vi "testLoop.vi"() -> ()   [LabVIEW 2018]
uses:
  02.Type Def's/All Motions.ctl
  02.Type Def's/NVH Mode Control 2.0.ctl
  05.UserVI's/type defs/EOL Global Digital Output Control.ctl
  05.UserVI's/type defs/EOL Global Digital Output Cluster Control.ctl
  <vilib>/Instr/_visa.llb/VISA Configure Serial Port (Instr).vi
  02.Type Def's/Pass Fail Control.ctl
  05.UserVI's/type defs/17x AP Data Type.ctl
  05.UserVI's/type defs/17x Audit Motion Data Seq Control.ctl
  02.Type Def's/EOL Motion Database Table.ctl
  02.Type Def's/lvdt name val pair.ctl
  02.Type Def's/NVH Digital Input.ctl
  02.Type Def's/EOL Switch Max Min Check Cluster.ctl
  02.Type Def's/EOL Switch Value Configuration Cluster.ctl
  02.Type Def's/All Switch Configuration Cluster.ctl
  02.Type Def's/station nvh config.ctl
  02.Type Def's/station DO map.ctl
  02.Type Def's/station rs232 port map.ctl
  02.Type Def's/station ethernet address map.ctl
  02.Type Def's/station paths.ctl
  05.UserVI's/type defs/17x Sunshade Limts Seq.ctl
  02.Type Def's/EOL Module Info Control.ctl
  02.Type Def's/EOL Save Module Test Data Control.ctl
  05.UserVI's/type defs/EOL Global Digital Input Control.ctl
  02.Type Def's/station DI map.ctl
  02.Type Def's/Screen Motion Data.ctl
  02.Type Def's/station motion data indicator.ctl
  02.Type Def's/station hmi.ctl
  02.Type Def's/individual station status.ctl
  02.Type Def's/control refs.ctl
  05.UserVI's/Lambda Power/power supply types.ctl
  <vilib>/Platform/dataskt.llb/DataSocket Reference Type.ctl
  05.UserVI's/type defs/plc path and tag.ctl
  02.Type Def's/station plc read boolean tags.ctl
  02.Type Def's/station plc write boolean tags.ctl
  02.Type Def's/station plc read string tags.ctl
  02.Type Def's/station plc write string tags.ctl
  02.Type Def's/iGPS float tags.ctl
  02.Type Def's/station plc read float tags.ctl
  02.Type Def's/plc comms params.ctl
  05.UserVI's/type defs/EOL LVDT's Check Controller.ctl
  05.UserVI's/LVDT's/lvdt precision.ctl
  05.UserVI's/sequence/type defs/Sequence Info.ctl
  02.Type Def's/sequence state.ctl
  05.UserVI's/type defs/EOL Motor Type.ctl
  05.UserVI's/type defs/RAP Signal Control.ctl
  05.UserVI's/type defs/Communication with Motors.ctl
  02.Type Def's/All Communication Types.ctl
  05.UserVI's/type defs/EOL Part Setup.ctl
  03.Inalfa LIN/LIN Device.ctl
  <vilib>/CMC.AME/Inalfa ADCS/Ctl'Def/ADCS_LIN info.ctl
  02.Type Def's/main state cluster.ctl
  C:/Program Files (x86)/National Instruments/LabVIEW 2018/vi.lib/CMC.AME/_Inalfa TS LIN_internal_deps/Interop.TSMasterAPI.dll
  Program Files (x86)/National Instruments/LabVIEW 2018/vi.lib/CMC.AME/_Inalfa TS LIN_internal_deps/Interop.TSMasterAPI.dll
  02.Type Def's/station LIN config.ctl
  02.Type Def's/misc station config.ctl
panel:
  out "Main State Cluster.Station Count":i32
  in  "Main State Cluster":T1 {"LIN INFO"."NAD" format="%.0x"; "LIN INFO"."ADCS LIN"."HW select" items=["NI-XNET", "NI-CAN"]; "LVDT Status"."LVDT's stored config"."Lower Limit" format="%.2f"; "LVDT Status"."LVDT's stored config"."Upper Limit" format="%.2f"; "PLC Comms"."PLC string write Tags"."error message 9"."DataSocket Reference"."OnStatusUpdated" format="%.0x"; "PLC Comms"."PLC string write Tags"."error message 9"."DataSocket Reference"."OnDataUpdated" format="%.0x"; "PLC Comms"."PLC string write Tags"."error message 8"."DataSocket Reference"."OnStatusUpdated" format="%.0x"; "PLC Comms"."PLC string write Tags"."error message 8"."DataSocket Reference"."OnDataUpdated" format="%.0x"; "PLC Comms"."PLC string write Tags"."error message 7"."DataSocket Reference"."OnStatusUpdated" format="%.0x"; "PLC Comms"."PLC string write Tags"."error message 7"."DataSocket Reference"."OnDataUpdated" format="%.0x"; "PLC Comms"."PLC string write Tags"."error message 6"."DataSocket Reference"."OnStatusUpdated" format="%.0x"; "PLC Comms"."PLC string write Tags"."error message 6"."DataSocket Reference"."OnDataUpdated" format="%.0x"; "PLC Comms"."PLC string write Tags"."error message 5"."DataSocket Reference"."OnStatusUpdated" format="%.0x"; "PLC Comms"."PLC string write Tags"."error message 5"."DataSocket Reference"."OnDataUpdated" format="%.0x"; "PLC Comms"."PLC string write Tags"."error message 4"."DataSocket Reference"."OnStatusUpdated" format="%.0x"; "PLC Comms"."PLC string write Tags"."error message 4"."DataSocket Reference"."OnDataUpdated" format="%.0x"; "PLC Comms"."PLC string write Tags"."error message 3"."DataSocket Reference"."OnStatusUpdated" format="%.0x"; "PLC Comms"."PLC string write Tags"."error message 3"."DataSocket Reference"."OnDataUpdated" format="%.0x"; "PLC Comms"."PLC string write Tags"."error message 2"."DataSocket Reference"."OnStatusUpdated" format="%.0x"; "PLC Comms"."PLC string write Tags"."error message 2"."DataSocket Reference"."OnDataUpdated" format="%.0x"; "PLC Comms"."PLC string write Tags"."error message 1"."DataSocket Reference"."OnStatusUpdated" format="%.0x"; "PLC Comms"."PLC string write Tags"."error message 1"."DataSocket Reference"."OnDataUpdated" format="%.0x"; "PLC Comms"."PLC string write Tags"."error message 0"."DataSocket Reference"."OnStatusUpdated" format="%.0x"; "PLC Comms"."PLC string write Tags"."error message 0"."DataSocket Reference"."OnDataUpdated" format="%.0x"; "PLC Comms"."PLC string write Tags"."barcode station error"."DataSocket Reference"."OnStatusUpdated" format="%.0x"; "PLC Comms"."PLC string write Tags"."barcode station error"."DataSocket Reference"."OnDataUpdated" format="%.0x"; "PLC Comms"."PLC string read Tags"."iGPS SN 9"."DataSocket Reference"."OnStatusUpdated" format="%.0x"; "PLC Comms"."PLC string read Tags"."iGPS SN 9"."DataSocket Reference"."OnDataUpdated" format="%.0x"; "PLC Comms"."PLC string read Tags"."iGPS SN 8"."DataSocket Reference"."OnStatusUpdated" format="%.0x"; "PLC Comms"."PLC string read Tags"."iGPS SN 8"."DataSocket Reference"."OnDataUpdated" format="%.0x"; "PLC Comms"."PLC string read Tags"."iGPS SN 7"."DataSocket Reference"."OnStatusUpdated" format="%.0x"; "PLC Comms"."PLC string read Tags"."iGPS SN 7"."DataSocket Reference"."OnDataUpdated" format="%.0x"; "PLC Comms"."PLC string read Tags"."iGPS SN 6"."DataSocket Reference"."OnStatusUpdated" format="%.0x"; "PLC Comms"."PLC string read Tags"."iGPS SN 6"."DataSocket Reference"."OnDataUpdated" format="%.0x"; "PLC Comms"."PLC string read Tags"."iGPS SN 5"."DataSocket Reference"."OnStatusUpdated" format="%.0x"; "PLC Comms"."PLC string read Tags"."iGPS SN 5"."DataSocket Reference"."OnDataUpdated" format="%.0x"; "PLC Comms"."PLC string read Tags"."iGPS SN 4"."DataSocket Reference"."OnStatusUpdated" format="%.0x"; "PLC Comms"."PLC string read Tags"."iGPS SN 4"."DataSocket Reference"."OnDataUpdated" format="%.0x"; "PLC Comms"."PLC string read Tags"."iGPS SN 3"."DataSocket Reference"."OnStatusUpdated" format="%.0x"; "PLC Comms"."PLC string read Tags"."iGPS SN 3"."DataSocket Reference"."OnDataUpdated" format="%.0x"; "PLC Comms"."PLC string read Tags"."iGPS SN 2"."DataSocket Reference"."OnStatusUpdated" format="%.0x"; "PLC Comms"."PLC string read Tags"."iGPS SN 2"."DataSocket Reference"."OnDataUpdated" format="%.0x"; "PLC Comms"."PLC string read Tags"."iGPS SN 1"."DataSocket Reference"."OnStatusUpdated" format="%.0x"; "PLC Comms"."PLC string read Tags"."iGPS SN 1"."DataSocket Reference"."OnDataUpdated" format="%.0x"; "PLC Comms"."PLC string read Tags"."iGPS SN 0"."DataSocket Reference"."OnStatusUpdated" format="%.0x"; "PLC Comms"."PLC string read Tags"."iGPS SN 0"."DataSocket Reference"."OnDataUpdated" format="%.0x"; "PLC Comms"."PLC string read Tags"."Manual Part History Number"."DataSocket Reference"."OnStatusUpdated" format="%.0x"; "PLC Comms"."PLC string read Tags"."Manual Part History Number"."DataSocket Reference"."OnDataUpdated" format="%.0x"; "PLC Comms"."PLC string read Tags"."Manual Customer Number"."DataSocket Reference"."OnStatusUpdated" format="%.0x"; "PLC Comms"."PLC string read Tags"."Manual Customer Number"."DataSocket Reference"."OnDataUpdated" format="%.0x"; "PLC Comms"."PLC string read Tags"."Manual Model Type"."DataSocket Reference"."OnStatusUpdated" format="%.0x"; "PLC Comms"."PLC string read Tags"."Manual Model Type"."DataSocket Reference"."OnDataUpdated" format="%.0x"; "PLC Comms"."PLC string read Tags"."Manual Shade Color"."DataSocket Reference"."OnStatusUpdated" format="%.0x"; "PLC Comms"."PLC string read Tags"."Manual Shade Color"."DataSocket Reference"."OnDataUpdated" format="%.0x"; "PLC Comms"."PLC string read Tags"."Manual Inalfa Part Number"."DataSocket Reference"."OnStatusUpdated" format="%.0x"; "PLC Comms"."PLC string read Tags"."Manual Inalfa Part Number"."DataSocket Reference"."OnDataUpdated" format="%.0x"; "PLC Comms"."PLC string read Tags"."Manual Serial Number"."DataSocket Reference"."OnStatusUpdated" format="%.0x"; "PLC Comms"."PLC string read Tags"."Manual Serial Number"."DataSocket Reference"."OnDataUpdated" format="%.0x"; "PLC Comms"."PLC string read Tags"."Shade 2 Barcode"."DataSocket Reference"."OnStatusUpdated" format="%.0x"; "PLC Comms"."PLC string read Tags"."Shade 2 Barcode"."DataSocket Reference"."OnDataUpdated" format="%.0x"; "PLC Comms"."PLC string read Tags"."Shade 1 Barcode"."DataSocket Reference"."OnStatusUpdated" format="%.0x"; "PLC Comms"."PLC string read Tags"."Shade 1 Barcode"."DataSocket Reference"."OnDataUpdated" format="%.0x"; "PLC Comms"."PLC string read Tags"."Part History Number"."DataSocket Reference"."OnStatusUpdated" format="%.0x"; "PLC Comms"."PLC string read Tags"."Part History Number"."DataSocket Reference"."OnDataUpdated" format="%.0x"; "PLC Comms"."PLC string read Tags"."Customer Number"."DataSocket Reference"."OnStatusUpdated" format="%.0x"; "PLC Comms"."PLC string read Tags"."Customer Number"."DataSocket Reference"."OnDataUpdated" format="%.0x"; "PLC Comms"."PLC string read Tags"."Model Type"."DataSocket Reference"."OnStatusUpdated" format="%.0x"; "PLC Comms"."PLC string read Tags"."Model Type"."DataSocket Reference"."OnDataUpdated" format="%.0x"; "PLC Comms"."PLC string read Tags"."Shade Color"."DataSocket Reference"."OnStatusUpdated" format="%.0x"; "PLC Comms"."PLC string read Tags"."Shade Color"."DataSocket Reference"."OnDataUpdated" format="%.0x"; "PLC Comms"."PLC string read Tags"."Inalfa Part Number"."DataSocket Reference"."OnStatusUpdated" format="%.0x"; "PLC Comms"."PLC string read Tags"."Inalfa Part Number"."DataSocket Reference"."OnDataUpdated" format="%.0x"; "PLC Comms"."PLC string read Tags"."Pallet Number"."DataSocket Reference"."OnStatusUpdated" format="%.0x"; "PLC Comms"."PLC string read Tags"."Pallet Number"."DataSocket Reference"."OnDataUpdated" format="%.0x"; "PLC Comms"."PLC string read Tags"."Serial Number"."DataSocket Reference"."OnStatusUpdated" format="%.0x"; "PLC Comms"."PLC string read Tags"."Serial Number"."DataSocket Reference"."OnDataUpdated" format="%.0x"; "PLC Comms"."PLC bool write Tags"."Move LVDT Adjust Station"."DataSocket Reference"."OnStatusUpdated" format="%.0x"; "PLC Comms"."PLC bool write Tags"."Move LVDT Adjust Station"."DataSocket Reference"."OnDataUpdated" format="%.0x"; "PLC Comms"."PLC bool write Tags"."AT set to Vent ATS Home Pos"."DataSocket Reference"."OnStatusUpdated" format="%.0x"; "PLC Comms"."PLC bool write Tags"."AT set to Vent ATS Home Pos"."DataSocket Reference"."OnDataUpdated" format="%.0x"; "PLC Comms"."PLC bool write Tags"."AT set to Vent ATS Test Pos"."DataSocket Reference"."OnStatusUpdated" format="%.0x"; "PLC Comms"."PLC bool write Tags"."AT set to Vent ATS Test Pos"."DataSocket Reference"."OnDataUpdated" format="%.0x"; "PLC Comms"."PLC bool write Tags"."Barcode02 OK"."DataSocket Reference"."OnStatusUpdated" format="%.0x"; "PLC Comms"."PLC bool write Tags"."Barcode02 OK"."DataSocket Reference"."OnDataUpdated" format="%.0x"; "PLC Comms"."PLC bool write Tags"."Barcode01 OK"."DataSocket Reference"."OnStatusUpdated" format="%.0x"; "PLC Comms"."PLC bool write Tags"."Barcode01 OK"."DataSocket Reference"."OnDataUpdated" format="%.0x"; "PLC Comms"."PLC bool write Tags"."AT set wand 02 home pos"."DataSocket Reference"."OnStatusUpdated" format="%.0x"; "PLC Comms"."PLC bool write Tags"."AT set wand 02 home pos"."DataSocket Reference"."OnDataUpdated" format="%.0x"; "PLC Comms"."PLC bool write Tags"."AT set sunshade 02 wand up"."DataSocket Reference"."OnStatusUpdated" format="%.0x"; "PLC Comms"."PLC bool write Tags"."AT set sunshade 02 wand up"."DataSocket Reference"."OnDataUpdated" format="%.0x"; "PLC Comms"."PLC bool write Tags"."NVH Operator Finish"."DataSocket Reference"."OnStatusUpdated" format="%.0x"; "PLC Comms"."PLC bool write Tags"."NVH Operator Finish"."DataSocket Reference"."OnDataUpdated" format="%.0x"; "PLC Comms"."PLC bool write Tags"."NVH Operator Glass Close Noise"."DataSocket Reference"."OnStatusUpdated" format="%.0x"; "PLC Comms"."PLC bool write Tags"."NVH Operator Glass Close Noise"."DataSocket Reference"."OnDataUpdated" format="%.0x"; "PLC Comms"."PLC bool write Tags"."NVH Operator Glass Open Noise"."DataSocket Reference"."OnStatusUpdated" format="%.0x"; "PLC Comms"."PLC bool write Tags"."NVH Operator Glass Open Noise"."DataSocket Reference"."OnDataUpdated" format="%.0x"; "PLC Comms"."PLC bool write Tags"."NVH Operator Sunshade Close Noise"."DataSocket Reference"."OnStatusUpdated" format="%.0x"; "PLC Comms"."PLC bool write Tags"."NVH Operator Sunshade Close Noise"."DataSocket Reference"."OnDataUpdated" format="%.0x"; "PLC Comms"."PLC bool write Tags"."NVH Operator Sunshade Open Noise"."DataSocket Reference"."OnStatusUpdated" format="%.0x"; "PLC Comms"."PLC bool write Tags"."NVH Operator Sunshade Open Noise"."DataSocket Reference"."OnDataUpdated" format="%.0x"; "PLC Comms"."PLC bool write Tags"."NVH Operator Vent Close Noise"."DataSocket Reference"."OnStatusUpdated" format="%.0x"; "PLC Comms"."PLC bool write Tags"."NVH Operator Vent Close Noise"."DataSocket Reference"."OnDataUpdated" format="%.0x"; "PLC Comms"."PLC bool write Tags"."NVH Operator Vent Open Noise"."DataSocket Reference"."OnStatusUpdated" format="%.0x"; "PLC Comms"."PLC bool write Tags"."NVH Operator Vent Open Noise"."DataSocket Reference"."OnDataUpdated" format="%.0x"; "PLC Comms"."PLC bool write Tags"."NVH Operator Check"."DataSocket Reference"."OnStatusUpdated" format="%.0x"; "PLC Comms"."PLC bool write Tags"."NVH Operator Check"."DataSocket Reference"."OnDataUpdated" format="%.0x"; "PLC Comms"."PLC bool write Tags"."NVH Operator Fail"."DataSocket Reference"."OnStatusUpdated" format="%.0x"; "PLC Comms"."PLC bool write Tags"."NVH Operator Fail"."DataSocket Reference"."OnDataUpdated" format="%.0x"; "PLC Comms"."PLC bool write Tags"."NVH Operator Pass"."DataSocket Reference"."OnStatusUpdated" format="%.0x"; "PLC Comms"."PLC bool write Tags"."NVH Operator Pass"."DataSocket Reference"."OnDataUpdated" format="%.0x"; "PLC Comms"."PLC bool write Tags"."NVH Operator Express Rollo Opened02"."DataSocket Reference"."OnStatusUpdated" format="%.0x"; "PLC Comms"."PLC bool write Tags"."NVH Operator Express Rollo Opened02"."DataSocket Reference"."OnDataUpdated" format="%.0x"; "PLC Comms"."PLC bool write Tags"."NVH Operator Express Rollo Closed01"."DataSocket Reference"."OnStatusUpdated" format="%.0x"; "PLC Comms"."PLC bool write Tags"."NVH Operator Express Rollo Closed01"."DataSocket Reference"."OnDataUpdated" format="%.0x"; "PLC Comms"."PLC bool write Tags"."NVH Operator Express Rollo Opened01"."DataSocket Reference"."OnStatusUpdated" format="%.0x"; "PLC Comms"."PLC bool write Tags"."NVH Operator Express Rollo Opened01"."DataSocket Reference"."OnDataUpdated" format="%.0x"; "PLC Comms"."PLC bool write Tags"."NVH Operator Express Glass Closed"."DataSocket Reference"."OnStatusUpdated" format="%.0x"; "PLC Comms"."PLC bool write Tags"."NVH Operator Express Glass Closed"."DataSocket Reference"."OnDataUpdated" format="%.0x"; "PLC Comms"."PLC bool write Tags"."NVH Operator Express Glass Opened"."DataSocket Reference"."OnStatusUpdated" format="%.0x"; "PLC Comms"."PLC bool write Tags"."NVH Operator Express Glass Opened"."DataSocket Reference"."OnDataUpdated" format="%.0x"; "PLC Comms"."PLC bool write Tags"."NVH Fail"."DataSocket Reference"."OnStatusUpdated" format="%.0x"; "PLC Comms"."PLC bool write Tags"."NVH Fail"."DataSocket Reference"."OnDataUpdated" format="%.0x"; "PLC Comms"."PLC bool write Tags"."NVH Pass"."DataSocket Reference"."OnStatusUpdated" format="%.0x"; "PLC Comms"."PLC bool write Tags"."NVH Pass"."DataSocket Reference"."OnDataUpdated" format="%.0x"; "PLC Comms"."PLC bool write Tags"."NVH SunRoof Stop"."DataSocket Reference"."OnStatusUpdated" format="%.0x"; "PLC Comms"."PLC bool write Tags"."NVH SunRoof Stop"."DataSocket Reference"."OnDataUpdated" format="%.0x"; "PLC Comms"."PLC bool write Tags"."NVH SunRoof Moving"."DataSocket Reference"."OnStatusUpdated" format="%.0x"; "PLC Comms"."PLC bool write Tags"."NVH SunRoof Moving"."DataSocket Reference"."OnDataUpdated" format="%.0x"; "PLC Comms"."PLC bool write Tags"."Extend Z LVDTS"."DataSocket Reference"."OnStatusUpdated" format="%.0x"; "PLC Comms"."PLC bool write Tags"."Extend Z LVDTS"."DataSocket Reference"."OnDataUpdated" format="%.0x"; "PLC Comms"."PLC bool write Tags"."Bad Frame Barcode"."DataSocket Reference"."OnStatusUpdated" format="%.0x"; "PLC Comms"."PLC bool write Tags"."Bad Frame Barcode"."DataSocket Reference"."OnDataUpdated" format="%.0x"; "PLC Comms"."PLC bool write Tags"."Good Frame Barcode"."DataSocket Reference"."OnStatusUpdated" format="%.0x"; "PLC Comms"."PLC bool write Tags"."Good Frame Barcode"."DataSocket Reference"."OnDataUpdated" format="%.0x"; "PLC Comms"."PLC bool write Tags"."AT VentPMACExtended"."DataSocket Reference"."OnStatusUpdated" format="%.0x"; "PLC Comms"."PLC bool write Tags"."AT VentPMACExtended"."DataSocket Reference"."OnDataUpdated" format="%.0x"; "PLC Comms"."PLC bool write Tags"."AT VentPMACHome"."DataSocket Reference"."OnStatusUpdated" format="%.0x"; "PLC Comms"."PLC bool write Tags"."AT VentPMACHome"."DataSocket Reference"."OnDataUpdated" format="%.0x"; "PLC Comms"."PLC bool write Tags"."control slide stop"."DataSocket Reference"."OnStatusUpdated" format="%.0x"; "PLC Comms"."PLC bool write Tags"."control slide stop"."DataSocket Reference"."OnDataUpdated" format="%.0x"; "PLC Comms"."PLC bool write Tags"."control slide start"."DataSocket Reference"."OnStatusUpdated" format="%.0x"; "PLC Comms"."PLC bool write Tags"."control slide start"."DataSocket Reference"."OnDataUpdated" format="%.0x"; "PLC Comms"."PLC bool write Tags"."ss servo close"."DataSocket Reference"."OnStatusUpdated" format="%.0x"; "PLC Comms"."PLC bool write Tags"."ss servo close"."DataSocket Reference"."OnDataUpdated" format="%.0x"; "PLC Comms"."PLC bool write Tags"."ss servo open"."DataSocket Reference"."OnStatusUpdated" format="%.0x"; "PLC Comms"."PLC bool write Tags"."ss servo open"."DataSocket Reference"."OnDataUpdated" format="%.0x"; "PLC Comms"."PLC bool write Tags"."Extend LVDT's"."DataSocket Reference"."OnStatusUpdated" format="%.0x"; "PLC Comms"."PLC bool write Tags"."Extend LVDT's"."DataSocket Reference"."OnDataUpdated" format="%.0x"; "PLC Comms"."PLC bool write Tags"."Retract LVDT's"."DataSocket Reference"."OnStatusUpdated" format="%.0x"; "PLC Comms"."PLC bool write Tags"."Retract LVDT's"."DataSocket Reference"."OnDataUpdated" format="%.0x"; "PLC Comms"."PLC bool write Tags"."Test Started"."DataSocket Reference"."OnStatusUpdated" format="%.0x"; "PLC Comms"."PLC bool write Tags"."Test Started"."DataSocket Reference"."OnDataUpdated" format="%.0x"; "PLC Comms"."PLC bool write Tags"."Test Complete Fail"."DataSocket Reference"."OnStatusUpdated" format="%.0x"; "PLC Comms"."PLC bool write Tags"."Test Complete Fail"."DataSocket Reference"."OnDataUpdated" format="%.0x"; "PLC Comms"."PLC bool write Tags"."Test Complete Pass"."DataSocket Reference"."OnStatusUpdated" format="%.0x"; "PLC Comms"."PLC bool write Tags"."Test Complete Pass"."DataSocket Reference"."OnDataUpdated" format="%.0x"; "PLC Comms"."PLC bool write Tags"."AT set wand home pos"."DataSocket Reference"."OnStatusUpdated" format="%.0x"; "PLC Comms"."PLC bool write Tags"."AT set wand home pos"."DataSocket Reference"."OnDataUpdated" format="%.0x"; "PLC Comms"."PLC bool write Tags"."AT set sunshade wand lower"."DataSocket Reference"."OnStatusUpdated" format="%.0x"; "PLC Comms"."PLC bool write Tags"."AT set sunshade wand lower"."DataSocket Reference"."OnDataUpdated" format="%.0x"; "PLC Comms"."PLC bool write Tags"."AT set glass wand lower"."DataSocket Reference"."OnStatusUpdated" format="%.0x"; "PLC Comms"."PLC bool write Tags"."AT set glass wand lower"."DataSocket Reference"."OnDataUpdated" format="%.0x"; "PLC Comms"."PLC boolean read Tags"."Finish Adjust LVDT"."DataSocket Reference"."OnStatusUpdated" format="%.0x"; "PLC Comms"."PLC boolean read Tags"."Finish Adjust LVDT"."DataSocket Reference"."OnDataUpdated" format="%.0x"; "PLC Comms"."PLC boolean read Tags"."Start Adjust LVDT"."DataSocket Reference"."OnStatusUpdated" format="%.0x"; "PLC Comms"."PLC boolean read Tags"."Start Adjust LVDT"."DataSocket Reference"."OnDataUpdated" format="%.0x"; "PLC Comms"."PLC boolean read Tags"."AT at vent ATS Home pos"."DataSocket Reference"."OnStatusUpdated" format="%.0x"; "PLC Comms"."PLC boolean read Tags"."AT at vent ATS Home pos"."DataSocket Reference"."OnDataUpdated" format="%.0x"; "PLC Comms"."PLC boolean read Tags"."AT at vent ATS test pos"."DataSocket Reference"."OnStatusUpdated" format="%.0x"; "PLC Comms"."PLC boolean read Tags"."AT at vent ATS test pos"."DataSocket Reference"."OnDataUpdated" format="%.0x"; "PLC Comms"."PLC boolean read Tags"."NVH Operator Re-do"."DataSocket Reference"."OnStatusUpdated" format="%.0x"; "PLC Comms"."PLC boolean read Tags"."NVH Operator Re-do"."DataSocket Reference"."OnDataUpdated" format="%.0x"; "PLC Comms"."PLC boolean read Tags"."NVH Operator Express Glass Vent Close"."DataSocket Reference"."OnStatusUpdated" format="%.0x"; "PLC Comms"."PLC boolean read Tags"."NVH Operator Express Glass Vent Close"."DataSocket Reference"."OnDataUpdated" format="%.0x"; "PLC Comms"."PLC boolean read Tags"."NVH Operator Express Glass vent Open"."DataSocket Reference"."OnStatusUpdated" format="%.0x"; "PLC Comms"."PLC boolean read Tags"."NVH Operator Express Glass vent Open"."DataSocket Reference"."OnDataUpdated" format="%.0x"; "PLC Comms"."PLC boolean read Tags"."windproof position"."DataSocket Reference"."OnStatusUpdated" format="%.0x"; "PLC Comms"."PLC boolean read Tags"."windproof position"."DataSocket Reference"."OnDataUpdated" format="%.0x"; "PLC Comms"."PLC boolean read Tags"."AT in wand 02 home pos"."DataSocket Reference"."OnStatusUpdated" format="%.0x"; "PLC Comms"."PLC boolean read Tags"."AT in wand 02 home pos"."DataSocket Reference"."OnDataUpdated" format="%.0x"; "PLC Comms"."PLC boolean read Tags"."AT in sunshad 02 wand up pos"."DataSocket Reference"."OnStatusUpdated" format="%.0x"; "PLC Comms"."PLC boolean read Tags"."AT in sunshad 02 wand up pos"."DataSocket Reference"."OnDataUpdated" format="%.0x"; "PLC Comms"."PLC boolean read Tags"."AT shade 02 position"."DataSocket Reference"."OnStatusUpdated" format="%.0x"; "PLC Comms"."PLC boolean read Tags"."AT shade 02 position"."DataSocket Reference"."OnDataUpdated" format="%.0x"; "PLC Comms"."PLC boolean read Tags"."NVH Operator Check"."DataSocket Reference"."OnStatusUpdated" format="%.0x"; "PLC Comms"."PLC boolean read Tags"."NVH Operator Check"."DataSocket Reference"."OnDataUpdated" format="%.0x"; "PLC Comms"."PLC boolean read Tags"."NVH Operator Finish"."DataSocket Reference"."OnStatusUpdated" format="%.0x"; "PLC Comms"."PLC boolean read Tags"."NVH Operator Finish"."DataSocket Reference"."OnDataUpdated" format="%.0x"; "PLC Comms"."PLC boolean read Tags"."NVH Operator Glass Close Noise"."DataSocket Reference"."OnStatusUpdated" format="%.0x"; "PLC Comms"."PLC boolean read Tags"."NVH Operator Glass Close Noise"."DataSocket Reference"."OnDataUpdated" format="%.0x"; "PLC Comms"."PLC boolean read Tags"."NVH Operator Glass Open Noise"."DataSocket Reference"."OnStatusUpdated" format="%.0x"; "PLC Comms"."PLC boolean read Tags"."NVH Operator Glass Open Noise"."DataSocket Reference"."OnDataUpdated" format="%.0x"; "PLC Comms"."PLC boolean read Tags"."NVH Operator Sunshade Close Noise"."DataSocket Reference"."OnStatusUpdated" format="%.0x"; "PLC Comms"."PLC boolean read Tags"."NVH Operator Sunshade Close Noise"."DataSocket Reference"."OnDataUpdated" format="%.0x"; "PLC Comms"."PLC boolean read Tags"."NVH Operator Sunshade Open Noise"."DataSocket Reference"."OnStatusUpdated" format="%.0x"; "PLC Comms"."PLC boolean read Tags"."NVH Operator Sunshade Open Noise"."DataSocket Reference"."OnDataUpdated" format="%.0x"; "PLC Comms"."PLC boolean read Tags"."NVH Operator Vent Close Noise"."DataSocket Reference"."OnStatusUpdated" format="%.0x"; "PLC Comms"."PLC boolean read Tags"."NVH Operator Vent Close Noise"."DataSocket Reference"."OnDataUpdated" format="%.0x"; "PLC Comms"."PLC boolean read Tags"."NVH Operator Vent Open Noise"."DataSocket Reference"."OnStatusUpdated" format="%.0x"; "PLC Comms"."PLC boolean read Tags"."NVH Operator Vent Open Noise"."DataSocket Reference"."OnDataUpdated" format="%.0x"; "PLC Comms"."PLC boolean read Tags"."NVH Operator Express Rollo Close02"."DataSocket Reference"."OnStatusUpdated" format="%.0x"; "PLC Comms"."PLC boolean read Tags"."NVH Operator Express Rollo Close02"."DataSocket Reference"."OnDataUpdated" format="%.0x"; "PLC Comms"."PLC boolean read Tags"."NVH Operator Express Rollo Open02"."DataSocket Reference"."OnStatusUpdated" format="%.0x"; "PLC Comms"."PLC boolean read Tags"."NVH Operator Express Rollo Open02"."DataSocket Reference"."OnDataUpdated" format="%.0x"; "PLC Comms"."PLC boolean read Tags"."NVH Operator Express Rollo Close01"."DataSocket Reference"."OnStatusUpdated" format="%.0x"; "PLC Comms"."PLC boolean read Tags"."NVH Operator Express Rollo Close01"."DataSocket Reference"."OnDataUpdated" format="%.0x"; "PLC Comms"."PLC boolean read Tags"."NVH Operator Express Rollo Open01"."DataSocket Reference"."OnStatusUpdated" format="%.0x"; "PLC Comms"."PLC boolean read Tags"."NVH Operator Express Rollo Open01"."DataSocket Reference"."OnDataUpdated" format="%.0x"; "PLC Comms"."PLC boolean read Tags"."NVH Operator Express Glass Close"."DataSocket Reference"."OnStatusUpdated" format="%.0x"; "PLC Comms"."PLC boolean read Tags"."NVH Operator Express Glass Close"."DataSocket Reference"."OnDataUpdated" format="%.0x"; "PLC Comms"."PLC boolean read Tags"."NVH Operator Express Glass Open"."DataSocket Reference"."OnStatusUpdated" format="%.0x"; "PLC Comms"."PLC boolean read Tags"."NVH Operator Express Glass Open"."DataSocket Reference"."OnDataUpdated" format="%.0x"; "PLC Comms"."PLC boolean read Tags"."NVH Operator Fail"."DataSocket Reference"."OnStatusUpdated" format="%.0x"; "PLC Comms"."PLC boolean read Tags"."NVH Operator Fail"."DataSocket Reference"."OnDataUpdated" format="%.0x"; "PLC Comms"."PLC boolean read Tags"."NVH Operator Pass"."DataSocket Reference"."OnStatusUpdated" format="%.0x"; "PLC Comms"."PLC boolean read Tags"."NVH Operator Pass"."DataSocket Reference"."OnDataUpdated" format="%.0x"; "PLC Comms"."PLC boolean read Tags"."Z LVDTs Extended"."DataSocket Reference"."OnStatusUpdated" format="%.0x"; "PLC Comms"."PLC boolean read Tags"."Z LVDTs Extended"."DataSocket Reference"."OnDataUpdated" format="%.0x"; "PLC Comms"."PLC boolean read Tags"."iGPS Pass 9"."DataSocket Reference"."OnStatusUpdated" format="%.0x"; "PLC Comms"."PLC boolean read Tags"."iGPS Pass 9"."DataSocket Reference"."OnDataUpdated" format="%.0x"; "PLC Comms"."PLC boolean read Tags"."iGPS Pass 8"."DataSocket Reference"."OnStatusUpdated" format="%.0x"; "PLC Comms"."PLC boolean read Tags"."iGPS Pass 8"."DataSocket Reference"."OnDataUpdated" format="%.0x"; "PLC Comms"."PLC boolean read Tags"."iGPS Pass 7"."DataSocket Reference"."OnStatusUpdated" format="%.0x"; "PLC Comms"."PLC boolean read Tags"."iGPS Pass 7"."DataSocket Reference"."OnDataUpdated" format="%.0x"; "PLC Comms"."PLC boolean read Tags"."iGPS Pass 6"."DataSocket Reference"."OnStatusUpdated" format="%.0x"; "PLC Comms"."PLC boolean read Tags"."iGPS Pass 6"."DataSocket Reference"."OnDataUpdated" format="%.0x"; "PLC Comms"."PLC boolean read Tags"."iGPS Pass 5"."DataSocket Reference"."OnStatusUpdated" format="%.0x"; "PLC Comms"."PLC boolean read Tags"."iGPS Pass 5"."DataSocket Reference"."OnDataUpdated" format="%.0x"; "PLC Comms"."PLC boolean read Tags"."iGPS Pass 4"."DataSocket Reference"."OnStatusUpdated" format="%.0x"; "PLC Comms"."PLC boolean read Tags"."iGPS Pass 4"."DataSocket Reference"."OnDataUpdated" format="%.0x"; "PLC Comms"."PLC boolean read Tags"."iGPS Pass 3"."DataSocket Reference"."OnStatusUpdated" format="%.0x"; "PLC Comms"."PLC boolean read Tags"."iGPS Pass 3"."DataSocket Reference"."OnDataUpdated" format="%.0x"; "PLC Comms"."PLC boolean read Tags"."iGPS Pass 2"."DataSocket Reference"."OnStatusUpdated" format="%.0x"; "PLC Comms"."PLC boolean read Tags"."iGPS Pass 2"."DataSocket Reference"."OnDataUpdated" format="%.0x"; "PLC Comms"."PLC boolean read Tags"."iGPS Pass 1"."DataSocket Reference"."OnStatusUpdated" format="%.0x"; "PLC Comms"."PLC boolean read Tags"."iGPS Pass 1"."DataSocket Reference"."OnDataUpdated" format="%.0x"; "PLC Comms"."PLC boolean read Tags"."iGPS Pass 0"."DataSocket Reference"."OnStatusUpdated" format="%.0x"; "PLC Comms"."PLC boolean read Tags"."iGPS Pass 0"."DataSocket Reference"."OnDataUpdated" format="%.0x"; "PLC Comms"."PLC boolean read Tags"."Check Frame Barcode"."DataSocket Reference"."OnStatusUpdated" format="%.0x"; "PLC Comms"."PLC boolean read Tags"."Check Frame Barcode"."DataSocket Reference"."OnDataUpdated" format="%.0x"; "PLC Comms"."PLC boolean read Tags"."SS Barcode Scanner Bypassed"."DataSocket Reference"."OnStatusUpdated" format="%.0x"; "PLC Comms"."PLC boolean read Tags"."SS Barcode Scanner Bypassed"."DataSocket Reference"."OnDataUpdated" format="%.0x"; "PLC Comms"."PLC boolean read Tags"."AT VentPMACisExtend"."DataSocket Reference"."OnStatusUpdated" format="%.0x"; "PLC Comms"."PLC boolean read Tags"."AT VentPMACisExtend"."DataSocket Reference"."OnDataUpdated" format="%.0x"; "PLC Comms"."PLC boolean read Tags"."AT VentPMACatHome"."DataSocket Reference"."OnStatusUpdated" format="%.0x"; "PLC Comms"."PLC boolean read Tags"."AT VentPMACatHome"."DataSocket Reference"."OnDataUpdated" format="%.0x"; "PLC Comms"."PLC boolean read Tags"."wind deflector low speed pos"."DataSocket Reference"."OnStatusUpdated" format="%.0x"; "PLC Comms"."PLC boolean read Tags"."wind deflector low speed pos"."DataSocket Reference"."OnDataUpdated" format="%.0x"; "PLC Comms"."PLC boolean read Tags"."wind deflector high speed pos"."DataSocket Reference"."OnStatusUpdated" format="%.0x"; "PLC Comms"."PLC boolean read Tags"."wind deflector high speed pos"."DataSocket Reference"."OnDataUpdated" format="%.0x"; "PLC Comms"."PLC boolean read Tags"."control slide right over stroke"."DataSocket Reference"."OnStatusUpdated" format="%.0x"; "PLC Comms"."PLC boolean read Tags"."control slide right over stroke"."DataSocket Reference"."OnDataUpdated" format="%.0x"; "PLC Comms"."PLC boolean read Tags"."control slide right good"."DataSocket Reference"."OnStatusUpdated" format="%.0x"; "PLC Comms"."PLC boolean read Tags"."control slide right good"."DataSocket Reference"."OnDataUpdated" format="%.0x"; "PLC Comms"."PLC boolean read Tags"."control slide left over stroke"."DataSocket Reference"."OnStatusUpdated" format="%.0x"; "PLC Comms"."PLC boolean read Tags"."control slide left over stroke"."DataSocket Reference"."OnDataUpdated" format="%.0x"; "PLC Comms"."PLC boolean read Tags"."control slide left good"."DataSocket Reference"."OnStatusUpdated" format="%.0x"; "PLC Comms"."PLC boolean read Tags"."control slide left good"."DataSocket Reference"."OnDataUpdated" format="%.0x"; "PLC Comms"."PLC boolean read Tags"."control slide at home"."DataSocket Reference"."OnStatusUpdated" format="%.0x"; "PLC Comms"."PLC boolean read Tags"."control slide at home"."DataSocket Reference"."OnDataUpdated" format="%.0x"; "PLC Comms"."PLC boolean read Tags"."ss servo closing"."DataSocket Reference"."OnStatusUpdated" format="%.0x"; "PLC Comms"."PLC boolean read Tags"."ss servo closing"."DataSocket Reference"."OnDataUpdated" format="%.0x"; "PLC Comms"."PLC boolean read Tags"."ss servo opening"."DataSocket Reference"."OnStatusUpdated" format="%.0x"; "PLC Comms"."PLC boolean read Tags"."ss servo opening"."DataSocket Reference"."OnDataUpdated" format="%.0x"; "PLC Comms"."PLC boolean read Tags"."ss servo at close"."DataSocket Reference"."OnStatusUpdated" format="%.0x"; "PLC Comms"."PLC boolean read Tags"."ss servo at close"."DataSocket Reference"."OnDataUpdated" format="%.0x"; "PLC Comms"."PLC boolean read Tags"."ss servo at open"."DataSocket Reference"."OnStatusUpdated" format="%.0x"; "PLC Comms"."PLC boolean read Tags"."ss servo at open"."DataSocket Reference"."OnDataUpdated" format="%.0x"; "PLC Comms"."PLC boolean read Tags"."manual barcode print"."DataSocket Reference"."OnStatusUpdated" format="%.0x"; "PLC Comms"."PLC boolean read Tags"."manual barcode print"."DataSocket Reference"."OnDataUpdated" format="%.0x"; "PLC Comms"."PLC boolean read Tags"."LVDT's Retracted"."DataSocket Reference"."OnStatusUpdated" format="%.0x"; "PLC Comms"."PLC boolean read Tags"."LVDT's Retracted"."DataSocket Reference"."OnDataUpdated" format="%.0x"; "PLC Comms"."PLC boolean read Tags"."abort"."DataSocket Reference"."OnStatusUpdated" format="%.0x"; "PLC Comms"."PLC boolean read Tags"."abort"."DataSocket Reference"."OnDataUpdated" format="%.0x"; "PLC Comms"."PLC boolean read Tags"."start"."DataSocket Reference"."OnStatusUpdated" format="%.0x"; "PLC Comms"."PLC boolean read Tags"."start"."DataSocket Reference"."OnDataUpdated" format="%.0x"; "PLC Comms"."PLC boolean read Tags"."bolt check 21"."DataSocket Reference"."OnStatusUpdated" format="%.0x"; "PLC Comms"."PLC boolean read Tags"."bolt check 21"."DataSocket Reference"."OnDataUpdated" format="%.0x"; "PLC Comms"."PLC boolean read Tags"."bolt check 20"."DataSocket Reference"."OnStatusUpdated" format="%.0x"; "PLC Comms"."PLC boolean read Tags"."bolt check 20"."DataSocket Reference"."OnDataUpdated" format="%.0x"; "PLC Comms"."PLC boolean read Tags"."bolt check 19"."DataSocket Reference"."OnStatusUpdated" format="%.0x"; "PLC Comms"."PLC boolean read Tags"."bolt check 19"."DataSocket Reference"."OnDataUpdated" format="%.0x"; "PLC Comms"."PLC boolean read Tags"."bolt check 18"."DataSocket Reference"."OnStatusUpdated" format="%.0x"; "PLC Comms"."PLC boolean read Tags"."bolt check 18"."DataSocket Reference"."OnDataUpdated" format="%.0x"; "PLC Comms"."PLC boolean read Tags"."bolt check 17"."DataSocket Reference"."OnStatusUpdated" format="%.0x"; "PLC Comms"."PLC boolean read Tags"."bolt check 17"."DataSocket Reference"."OnDataUpdated" format="%.0x"; "PLC Comms"."PLC boolean read Tags"."bolt check 16"."DataSocket Reference"."OnStatusUpdated" format="%.0x"; "PLC Comms"."PLC boolean read Tags"."bolt check 16"."DataSocket Reference"."OnDataUpdated" format="%.0x"; "PLC Comms"."PLC boolean read Tags"."bolt check 15"."DataSocket Reference"."OnStatusUpdated" format="%.0x"; "PLC Comms"."PLC boolean read Tags"."bolt check 15"."DataSocket Reference"."OnDataUpdated" format="%.0x"; "PLC Comms"."PLC boolean read Tags"."bolt check 14"."DataSocket Reference"."OnStatusUpdated" format="%.0x"; "PLC Comms"."PLC boolean read Tags"."bolt check 14"."DataSocket Reference"."OnDataUpdated" format="%.0x"; "PLC Comms"."PLC boolean read Tags"."bolt check 13"."DataSocket Reference"."OnStatusUpdated" format="%.0x"; "PLC Comms"."PLC boolean read Tags"."bolt check 13"."DataSocket Reference"."OnDataUpdated" format="%.0x"; "PLC Comms"."PLC boolean read Tags"."bolt check 12"."DataSocket Reference"."OnStatusUpdated" format="%.0x"; "PLC Comms"."PLC boolean read Tags"."bolt check 12"."DataSocket Reference"."OnDataUpdated" format="%.0x"; "PLC Comms"."PLC boolean read Tags"."bolt check 11"."DataSocket Reference"."OnStatusUpdated" format="%.0x"; "PLC Comms"."PLC boolean read Tags"."bolt check 11"."DataSocket Reference"."OnDataUpdated" format="%.0x"; "PLC Comms"."PLC boolean read Tags"."bolt check 10"."DataSocket Reference"."OnStatusUpdated" format="%.0x"; "PLC Comms"."PLC boolean read Tags"."bolt check 10"."DataSocket Reference"."OnDataUpdated" format="%.0x"; "PLC Comms"."PLC boolean read Tags"."bolt check 9"."DataSocket Reference"."OnStatusUpdated" format="%.0x"; "PLC Comms"."PLC boolean read Tags"."bolt check 9"."DataSocket Reference"."OnDataUpdated" format="%.0x"; "PLC Comms"."PLC boolean read Tags"."bolt check 8"."DataSocket Reference"."OnStatusUpdated" format="%.0x"; "PLC Comms"."PLC boolean read Tags"."bolt check 8"."DataSocket Reference"."OnDataUpdated" format="%.0x"; "PLC Comms"."PLC boolean read Tags"."bolt check 7"."DataSocket Reference"."OnStatusUpdated" format="%.0x"; "PLC Comms"."PLC boolean read Tags"."bolt check 7"."DataSocket Reference"."OnDataUpdated" format="%.0x"; "PLC Comms"."PLC boolean read Tags"."bolt check 6"."DataSocket Reference"."OnStatusUpdated" format="%.0x"; "PLC Comms"."PLC boolean read Tags"."bolt check 6"."DataSocket Reference"."OnDataUpdated" format="%.0x"; "PLC Comms"."PLC boolean read Tags"."bolt check 5"."DataSocket Reference"."OnStatusUpdated" format="%.0x"; "PLC Comms"."PLC boolean read Tags"."bolt check 5"."DataSocket Reference"."OnDataUpdated" format="%.0x"; "PLC Comms"."PLC boolean read Tags"."bolt check 4"."DataSocket Reference"."OnStatusUpdated" format="%.0x"; "PLC Comms"."PLC boolean read Tags"."bolt check 4"."DataSocket Reference"."OnDataUpdated" format="%.0x"; "PLC Comms"."PLC boolean read Tags"."bolt check 3"."DataSocket Reference"."OnStatusUpdated" format="%.0x"; "PLC Comms"."PLC boolean read Tags"."bolt check 3"."DataSocket Reference"."OnDataUpdated" format="%.0x"; "PLC Comms"."PLC boolean read Tags"."bolt check 2"."DataSocket Reference"."OnStatusUpdated" format="%.0x"; "PLC Comms"."PLC boolean read Tags"."bolt check 2"."DataSocket Reference"."OnDataUpdated" format="%.0x"; "PLC Comms"."PLC boolean read Tags"."bolt check 1"."DataSocket Reference"."OnStatusUpdated" format="%.0x"; "PLC Comms"."PLC boolean read Tags"."bolt check 1"."DataSocket Reference"."OnDataUpdated" format="%.0x"; "PLC Comms"."PLC boolean read Tags"."FB light block present"."DataSocket Reference"."OnStatusUpdated" format="%.0x"; "PLC Comms"."PLC boolean read Tags"."FB light block present"."DataSocket Reference"."OnDataUpdated" format="%.0x"; "PLC Comms"."PLC boolean read Tags"."audit gap hider present RH"."DataSocket Reference"."OnStatusUpdated" format="%.0x"; "PLC Comms"."PLC boolean read Tags"."audit gap hider present RH"."DataSocket Reference"."OnDataUpdated" format="%.0x"; "PLC Comms"."PLC boolean read Tags"."audit gap hider present LH"."DataSocket Reference"."OnStatusUpdated" format="%.0x"; "PLC Comms"."PLC boolean read Tags"."audit gap hider present LH"."DataSocket Reference"."OnDataUpdated" format="%.0x"; "PLC Comms"."PLC boolean read Tags"."motor foam present RH"."DataSocket Reference"."OnStatusUpdated" format="%.0x"; "PLC Comms"."PLC boolean read Tags"."motor foam present RH"."DataSocket Reference"."OnDataUpdated" format="%.0x"; "PLC Comms"."PLC boolean read Tags"."motor foam present LH"."DataSocket Reference"."OnStatusUpdated" format="%.0x"; "PLC Comms"."PLC boolean read Tags"."motor foam present LH"."DataSocket Reference"."OnDataUpdated" format="%.0x"; "PLC Comms"."PLC boolean read Tags"."LVDT's Extended"."DataSocket Reference"."OnStatusUpdated" format="%.0x"; "PLC Comms"."PLC boolean read Tags"."LVDT's Extended"."DataSocket Reference"."OnDataUpdated" format="%.0x"; "PLC Comms"."PLC boolean read Tags"."AT in wand home pos"."DataSocket Reference"."OnStatusUpdated" format="%.0x"; "PLC Comms"."PLC boolean read Tags"."AT in wand home pos"."DataSocket Reference"."OnDataUpdated" format="%.0x"; "PLC Comms"."PLC boolean read Tags"."AT in sunshad wand lower pos"."DataSocket Reference"."OnStatusUpdated" format="%.0x"; "PLC Comms"."PLC boolean read Tags"."AT in sunshad wand lower pos"."DataSocket Reference"."OnDataUpdated" format="%.0x"; "PLC Comms"."PLC boolean read Tags"."AT in glass wand lower pos"."DataSocket Reference"."OnStatusUpdated" format="%.0x"; "PLC Comms"."PLC boolean read Tags"."AT in glass wand lower pos"."DataSocket Reference"."OnDataUpdated" format="%.0x"; "PLC Comms"."PLC boolean read Tags"."AT shade position"."DataSocket Reference"."OnStatusUpdated" format="%.0x"; "PLC Comms"."PLC boolean read Tags"."AT shade position"."DataSocket Reference"."OnDataUpdated" format="%.0x"; "PLC Comms"."PLC boolean read Tags"."AT glass position"."DataSocket Reference"."OnStatusUpdated" format="%.0x"; "PLC Comms"."PLC boolean read Tags"."AT glass position"."DataSocket Reference"."OnDataUpdated" format="%.0x"; "Store Data"."Sun Shade Open Force Limits"."Variance" format="%.2g"; "Store Data"."Sun Shade Open Force Limits"."Truncation End" format="%.2g"; "Store Data"."Sun Shade Open Force Limits"."Truncation Start" format="%.2g"; "Store Data"."Sun Shade Open Force Limits"."Avg Max" format="%.2g"; "Store Data"."Sun Shade Open Force Limits"."Avg Min" format="%.2g"; "Store Data"."Sun Shade Open Force Limits"."Overall Max" format="%.2g"; "Store Data"."Sun Shade Open Force Limits"."Overall Min" format="%.2g"; "Store Data"."Sun Shade Close Force Limits"."Variance" format="%.2g"; "Store Data"."Sun Shade Close Force Limits"."Truncation End" format="%.2g"; "Store Data"."Sun Shade Close Force Limits"."Truncation Start" format="%.2g"; "Store Data"."Sun Shade Close Force Limits"."Avg Max" format="%.2g"; "Store Data"."Sun Shade Close Force Limits"."Avg Min" format="%.2g"; "Store Data"."Sun Shade Close Force Limits"."Overall Max" format="%.2g"; "Store Data"."Sun Shade Close Force Limits"."Overall Min" format="%.2g"}
  # "start/abort only used by barcode instance, since there are discrete signals for this in the other stations."
  # "Sunroof Barcode"
  # "Pallet Number"
  # "Part Type"
  # "Application Status"
  # "Current Step"
  # "Cycle Time"
  # "Pass / Fail"
  # "Shade Close"
  # "Actual Data"
  # "Limits"
  # "Avg Current"
  # "Run Time"
  # "Speed"
  # "Noise Test"
  # "Position"
  # "Shade Open"
  # "Actual Data"
  # "Limits"
  # "Avg Current"
  # "Run Time"
  # "Speed"
  # "Noise Test"
  # "Position"
  # "Vent Close"
  # "Actual Data"
  # "Limits"
  # "Avg Current"
  # "Run Time"
  # "Speed"
  # "Noise Test"
  # "Position"
  # "Vent Open"
  # "Actual Data"
  # "Limits"
  # "Avg Current"
  # "Run Time"
  # "Speed"
  # "Noise Test"
  # "Position"
  # "Slide Close"
  # "Actual Data"
  # "Limits"
  # "Avg Current"
  # "Run Time"
  # "Speed"
  # "Noise Test"
  # "Position"
  # "Slide Open"
  # "Actual Data"
  # "Limits"
  # "Avg Current"
  # "Run Time"
  # "Speed"
  # "Noise Test"
  # "Position"
  # "Min"
  # "N"
  # "Min"
  # "Start"
  # "N"
  # "Max"
  # "N"
  # "Max"
  # "N"
  # "End"
  # "Min"
  # "N"
  # "Min"
  # "Start"
  # "N"
  # "Max"
  # "N"
  # "Max"
  # "N"
  # "End"
  # "Min"
  # "Max"
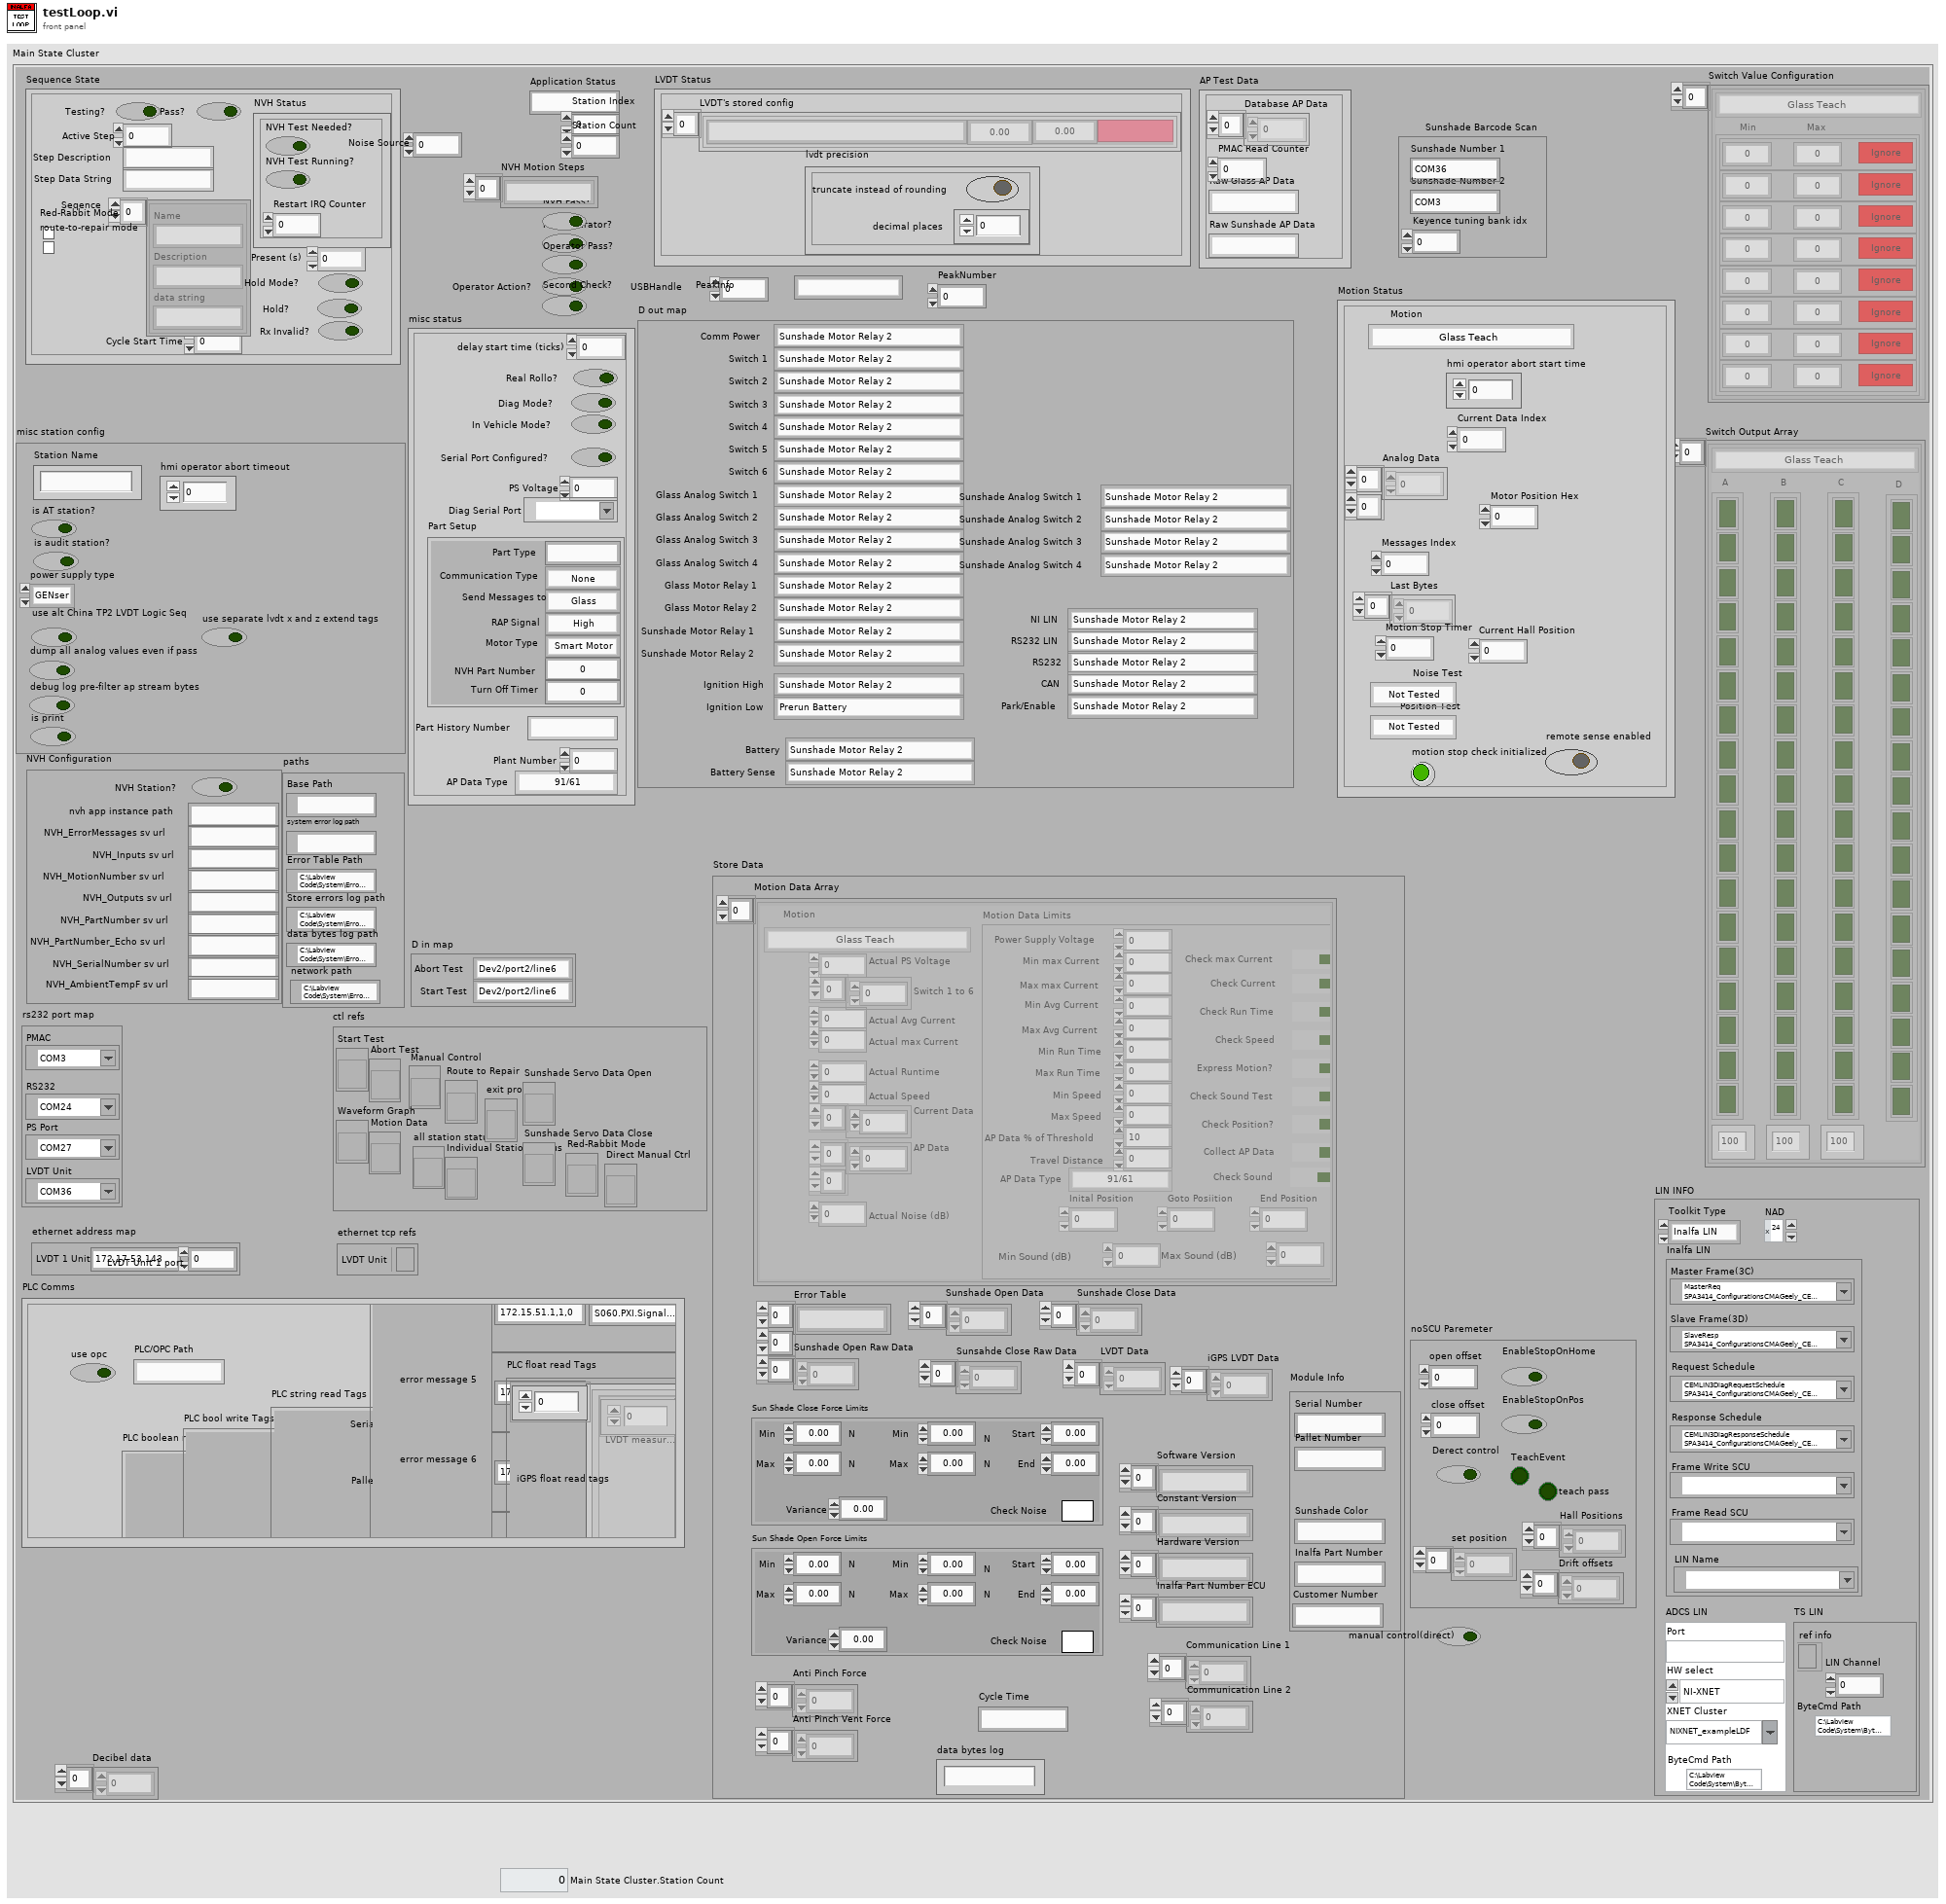
[diagram p1: front panel]
types:
  T1 = typedef "main state cluster.ctl" = cluster{"Application Status":string, "Switch Output Array":T2[], "Switch Value Configuration":T4[], "NVH Configuration":T6, "D out map":T7, "rs232 port map":T10, "ethernet address map":T11, "paths":T12, "Station Index":i32, "Station Count":i32, "Store Data":T13, "D in map":T19, "ctl refs":T21, "misc station config":T22, "ethernet tcp refs":cluster{"LVDT Unit":refnum<k5>}, "PLC Comms":T24, "Sunshade Barcode Scan":cluster{"Sunshade Number 2":string, "Sunshade Number 1":string, "Keyence tuning bank idx":i32}, "AP Test Data":cluster{"Raw Sunshade AP Data":string, "Raw Glass AP Data":string, "PMAC Read Counter":dbl, "Database AP Data":dbl[]}, "Motion Status":cluster{"hmi operator abort start time":u32, "Current Data Index":i32, "Analog Data":sgl[][], "Motor Position Hex":u16, "Messages Index":u16, "Last Bytes":u8[], "Current Hall Position":i16, "Motion Stop Timer":u32, "Position Test":T33, "Noise Test":T33, "motion stop check initialized":bool, "remote sense enabled":bool, "Motion":T3}, "LVDT Status":cluster{"LVDT's stored config":T34[], "lvdt precision":T35}, "Sequence State":T36, "misc status":cluster{"delay start time (ticks)":u32, "In Vehicle Mode?":bool, "Diag Mode?":bool, "Serial Port Configured?":bool, "PS Voltage":dbl, "Diag Serial Port":refnum<visa-resource-name>, "Part Setup":T38, "Part History Number":string, "Plant Number":u8, "AP Data Type":T16, "Real Rollo?":bool}, "NVH Operator?":bool, "NVH Pass?":bool, "Operator Pass?":bool, "Operator Action?":bool, "Noise Source":u32, "USBHandle":i32, "PeakInfo":string, "PeakNumber":i32, "NVH Motion Steps":string[], "Second Check?":bool, "Decibel data":dbl[], "noSCU Paremeter":cluster{"EnableStopOnHome":bool, "EnableStopOnPos":bool, "TeachEvent":bool, "open offset":i32, "close offset":i32, "Derect control":bool, "set position":i32[], "teach pass ":bool, "Drift offsets":i32[], "Hall Positions":i32[]}, "manual control(direct)":bool, "LIN INFO":T43}
  T2 = typedef "All Switch Configuration Cluster.ctl" = cluster{"All Motions":T3, "A":bool[], "B":bool[], "C":bool[], "D":bool[], "A activation time (ms)":u32, "B activation time (ms)":u32, "C activation time (ms)":u32}
  T3 = typedef "All Motions.ctl" = enum16{"Glass Teach", "Glass Slide Open", "Glass Slide Close", "Glass Vent Open", "Glass Vent Close", "Sunshade Teach", "Sunshade Open", "Sunshade Close", "Idle", "Sunshade Open 2", "Sunshade Close 2", "Glass Slide Open Sunshade Open", "Glass Slide Open Sunshade Close", "Glass Slide Close Sunshade Open", "Glass Slide Close Sunshade Close", "Glass Vent Open Sunshade Open", "Glass Vent Open Sunshade Close", "Glass Vent Close Sunshade Open", "Glass Vent Close Sunshade Close", "Express Glass Slide Open", "Express Glass Slide Close", "Express Glass Vent Open", "Express Glass Vent Close", "Express Sunshade Open", "Express Sunshade Close", "Express Sunshade Open 2", "Express Sunshade Close 2", "Express Glass Slide Open Sunshade Open", "Express Glass Slide Open Sunshade Close", "Express Glass Slide Close Sunshade Open", "Express Glass Slide Close Sunshade Close", "Express Glass Vent Open Sunshade Open", "Express Glass Vent Open Sunshade Close", "Express Glass Vent Close Sunshade Open", "Express Glass Vent Close Sunshade Close", "Goto Position Glass", "Goto Position Sunshade", "Sunshade Teach 2"}
  T4 = typedef "EOL Switch Value Configuration Cluster.ctl" = cluster{"All Motions":T3, "Array":T5[]}
  T5 = typedef "EOL Switch Max Min Check Cluster.ctl" = cluster{"Min":dbl, "Max":dbl, "Check?":bool}
  T6 = typedef "station nvh config.ctl" = cluster{"NVH Station?":bool, "nvh app instance path":string, "NVH_ErrorMessages sv url":string, "NVH_Inputs sv url":string, "NVH_MotionNumber sv url":string, "NVH_Outputs sv url":string, "NVH_PartNumber sv url":string, "NVH_PartNumber_Echo sv url":string, "NVH_SerialNumber sv url":string, "NVH_AmbientTempF sv url":string}
  T7 = typedef "station DO map.ctl" = cluster{"Comm Power":T8, "Switch 1":T8, "Switch 2":T8, "Switch 3":T8, "Switch 4":T8, "Switch 5":T8, "Switch 6":T8, "Glass Analog Switch 1":T8, "Glass Analog Switch 2":T8, "Glass Analog Switch 3":T8, "Glass Analog Switch 4":T8, "Glass Motor Relay 1":T8, "Glass Motor Relay 2":T8, "Sunshade Motor Relay 1":T8, "Sunshade Motor Relay 2":T8, "Ignition High":T8, "Ignition Low":T9, "Battery":T8, "Sunshade Analog Switch 1":T8, "Sunshade Analog Switch 2":T8, "Sunshade Analog Switch 3":T8, "Sunshade Analog Switch 4":T8, "NI LIN":T8, "RS232 LIN":T8, "RS232":T8, "CAN":T8, "Park/Enable":T8, "Battery Sense":T8}
  T8 = typedef "EOL Global Digital Output Control.ctl" = enum16{"Battery", "IGN High", "IGN Low", "LIN", "CAN", "Switch 1", "Switch 2", "Switch 3", "Switch 4", "Switch 5", "Switch 6", "Glass Analog Switch 1", "Glass Analog Switch 2", "Glass Analog Switch 3", "Glass Analog Switch 4", "Sunshade Analog Switch 1", "Sunshade Analog Switch 2", "Sunshade Analog Switch 3", "Sunshade Analog Switch 4", "Glass Motor Relay 1", "Glass Motor Relay 2", "Sunshade Motor Relay 1", "Sunshade Motor Relay 2"}
  T9 = typedef "EOL Global Digital Output Control.ctl" = enum16{"Prerun Battery", "Prerun Ignition High", "Prerun Switch 1", "Prerun Switch 2", "Prerun Switch 3", "Prerun Select NI LIN", "Prerun Switch 4", "Prerun Switch 5", "Prerun Switch 6", "Prerun Ignition Low", "Prerun Glass Analog Switch 1", "Prerun Glass Analog Switch 2", "Prerun Glass Analog Switch 3", "Prerun Glass Analog Switch 4", "Prerun Sunshade Analog Switch 1", "Prerun Sunshade Analog Switch 2", "Prerun Sunshade Analog Switch 3", "Prerun Sunshade Analog Switch 4", "Prerun Select RS232 LIN", "Prerun Select RS232", "Prerun Select CAN", "Prerun Park/Enable", "Prerun Communications Power", "Prerun BMW Glass Motor Relay 1", "Prerun BMW Glass Motor Relay 2", "Prerun BMW Sunshade Motor Relay 1", "Prerun BMW Sunshade Motor Relay 2", "Prerun Spare 1", "Prerun Spare 2", "Prerun Spare 3", "Prerun Spare 4", "Prerun Spare 5", "Audit Battery", "Audit Ignition High", "Audit Ignition Low", "Audit Switch 1", "Audit Switch 2", "Audit Switch 3", "Audit Switch 4", "Audit Switch 5", "Audit Switch 6", "Audit Glass Analog Switch 1", "Audit Glass Analog Switch 2", "Audit Glass Analog Switch 3", "Audit Glass Analog Switch 4", "Audit Sunshade Analog Switch 1", "Audit Sunshade Analog Switch 2", "Audit Sunshade Analog Switch 3", "Audit Sunshade Analog Switch 4", "Audit Select NI LIN", "Audit Select RS232 LIN", "Audit Select RS232", "Audit Select CAN", "Audit Park/Enable", "Audit Communications Power", "Audit BMW Glass Motor Relay 1", "Audit BMW Glass Motor Relay 2", "Audit BMW Sunshade Motor Relay 1", "Audit BMW Sunshade Motor Relay 2", "Audit Spare 1", "Audit Spare 2", "Audit Spare 3", "Audit Spare 4", "Audit Spare 5", "Repair Battery", "Repair Ignition High", "Repair Switch 1", "Repair Switch 2", "Repair Select NI LIN", "Repair Ignition Low", "Repair Switch 3", "Repair Switch 4", "Repair Switch 5", "Repair Switch 6", "Repair Glass Analog Switch 1", "Repair Glass Analog Switch 2", "Repair Glass Analog Switch 3", "Repair Glass Analog Switch 4", "Repair Sunshade Analog Switch 1", "Repair Sunshade Analog Switch 2", "Repair Sunshade Analog Switch 3", "Repair Sunshade Analog Switch 4", "Repair Select RS232 LIN", "Repair Select RS232", "Repair Select CAN", "Repair Select Park/Enable", "Repair Communications Power", "Repair BMW Glass Motor Relay 1", "Repair BMW Glass Motor Relay 2", "Repair BMW Sunshade Motor Relay 1", "Repair BMW Sunshade Motor Relay 2", "Repair Spare 1", "Repair Spare 2", "Repair Spare 3", "Repair Spare 4", "Repair Spare 5", "Breakin Battery", "Breakin Igntiion High", "Breakin Ignition Low", "Breakin Switch 1", "Breakin Switch 2", "Breakin Switch 3", "Breakin Switch 4", "Breakin Switch 5", "Breakin Switch 6", "Breakin Glass Analog Switch 1", "Breakin Glass Analog Switch 2", "Breakin Glass Analog Switch 3", "Breakin Glass Analog Switch 4", "Breakin Sunshade Analog Switch 1", "Breakin Sunshade Analog Switch 2", "Breakin Sunshade Analog Switch 3", "Breakin Sunshade Analog Switch 4", "Breakin Select NI LIN", "Breakin Select RS232 LIN", "Breakin Select RS232", "Breakin Select CAN", "Breakin Park/Enable", "Breakin Communications Power", "Breakin BMW Glass Motor Relay 1", "Breakin BMW Glass Motor Relay 2", "Breakin BMW Sunshade Motor Relay 1", "Breakin BMW Sunshade Motor Relay 2", "Breakin Spare 1", "Breakin Spare 2", "Breakin Spare 3", "Breakin Spare 4", "Breakin Spare 5", "Not Implemented"}
  T10 = typedef "station rs232 port map.ctl" = cluster{"PMAC":refnum<visa-resource-name>, "PS Port":refnum<visa-resource-name>, "LVDT Unit":refnum<visa-resource-name>, "RS232":refnum<visa-resource-name>}
  T11 = typedef "station ethernet address map.ctl" = cluster{"LVDT 1 Unit":string, "LVDT Unit 1 port":u16}
  T12 = typedef "station paths.ctl" = cluster{"Base Path":path, "system error log path":path, "Error Table Path":path, "Store errors log path":path, "data bytes log path":path, "network path":path}
  T13 = typedef "EOL Save Module Test Data Control.ctl" = cluster{"Motion Data Array":T14[], "Error Table":string[][], "Sun Shade Close Force Limits":T17, "Sun Shade Open Force Limits":T17, "Sunshade Open Data":sgl[], "Sunshade Close Data":sgl[], "Module Info":T18, "Sunsahde Close Raw Data":sgl[], "Sunshade Open Raw Data":sgl[], "Software Version":string[], "Constant Version":string[], "Hardware Version":string[], "Inalfa Part Number ECU":string[], "LVDT Data":sgl[], "Communication Line 1":sgl[], "Communication Line 2":sgl[], "Anti Pinch Force":sgl[], "Cycle Time":string, "Anti Pinch Vent Force":sgl[], "iGPS LVDT Data":sgl[], "data bytes log":string}
  T14 = typedef "EOL Motion Database Table.ctl" = cluster{"Motion":T3, "Actual Avg Current":dbl, "Actual Runtime":dbl, "Actual Speed":dbl, "Current Data":sgl[], "Motion Data Limits":T15, "Switch 1 to 6":dbl[], "Actual PS Voltage":dbl, "AP Data":i16[][], "Actual max Current":dbl, "Actual Noise (dB)":dbl}
  T15 = typedef "17x Audit Motion Data Seq Control.ctl" = cluster{"Power Supply Voltage":dbl, "Min Avg Current":dbl, "Max Avg Current":dbl, "Min Run Time":dbl, "Max Run Time":dbl, "Min Speed":dbl, "Max Speed":dbl, "AP Data % of Threshold":dbl, "Travel Distance":dbl, "AP Data Type":T16, "Check Current":bool, "Check Run Time":bool, "Check Speed":bool, "Express Motion?":bool, "Check Sound Test":bool, "Check Position?":bool, "Collect AP Data":bool, "Inital Position":u16, "End Position":u16, "Goto Posiition":u16, "Max max Current":dbl, "Min max Current":dbl, "Check max Current":bool, "Check Sound":bool, "Min Sound (dB)":dbl, "Max Sound (dB)":dbl}
  T16 = typedef "17x AP Data Type.ctl" = enum16{"91/61", "92/62", "93/63", "67", "68", "6F", "71", "91 Msg", "92 Msg", "93 Msg", "94 Msg", "HiRain 91", "HiRain 92 Speed", "HiRain 92 HS", "HiRain 92", "HiRain 93", "SnT"}
  T17 = typedef "17x Sunshade Limts Seq.ctl" = cluster{"Overall Min":dbl, "Overall Max":dbl, "Avg Min":dbl, "Avg Max":dbl, "Truncation Start":dbl, "Truncation End":dbl, "Variance":dbl, "Check Noise":bool}
  T18 = typedef "EOL Module Info Control.ctl" = cluster{"Serial Number":string, "Pallet Number":string, "Sunshade Color":string, "Inalfa Part Number":string, "Customer Number":string}
  T19 = typedef "station DI map.ctl" = cluster{"Abort Test":T20, "Start Test":T20}
  T20 = typedef "EOL Global Digital Input Control.ctl" = enum16{"Dev2/port0/line0", "Dev2/port0/line1", "Dev2/port0/line2", "Dev2/port0/line3", "Dev2/port0/line4", "Dev2/port0/line5", "Dev2/port0/line6", "Dev2/port0/line7", "Dev2/port1/line0", "Dev2/port1/line1", "Dev2/port1/line2", "Dev2/port1/line3", "Dev2/port1/line4", "Dev2/port1/line5", "Dev2/port1/line6", "Dev2/port1/line7", "Dev2/port2/line0", "Dev2/port2/line1", "Dev2/port2/line2", "Dev2/port2/line3", "Dev2/port2/line4", "Dev2/port2/line5", "Dev2/port2/line6", "Dev2/port2/line7", "Prerun Start Test", "Prerun Abort Test", "Audit Start Test", "Audit Abort Test", "Dev2/port3/line4", "Dev2/port3/line5", "Breakin Start Test", "Breakin Abort Test", "Not Implemented"}
  T21 = typedef "control refs.ctl" = cluster{"Start Test":refnum<vi>, "Abort Test":refnum<vi>, "Manual Control":refnum<vi>, "Route to Repair":refnum<vi>, "Waveform Graph":refnum<vi>, "Motion Data":refnum<vi>, "all station status":refnum<vi>, "Individual Station Status":refnum<vi>, "exit program":refnum<vi>, "Sunshade Servo Data Open":refnum<vi>, "Sunshade Servo Data Close":refnum<vi>, "Red-Rabbit Mode":refnum<vi>, "Direct Manual Ctrl":refnum<vi>}
  T22 = typedef "misc station config.ctl" = cluster{"Station Name":string, "is AT station?":bool, "is audit station?":bool, "power supply type":T23, "use alt China TP2 LVDT Logic Seq":bool, "hmi operator abort timeout":u32, "dump all analog values even if pass":bool, "debug log pre-filter ap stream bytes":bool, "use separate lvdt x and z extend tags":bool, "is print":bool}
  T23 = typedef "power supply types.ctl" = enum16{"GENser", "ZUPser", "GENeth", "Manual", "ITECH"}
  T24 = typedef "plc comms params.ctl" = cluster{"PLC boolean read Tags":T25, "PLC bool write Tags":T28, "PLC string read Tags":T29, "PLC string write Tags":T30, "use opc":bool, "PLC/OPC Path":string, "PLC float read Tags":T31}
  T25 = typedef "station plc read boolean tags.ctl" = cluster{"AT glass position":T26, "AT shade position":T26, "AT in glass wand lower pos":T26, "AT in sunshad wand lower pos":T26, "AT in wand home pos":T26, "LVDT's Extended":T26, "motor foam present LH":T26, "motor foam present RH":T26, "audit gap hider present LH":T26, "audit gap hider present RH":T26, "FB light block present":T26, "bolt check 1":T26, "bolt check 2":T26, "bolt check 3":T26, "bolt check 4":T26, "bolt check 5":T26, "bolt check 6":T26, "bolt check 7":T26, "bolt check 8":T26, "bolt check 9":T26, "bolt check 10":T26, "bolt check 11":T26, "bolt check 12":T26, "bolt check 13":T26, "bolt check 14":T26, "bolt check 15":T26, "bolt check 16":T26, "bolt check 17":T26, "bolt check 18":T26, "bolt check 19":T26, "bolt check 20":T26, "bolt check 21":T26, "start":T26, "abort":T26, "LVDT's Retracted":T26, "manual barcode print":T26, "ss servo at open":T26, "ss servo at close":T26, "ss servo opening":T26, "ss servo closing":T26, "control slide at home":T26, "control slide left good":T26, "control slide left over stroke":T26, "control slide right good":T26, "control slide right over stroke":T26, "wind deflector high speed pos":T26, "wind deflector low speed pos":T26, "AT VentPMACatHome":T26, "AT VentPMACisExtend":T26, "SS Barcode Scanner Bypassed":T26, "Check Frame Barcode":T26, "iGPS Pass 0":T26, "iGPS Pass 1":T26, "iGPS Pass 2":T26, "iGPS Pass 3":T26, "iGPS Pass 4":T26, "iGPS Pass 5":T26, "iGPS Pass 6":T26, "iGPS Pass 7":T26, "iGPS Pass 8":T26, "iGPS Pass 9":T26, "Z LVDTs Extended":T26, "NVH Operator Pass":T26, "NVH Operator Fail":T26, "NVH Operator Express Glass Open":T26, "NVH Operator Express Glass Close":T26, "NVH Operator Express Rollo Open01":T26, "NVH Operator Express Rollo Close01":T26, "NVH Operator Express Rollo Open02":T26, "NVH Operator Express Rollo Close02":T26, "NVH Operator Vent Open Noise":T26, "NVH Operator Vent Close Noise":T26, "NVH Operator Sunshade Open Noise":T26, "NVH Operator Sunshade Close Noise":T26, "NVH Operator Glass Open Noise":T26, "NVH Operator Glass Close Noise":T26, "NVH Operator Finish":T26, "NVH Operator Check":T26, "AT shade 02 position":T26, "AT in sunshad 02 wand up pos":T26, "AT in wand 02 home pos":T26, "windproof position":T26, "NVH Operator Express Glass vent Open":T26, "NVH Operator Express Glass Vent Close":T26, "NVH Operator Re-do":T26, "AT at vent ATS test pos":T26, "AT at vent ATS Home pos":T26, "Start Adjust LVDT":T26, "Finish Adjust LVDT":T26}
  T26 = typedef "plc path and tag.ctl" = cluster{"Tag Name":string, "Network Path":string, "use opc":bool, "DataSocket Reference":T27}
  T27 = typedef "DataSocket Reference Type.ctl" = cluster{"CWDSLib._DCWDataSocket":refnum<k7>, "CWDSLib._DCWData":refnum<k7>, "OnDataUpdated":u32, "OnStatusUpdated":u32}
  T28 = typedef "station plc write boolean tags.ctl" = cluster{"AT set glass wand lower":T26, "AT set sunshade wand lower":T26, "AT set wand home pos":T26, "Test Complete Pass":T26, "Test Complete Fail":T26, "Test Started":T26, "Retract LVDT's":T26, "Extend LVDT's":T26, "ss servo open":T26, "ss servo close":T26, "control slide start":T26, "control slide stop":T26, "AT VentPMACHome":T26, "AT VentPMACExtended":T26, "Good Frame Barcode":T26, "Bad Frame Barcode":T26, "Extend Z LVDTS":T26, "NVH SunRoof Moving":T26, "NVH SunRoof Stop":T26, "NVH Pass":T26, "NVH Fail":T26, "NVH Operator Express Glass Opened":T26, "NVH Operator Express Glass Closed":T26, "NVH Operator Express Rollo Opened01":T26, "NVH Operator Express Rollo Closed01":T26, "NVH Operator Express Rollo Opened02":T26, "NVH Operator Pass":T26, "NVH Operator Fail":T26, "NVH Operator Check":T26, "NVH Operator Vent Open Noise":T26, "NVH Operator Vent Close Noise":T26, "NVH Operator Sunshade Open Noise":T26, "NVH Operator Sunshade Close Noise":T26, "NVH Operator Glass Open Noise":T26, "NVH Operator Glass Close Noise":T26, "NVH Operator Finish":T26, "AT set sunshade 02 wand up":T26, "AT set wand 02 home pos":T26, "Barcode01 OK":T26, "Barcode02 OK":T26, "AT set to Vent ATS Test Pos":T26, "AT set to Vent ATS Home Pos":T26, "Move LVDT Adjust Station":T26}
  T29 = typedef "station plc read string tags.ctl" = cluster{"Serial Number":T26, "Pallet Number":T26, "Inalfa Part Number":T26, "Shade Color":T26, "Model Type":T26, "Customer Number":T26, "Part History Number":T26, "Shade 1 Barcode":T26, "Shade 2 Barcode":T26, "Manual Serial Number":T26, "Manual Inalfa Part Number":T26, "Manual Shade Color":T26, "Manual Model Type":T26, "Manual Customer Number":T26, "Manual Part History Number":T26, "iGPS SN 0":T26, "iGPS SN 1":T26, "iGPS SN 2":T26, "iGPS SN 3":T26, "iGPS SN 4":T26, "iGPS SN 5":T26, "iGPS SN 6":T26, "iGPS SN 7":T26, "iGPS SN 8":T26, "iGPS SN 9":T26}
  T30 = typedef "station plc write string tags.ctl" = cluster{"barcode station error":T26, "error message 0":T26, "error message 1":T26, "error message 2":T26, "error message 3":T26, "error message 4":T26, "error message 5":T26, "error message 6":T26, "error message 7":T26, "error message 8":T26, "error message 9":T26}
  T31 = typedef "station plc read float tags.ctl" = cluster{"iGPS float read tags":T32[]}
  T32 = typedef "iGPS float tags.ctl" = cluster{"LVDT measurements":cluster{"value":T26, "UCL":T26, "LCL":T26, "LVDT Name":string}[]}
  T33 = typedef "Pass Fail Control.ctl" = enum16{"Not Tested", "Pass", "Fail"}
  T34 = typedef "EOL LVDT's Check Controller.ctl" = cluster{"Upper Limit":dbl, "Lower Limit":dbl, "LVDT Name":string, "Check":bool}
  T35 = typedef "lvdt precision.ctl" = cluster{"truncate instead of rounding":bool, "decimal places":u8}
  T36 = typedef "sequence state.ctl" = cluster{"Step Description":string, "Cycle Start Time":u32, "Step Data String":string, "Pass?":bool, "Seqence":T37[], "Active Step":u8, "Testing?":bool, "Red-Rabbit Mode":bool, "route-to-repair mode":bool, "NVH Status":cluster{"Restart IRQ Counter":u8, "NVH Test Needed?":bool, "NVH Test Running?":bool}, "Present (s)":dbl, "Hold Mode?":bool, "Hold?":bool, "Rx Invalid?":bool}
  T37 = typedef "Sequence Info.ctl" = cluster{"Name":string, "Description":string, "data string":string}
  T38 = typedef "EOL Part Setup.ctl" = cluster{"Communication Type":T39, "Send Messages to":T40, "RAP Signal":T41, "Motor Type":T42, "NVH Part Number":u16, "Turn Off Timer":u16, "Part Type":string}
  T39 = typedef "All Communication Types.ctl" = enum16{"None", "CAN", "RS 232", "RS 232 LIN", "GM LIN", "SnT LIN", "K Line", "Robel CAN", "P42M-Continental", "Inalfa SCU LIN", "Spare 3"}
  T40 = typedef "Communication with Motors.ctl" = enum16{"Glass", "Rollo", "Both"}
  T41 = typedef "RAP Signal Control.ctl" = enum16{"High", "Low", "None"}
  T42 = typedef "EOL Motor Type.ctl" = enum16{"Smart Motor", "Sensor Motor"}
  T43 = typedef "station LIN config.ctl" = cluster{"Toolkit Type":enum16{"Inalfa LIN", "ADCS LIN", "TS LIN"}, "NAD":u8, "Inalfa LIN":T44, "ADCS LIN":T45, "TS LIN":cluster{"ref info":refnum<k24>, "LIN Channel":i32, "ByteCmd Path":path}}
  T44 = typedef "LIN Device.ctl" = cluster{"Master Frame(3C)":refnum<k21>, "Slave Frame(3D)":refnum<k21>, "Request Schedule":refnum<k21>, "Response Schedule":refnum<k21>, "Frame Write SCU":refnum<k21>, "Frame Read SCU":refnum<k21>, "LIN Name":refnum<k21>}
  T45 = typedef "ADCS_LIN info.ctl" = cluster{"Port":string, "HW select":u16, "XNET Cluster":string, "ByteCmd Path":path}
  T46 = enum32{"Invalid", "Standard", "Closed", "Hidden", "Minimized", "Maximized"}
  T47 = enum32{"invalid app kind", "Development System", "Run Time System", "Student Edition", "Embedded LabVIEW", "Evaluation", "Custom"}
  T48 = typedef "EOL Global Digital Output Cluster Control.ctl" = cluster{"Status":bool, "Global DO Ch":T8}
  T49 = enum16{"Init", "Write", "Write All", "Clear All", "Stop"}
  T50 = typedef "lvdt name val pair.ctl" = cluster{"lvdt name":string, "value":dbl}
  T51 = typedef "NVH Mode Control 2.0.ctl" = enum16{"Init", "Write", "Write String", "Read", "Write Part Number", "Write Motion Number", "Write Ambient TempF"}
  T52 = cluster{"Core":cluster{"Current VI Reference":refnum<vi>, "Close Panel on Exit?":bool}, "Your Boolean data":bool, "Your string data":string, "Main State Cluster":T1}
  T53 = cluster{"Current VI Reference":refnum<vi>, "Close Panel on Exit?":bool}
  T54 = typedef "individual station status.ctl" = cluster{"Line Number":u8, "Serial Port":bool, "Loop Stopped?":bool, "Nidec Serial #":string, "Platform Constant":string, "ATS Constant":string, "Position Constant":string, "Schematic Ver":string, "Bootloader Ver":string, "Hardware Ver":string, "Vehicle Type":string, "Inalfa Motor P/N":string, "System Mode":string, "DTC's?":bool, "Calibrated?":bool, "Slide Count":u16, "Vent Count":u16, "Glass Voltage":dbl, "Anti Pinch Test?":bool, "Station":string}
  T55 = typedef "station hmi.ctl" = cluster{"Error Table Br":string[][], "Pass / Fail":u32, "Cycle Time Br":dbl, "Sunroof Barcode":string, "Pallet Number":string, "Part Type":string, "Current Step Br":string, "Application Status":string, "Station Name":string, "Database LVDT's Data Out":T50[], "NVH System":bool, "Date":string, "Time":string}
  T56 = cluster{"Noise Test":T33, "Avg Current":dbl, "Run Time":dbl, "Speed":dbl, "Position":T33}
  T57 = typedef "station motion data indicator.ctl" = cluster{"Shade Close Limits":T58, "Shade Close Data 2":T58, "Shade Open Limits":T58, "Shade Open Data":T58, "Vent Close Limits":T58, "Vent Close Data":T58, "Vent Open Limits":T58, "Vent Open Data":T58, "Slide Close Limits":T58, "Slide Close Data":T58, "Slide Open Limits":T58, "Slide Open Data":T58}
  T58 = typedef "Screen Motion Data.ctl" = cluster{"Noise Test":T33, "Avg Current":dbl, "Run Time":dbl, "Speed":dbl, "Position":T33}
  T59 = typedef "NVH Digital Input.ctl" = enum16{"Online", "Pass", "Fail", "Testing", "Ready for Model", "Error Bit 1", "Error Bit 2", "Error Bit 3", "Failure Bit 1", "Failure Bit 2", "Failure Bit 3", "Failure Bit 4", "Echo Bit 1", "Echo Bit 2", "Echo Bit 3", "Echo Bit 4", "Serial Number Read Ok", "Ready for Serrial Number"}
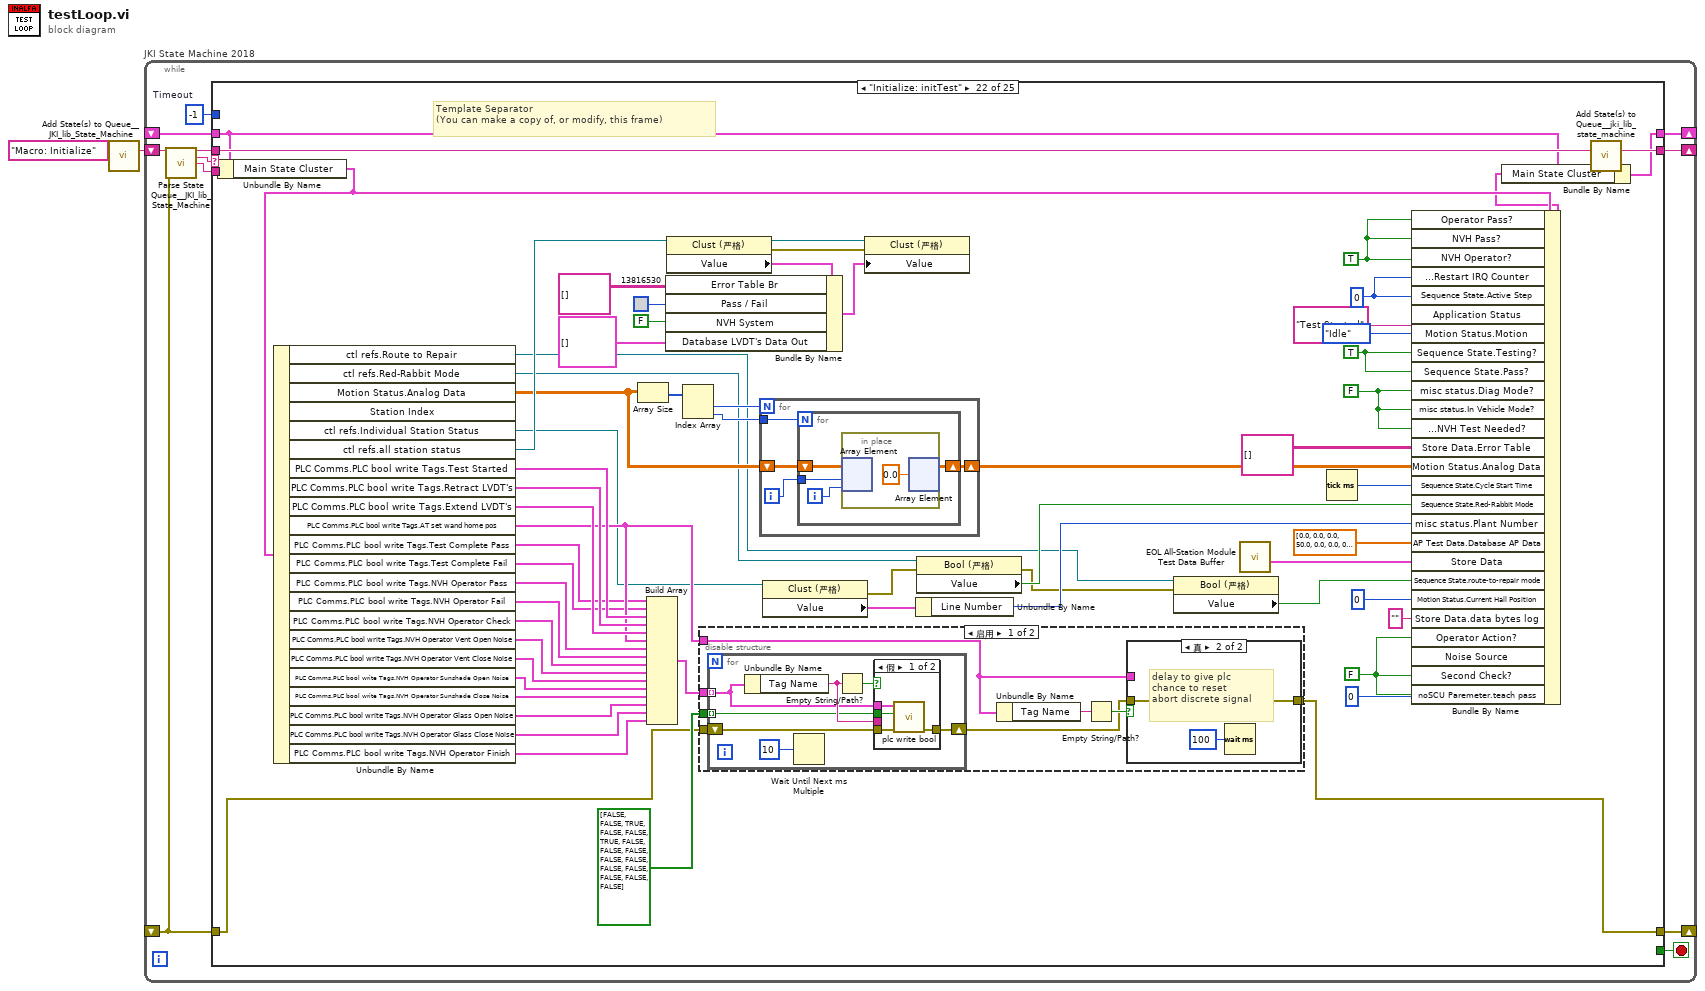
[diagram p0: block diagram]
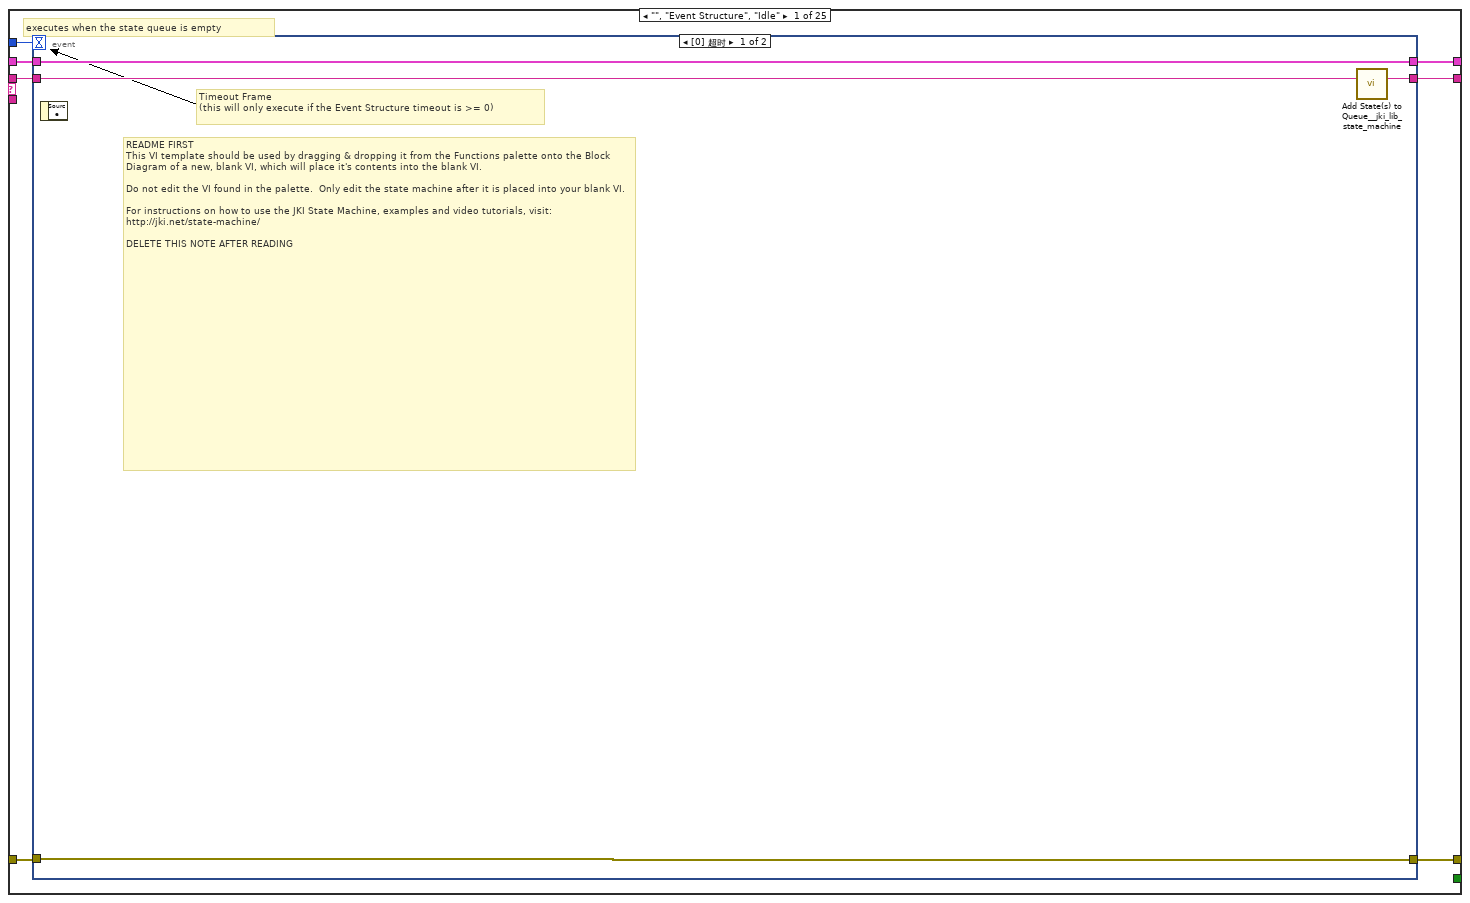
[diagram p2: hidden frame]
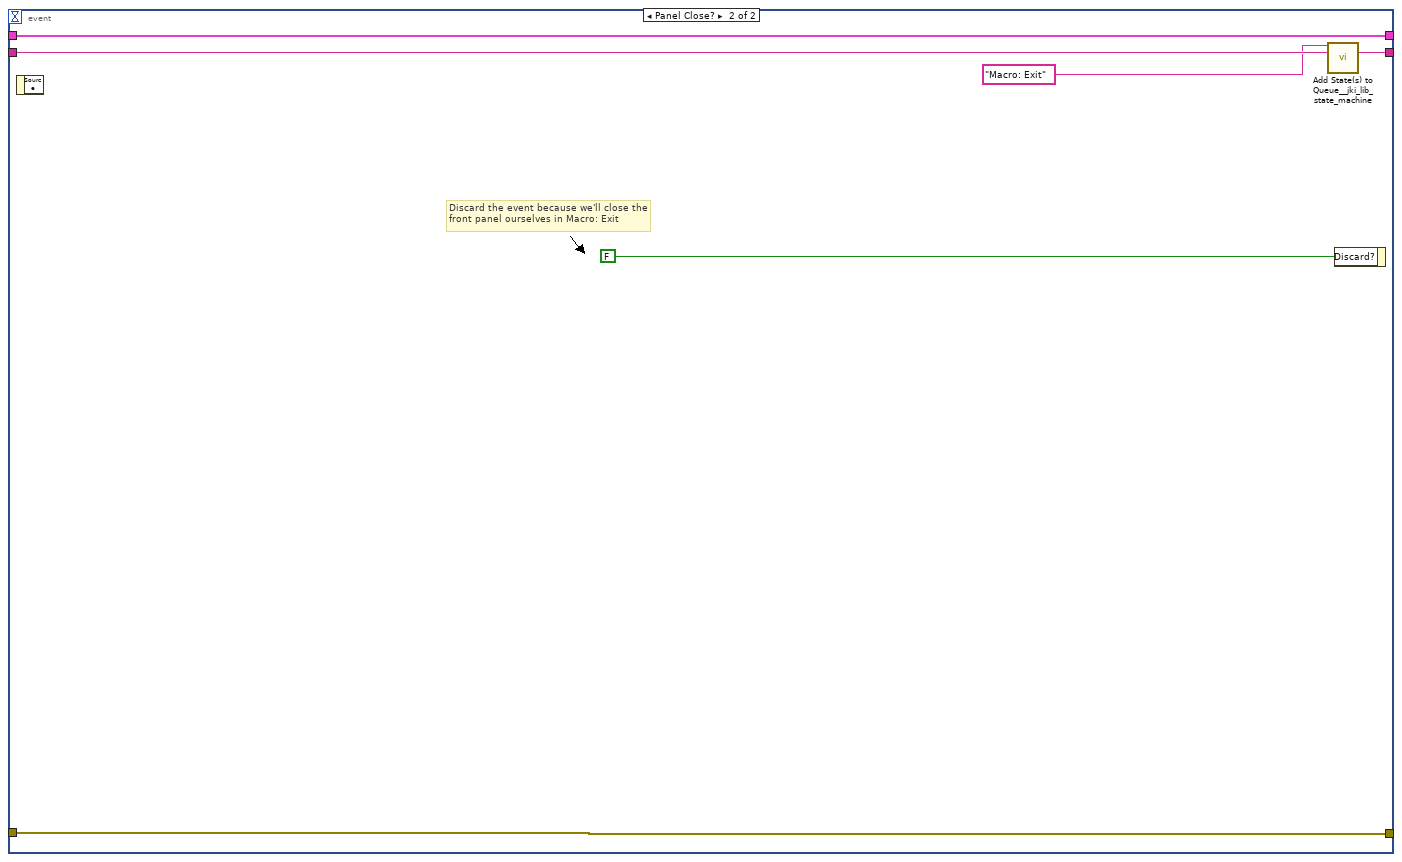
[diagram p3: hidden frame]
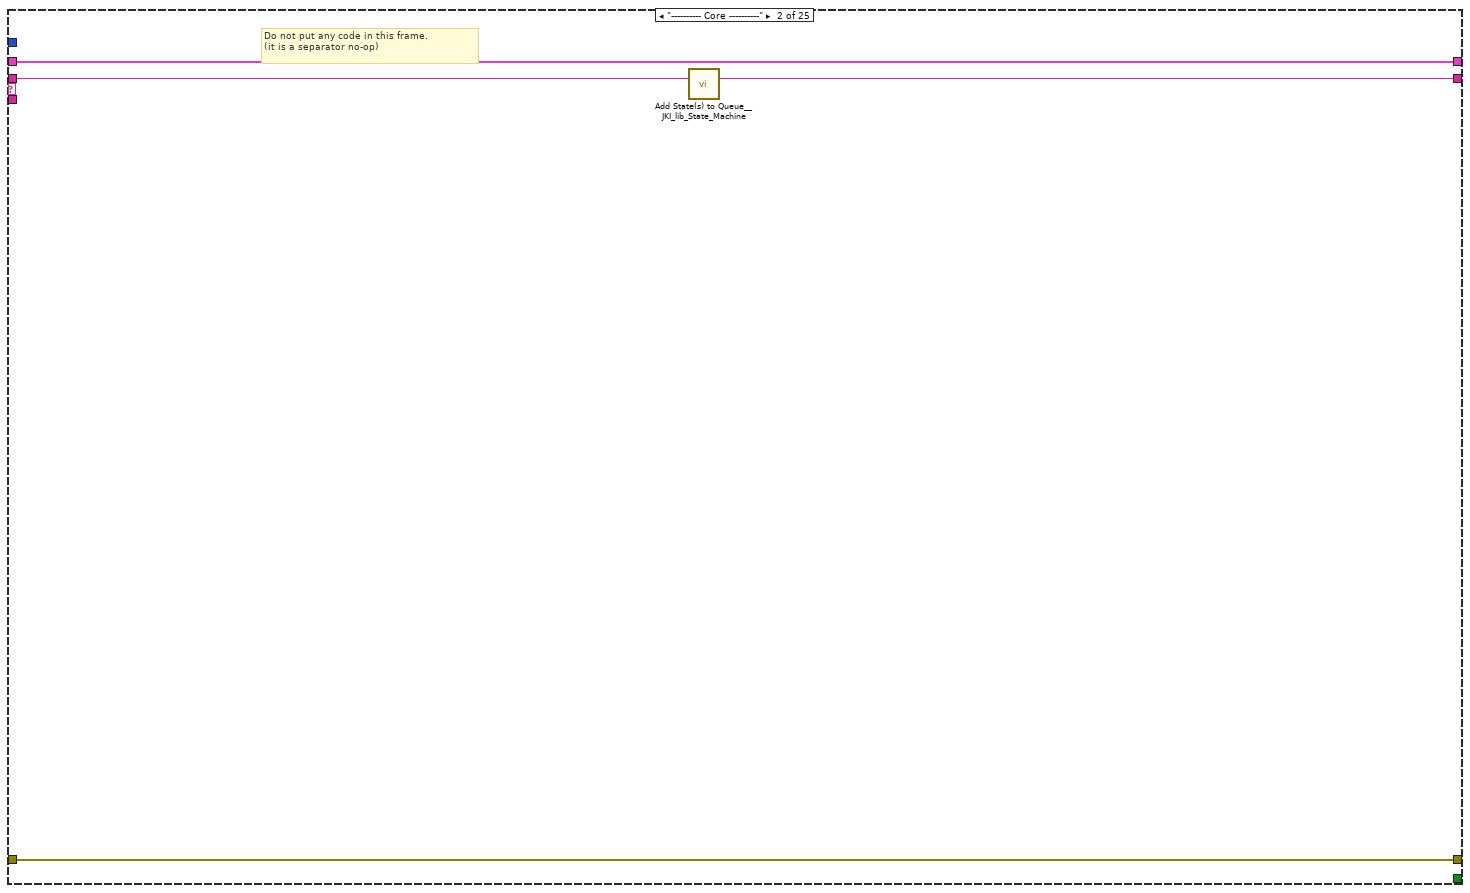
[diagram p4: hidden frame]
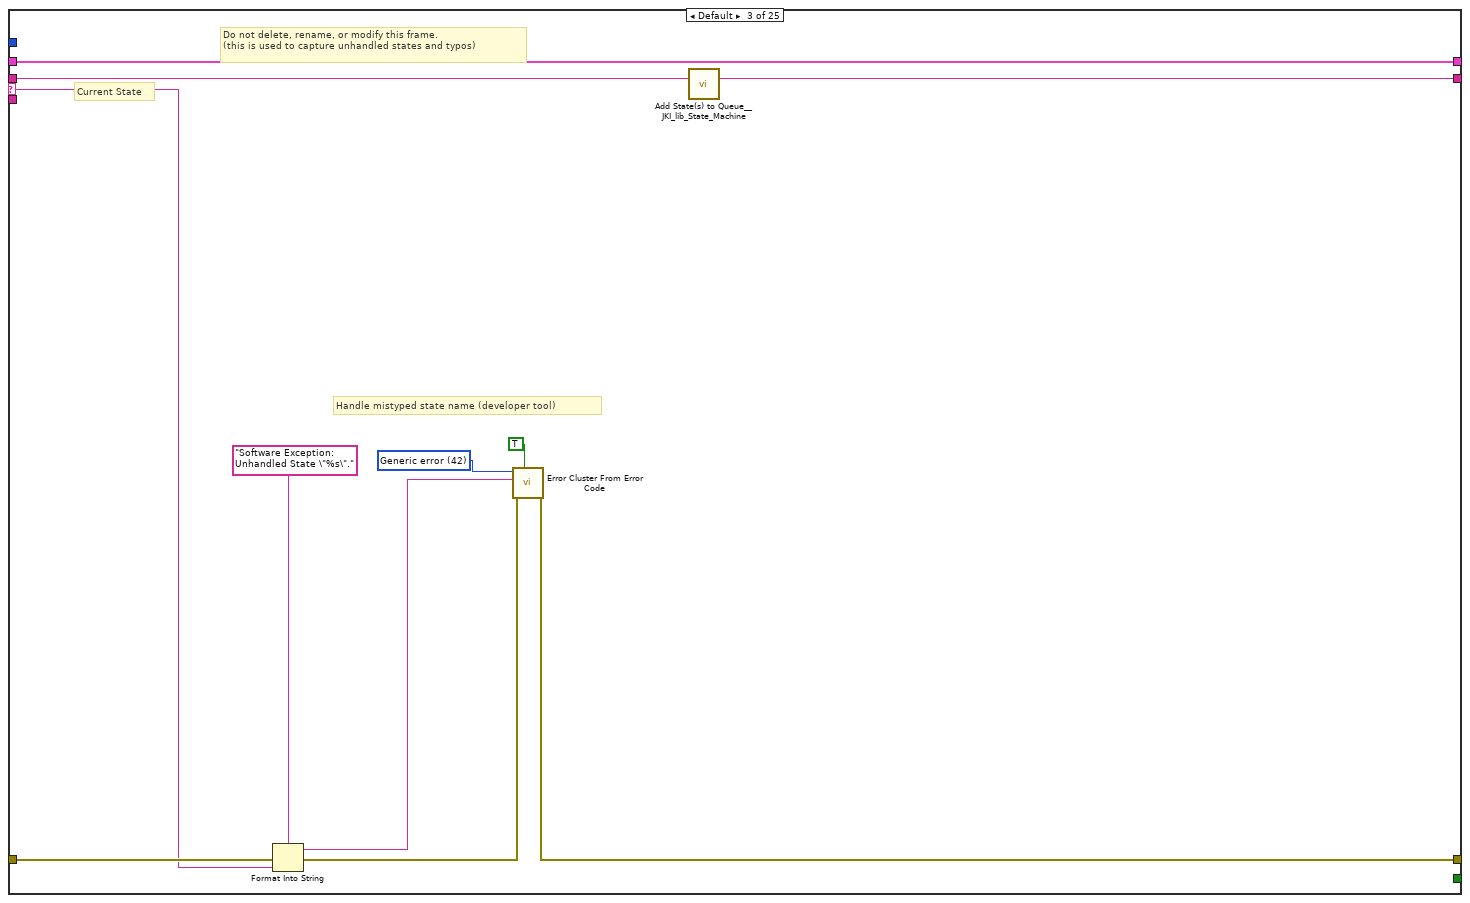
[diagram p5: hidden frame]
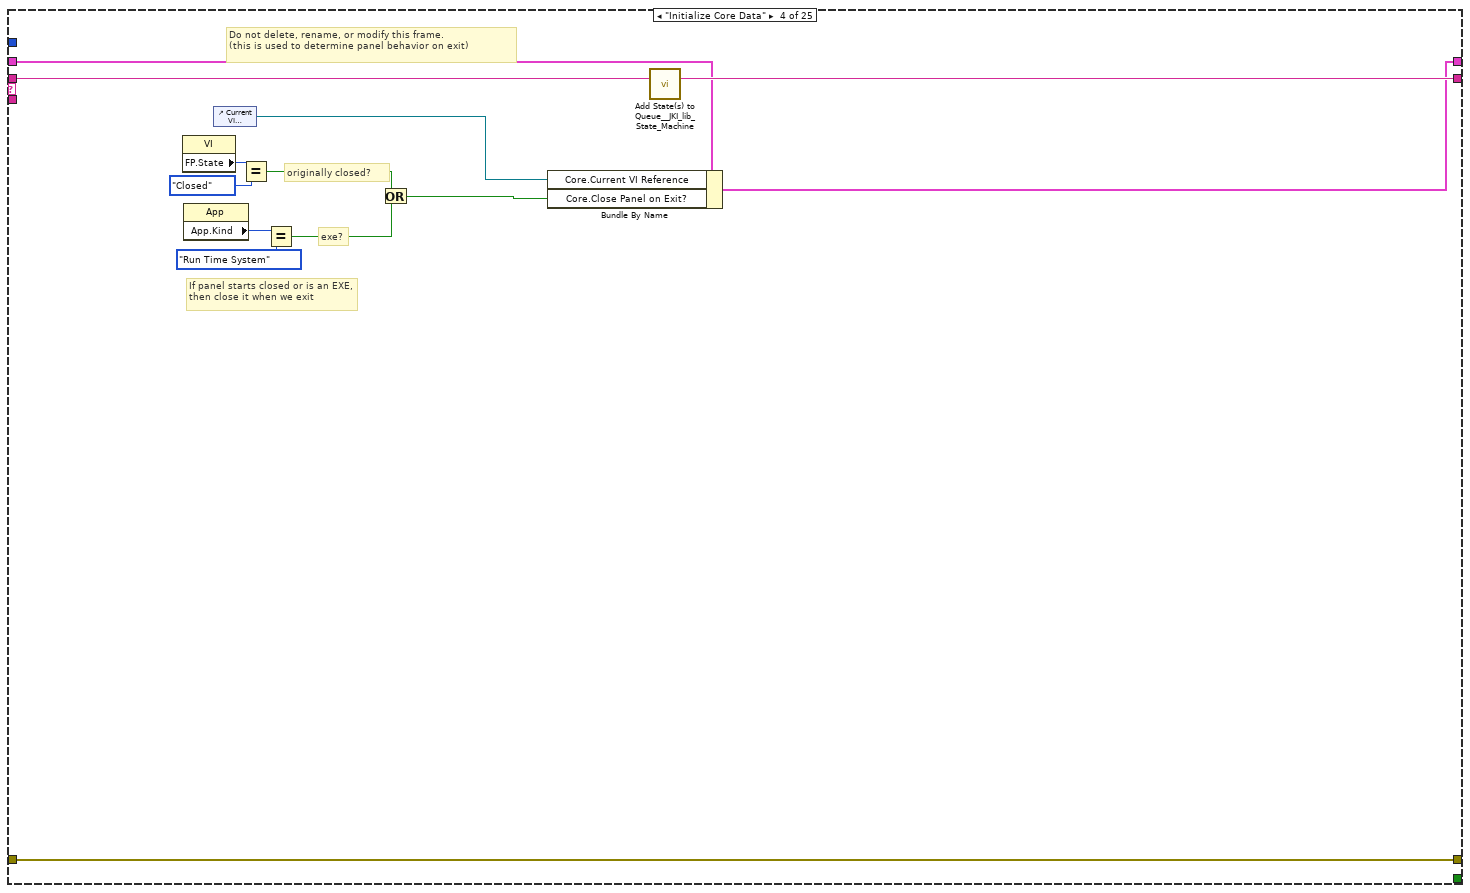
[diagram p6: hidden frame]
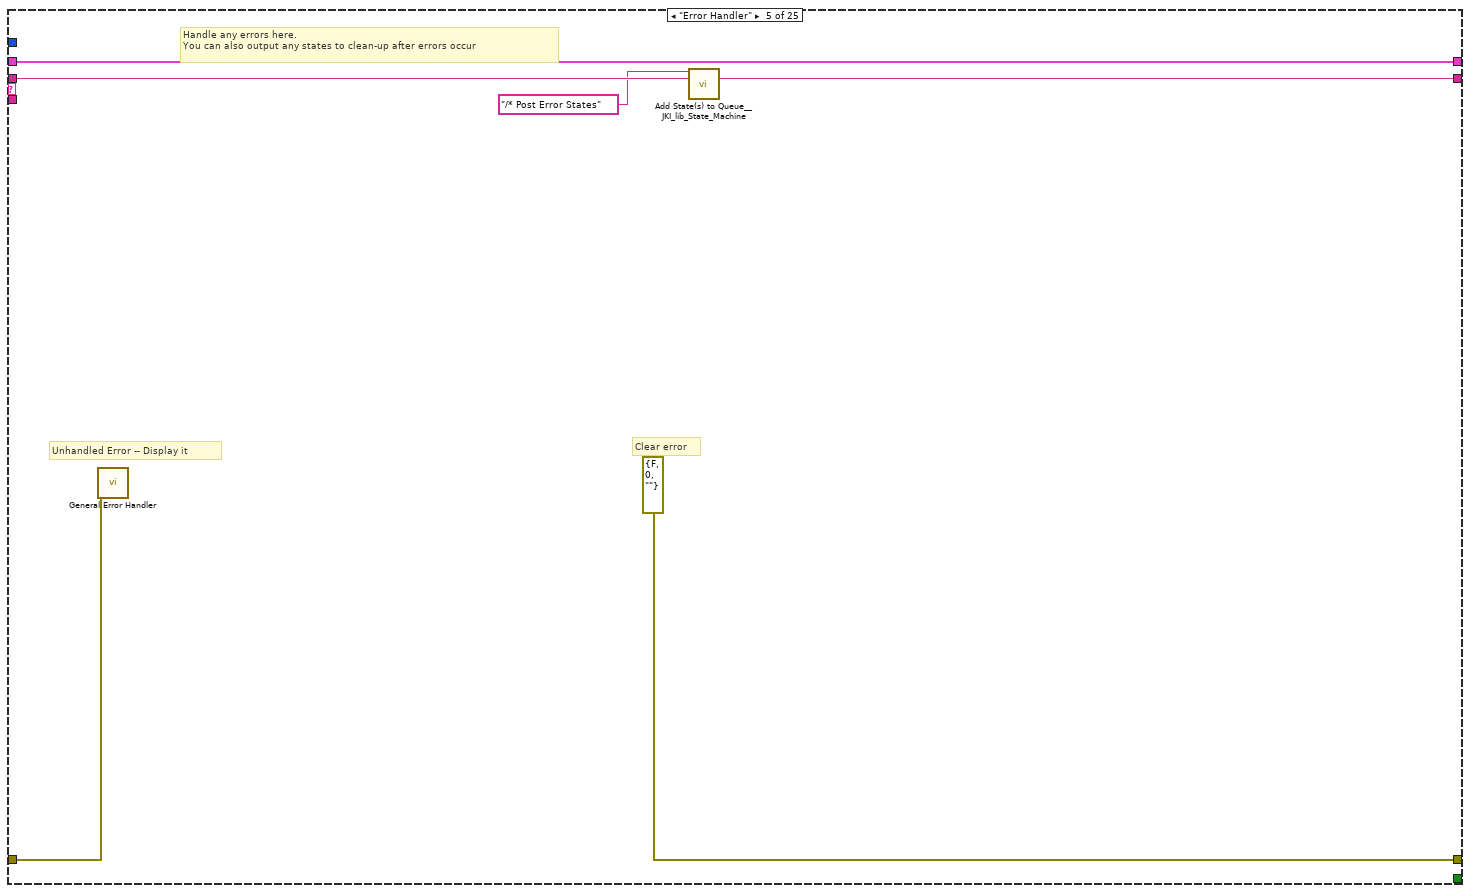
[diagram p7: hidden frame]
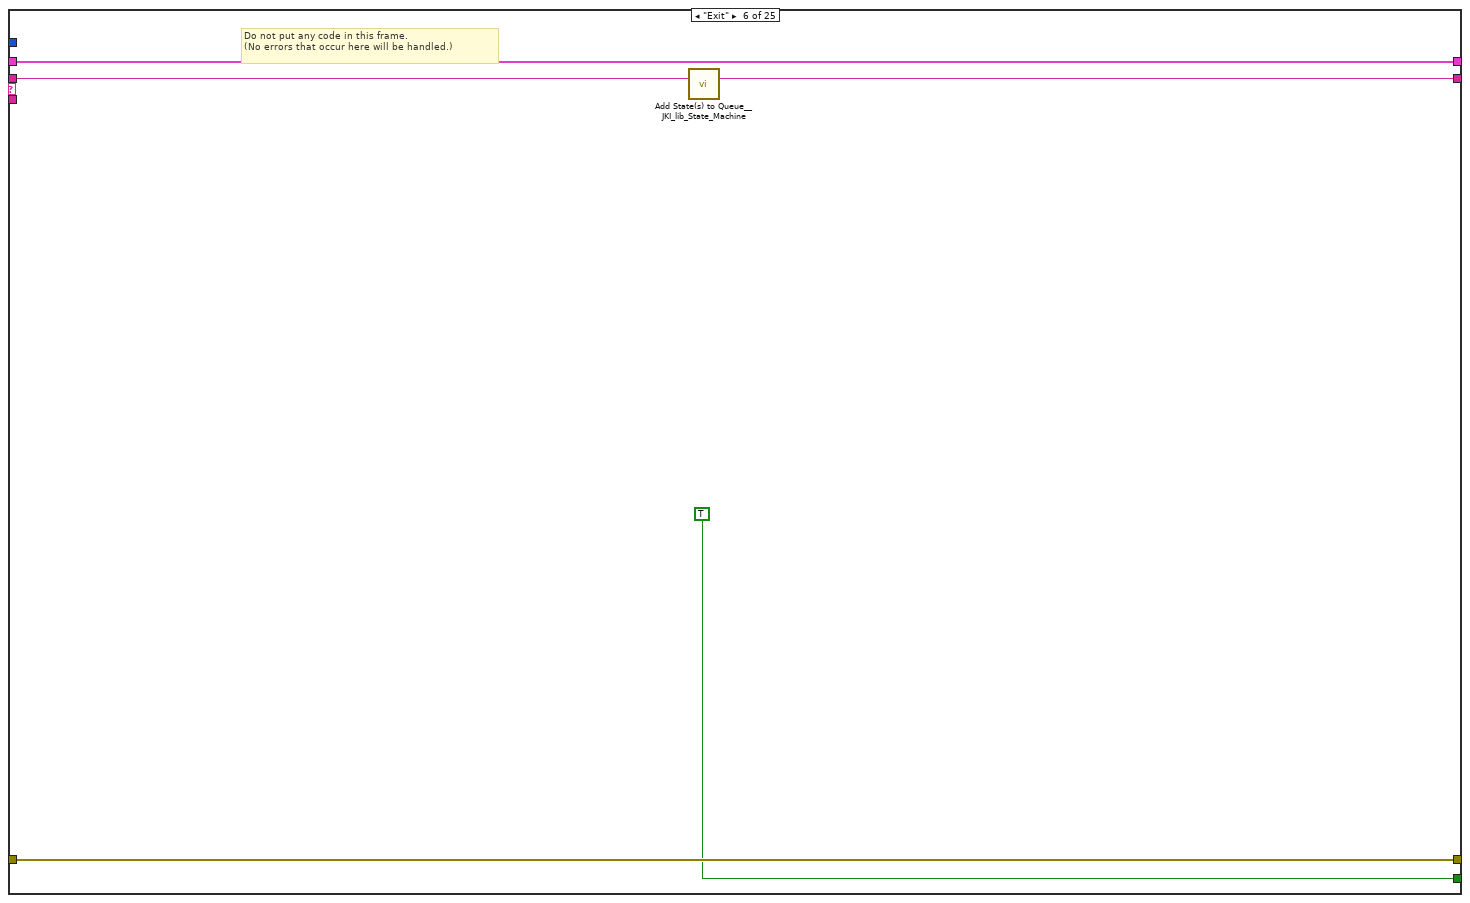
[diagram p8: hidden frame]
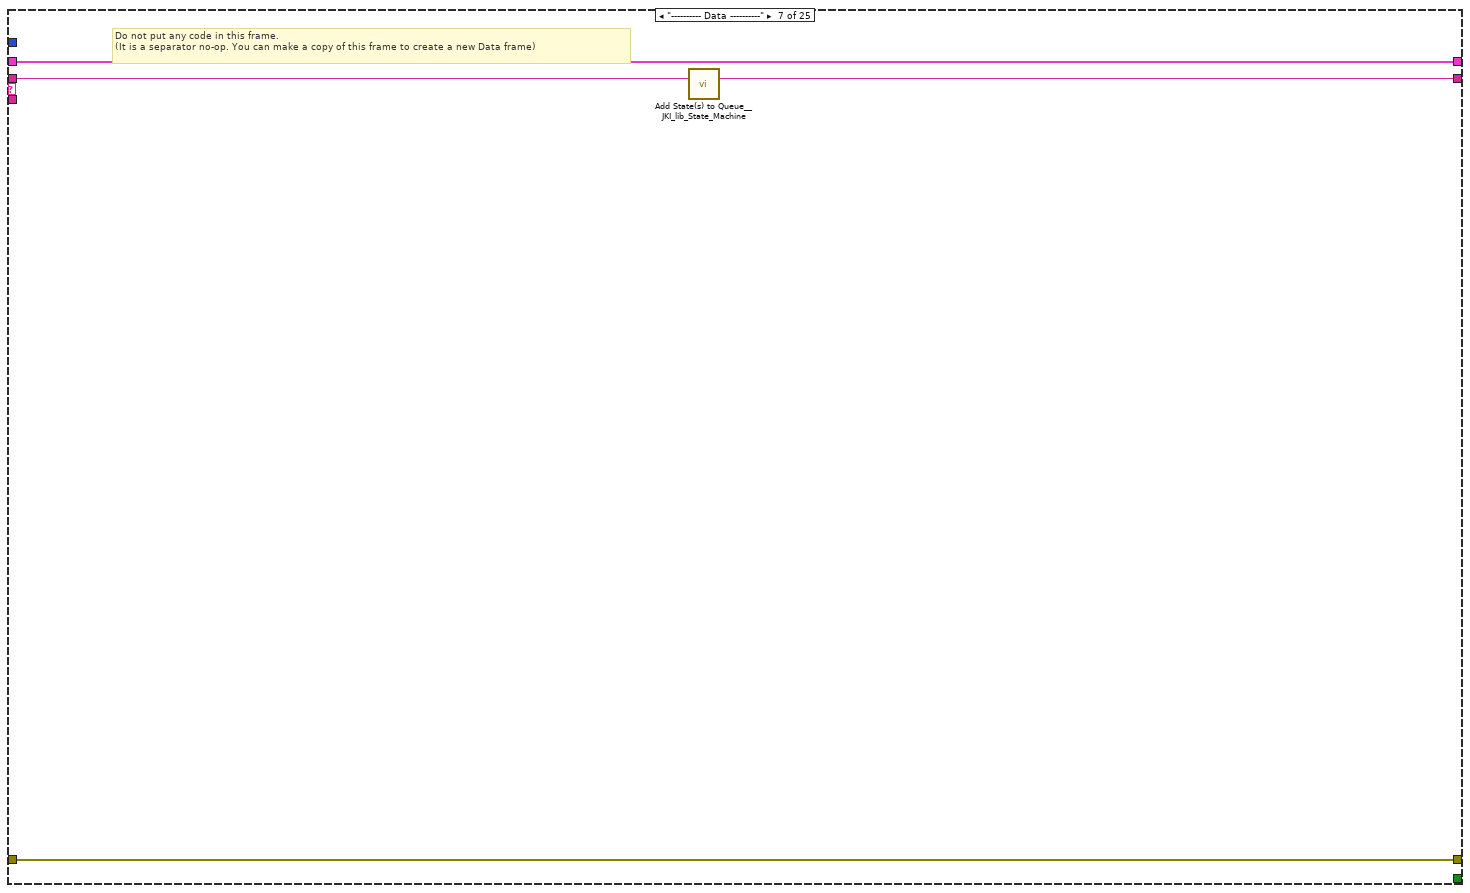
[diagram p9: hidden frame]
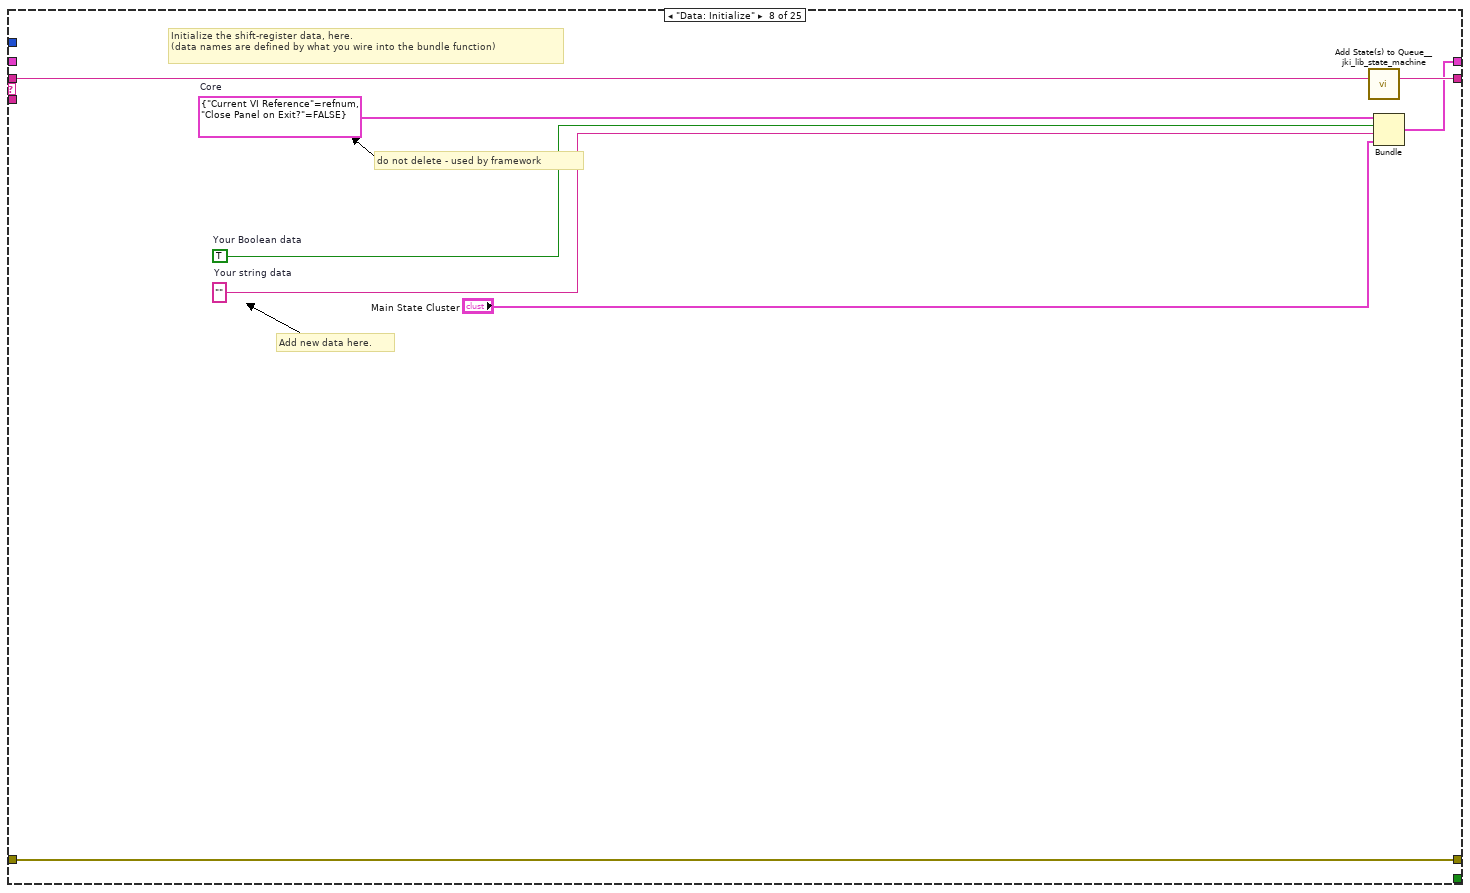
[diagram p10: hidden frame]
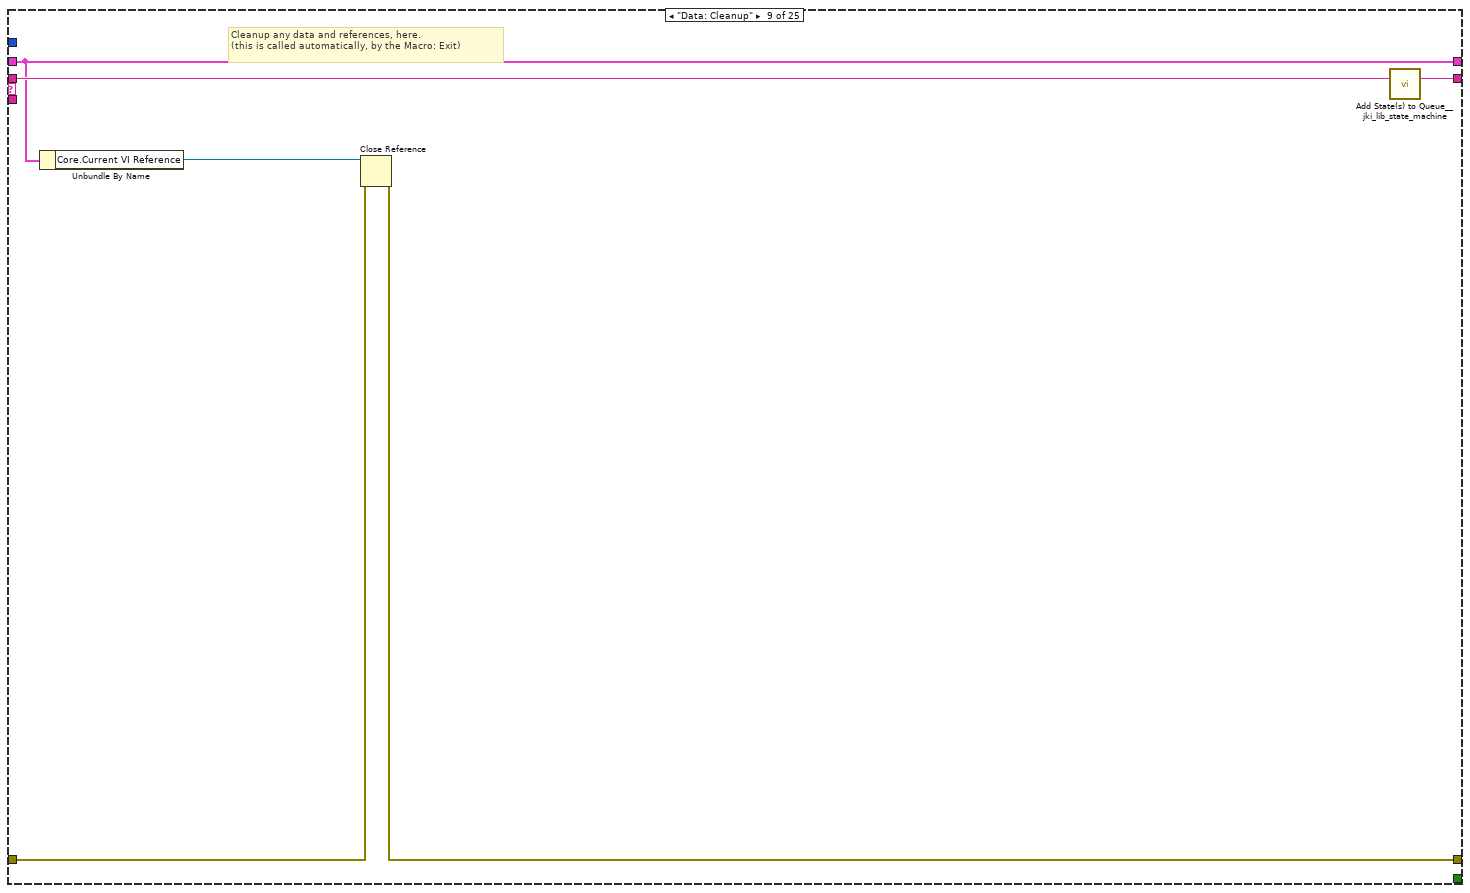
[diagram p11: hidden frame]
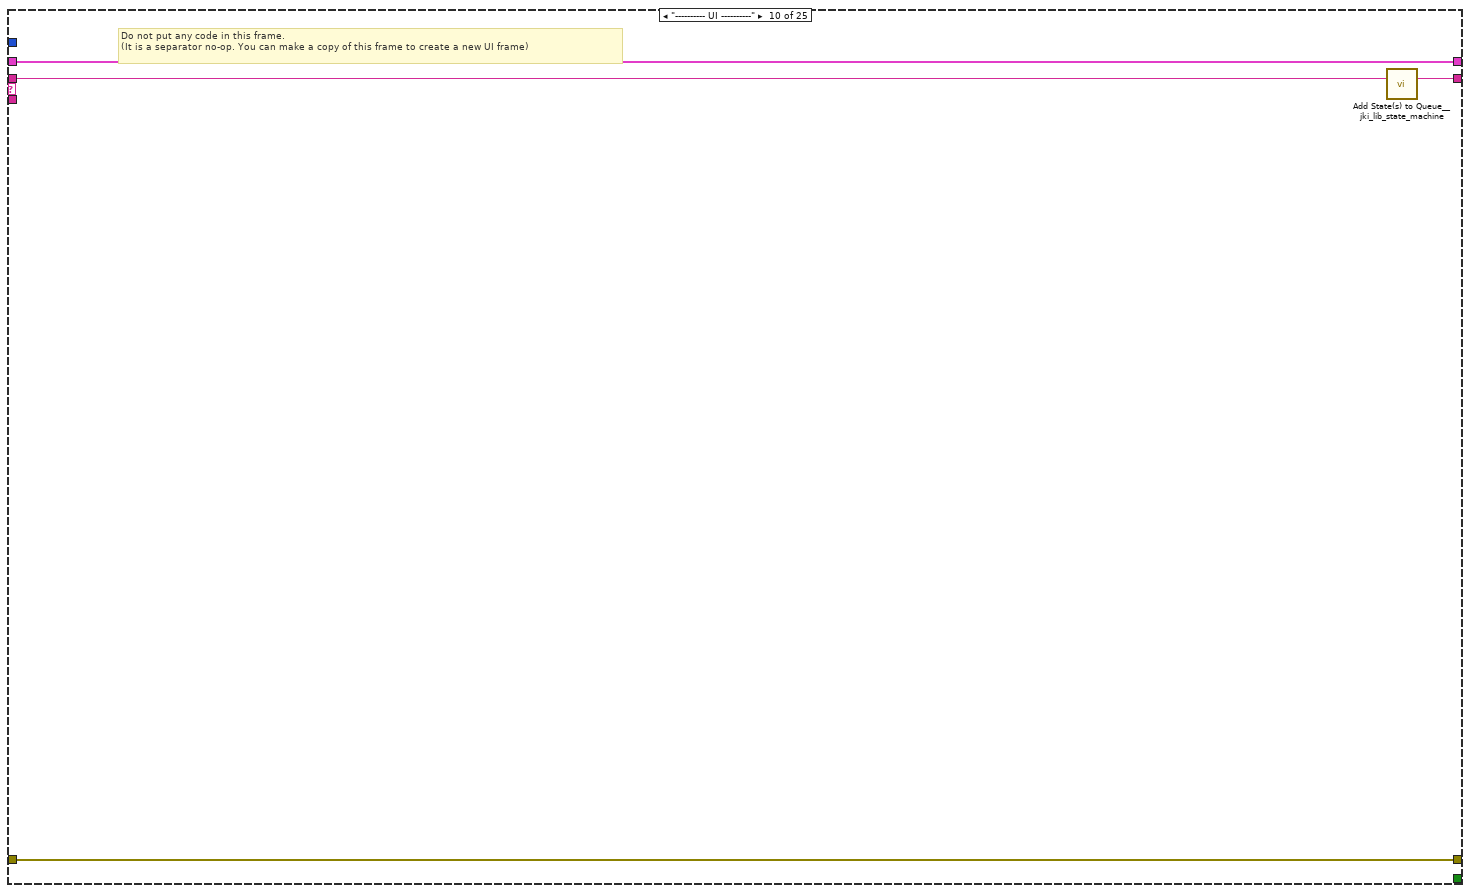
[diagram p12: hidden frame]
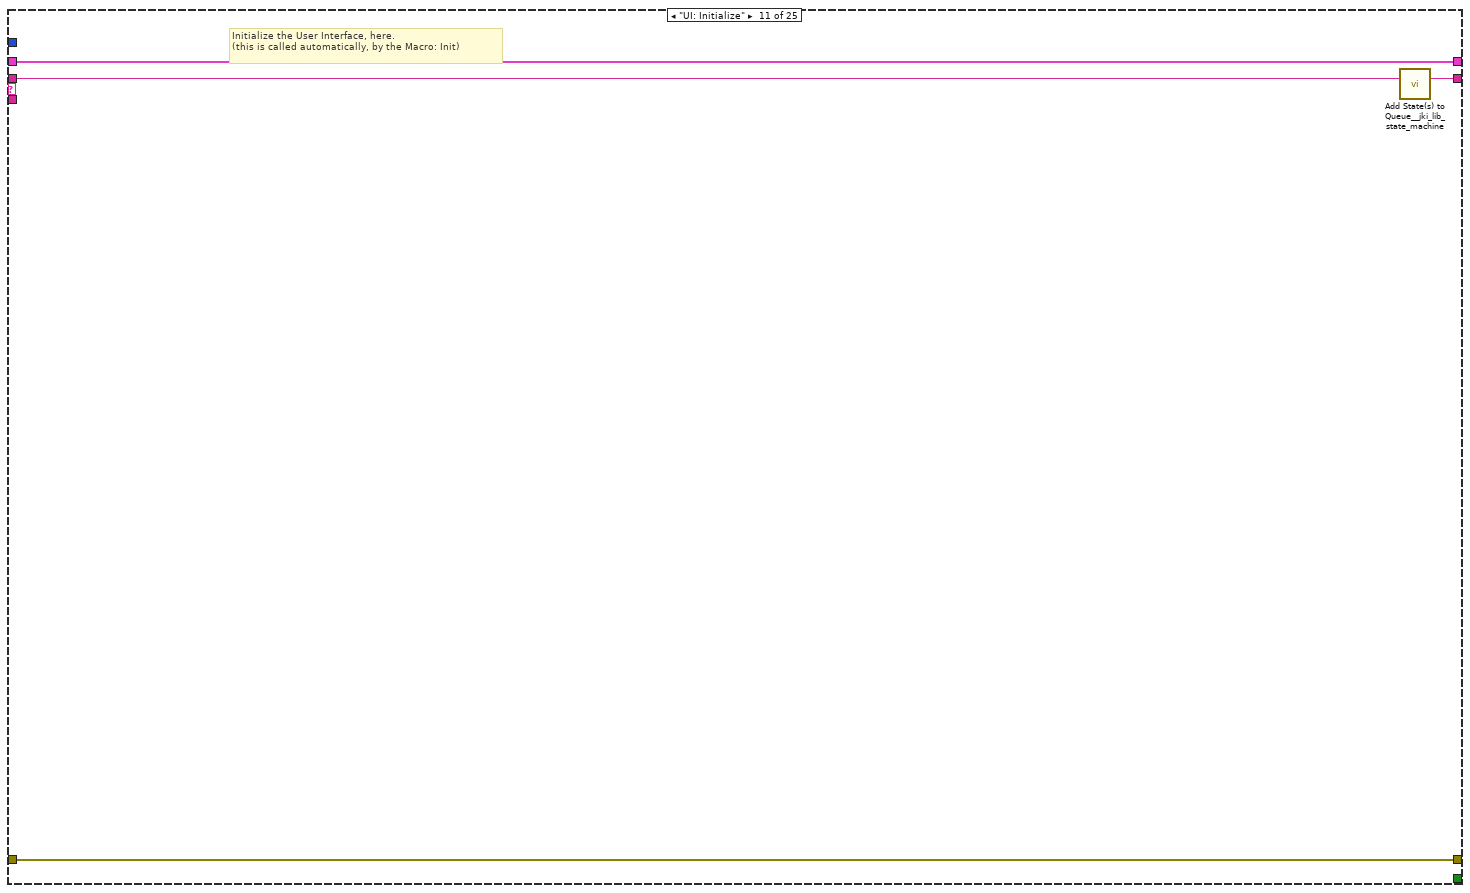
[diagram p13: hidden frame]
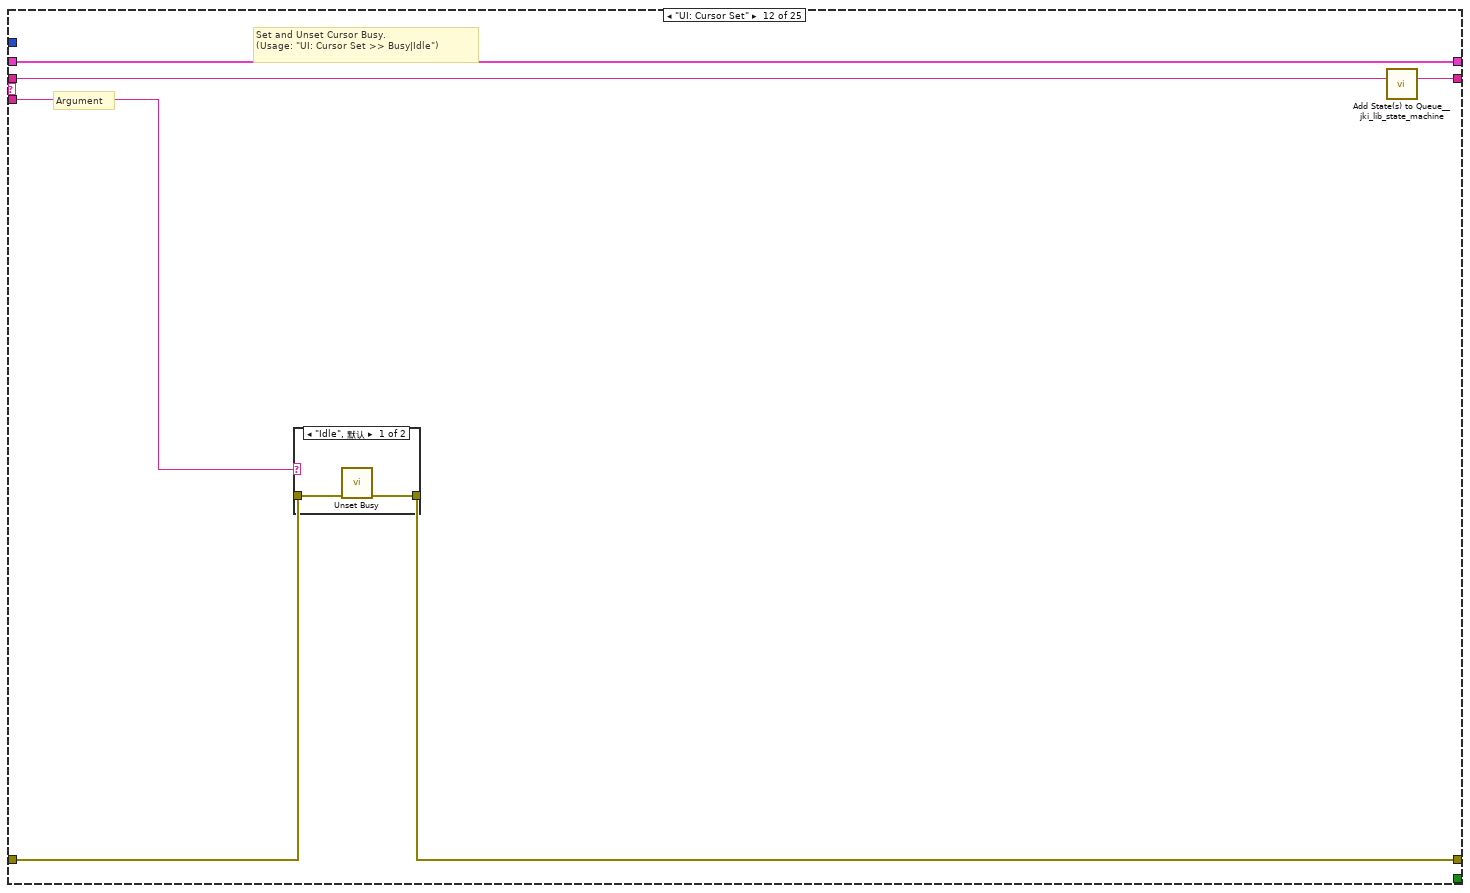
[diagram p14: hidden frame]
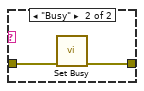
[diagram p15: hidden frame]
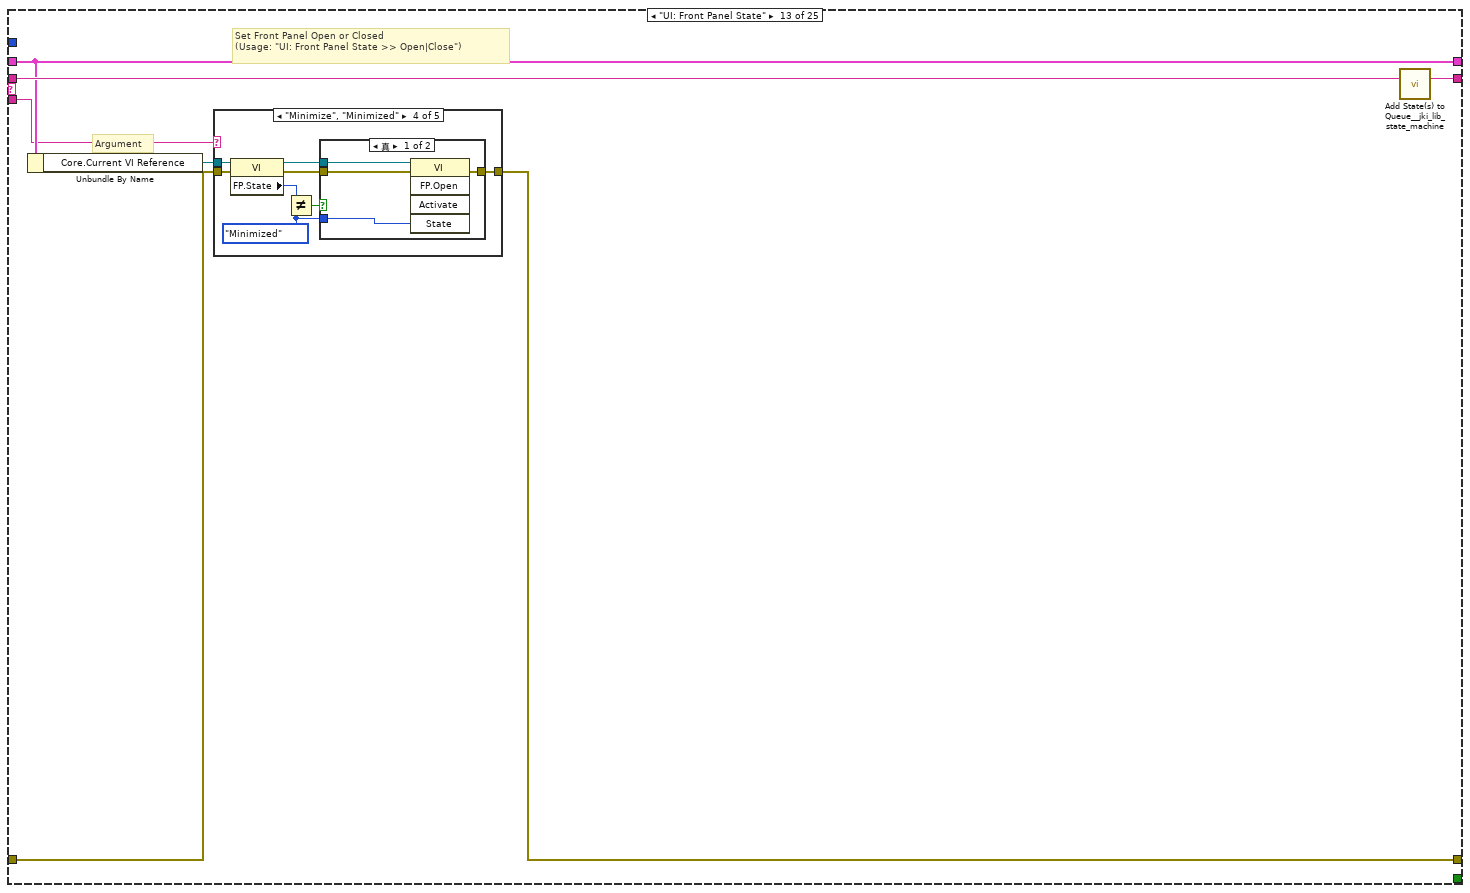
[diagram p16: hidden frame]
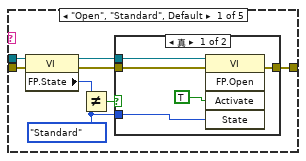
[diagram p17: hidden frame]
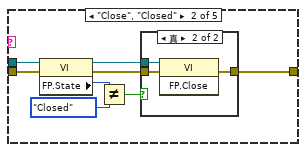
[diagram p19: hidden frame]
diagram:
  n1 = call <vilib>:"Add State(s) to Queue__JKI_lib_State_Machine.vi"("State(s) in (\"\")"="Macro: Initialize") -> ("States Out"=w2:string)  [unwired: 14 in]
  n2 = while "JKI State Machine 2018" {
    shift-right: [w6] -> _
    shift-left: _ -> [w5]
    shift-right: [w9] -> _
    shift-left: _ -> [w3]
    shift-right: [w8] -> _
    shift-left: w2 -> [w10]
    stop <- w7 stop-if-true
    w4 = -1  # Timeout
    n3 = call <vilib>:"Parse State Queue__JKI_lib_State_Machine.vi"("State Queue"=w10, "Error In (no error)"=w3) -> ("Remaining States"=w12:string, "Current State"=w13:string, "Arguments"=w11:string)  [unwired: 11 in]
    n4 = case shown="\"Initialize: initTest\"" w13 {
      selector: w13 -> [_ _ w35 _ _ _ _ _ _ _ _ _ _ _ _ _ _ _ _ _ _ _ _ _ _]
      tunnel: w12 -> [w20 w34 w39 w58 w64 w69 w73 w81 w87 w91 w95 w101 w112 w181 w186 w196 w200 w255 w317 w358 w401 w492 w531 w563 w568]
      tunnel: w11 -> [_ _ _ _ _ _ _ _ _ _ _ w96 w106 _ _ _ _ _ _ _ _ _ _ _ _]
      tunnel: w5 -> [w18 w31 w37 w51 w61 w67 w70 _ w82 w88 w93 w99 w108 w178 w183 w193 w197 w204 w296 w349 w361 w433 w534 w560 w565]
      tunnel: [w17 w32 w41 w55 errorcluster {"status"=FALSE, "code"=0, "source"=""} ("error out") w66 w71 w78 w83 w89 w92 w97 w109 w179 w184 w194 w198 w202 w297 w356 w362 w434 w538 w561 w566] -> w9
      tunnel: w3 -> [w16 w32 w40 w55 w60 w66 w71 w78 w84 w89 w92 w98 w110 w179 w184 w194 w198 w203 w298 w356 w363 w435 w538 w561 w566]
      tunnel: [w19 w33 w38 w57 w63 w68 w72 w80 w86 w90 w94 w100 w111 w180 w185 w195 w199 w254 w316 w357 w400 w491 w539 w562 w567] -> w8
      tunnel: [_ _ _ _ _ TRUE _ _ _ _ _ _ _ _ _ _ _ _ _ _ _ _ _ _ _] -> w7
      tunnel: [w15 w31 w37 w56 w61 w67 w70 w79 w82 w88 w93 w99 w108 w178 w183 w193 w197 w201 w295 w349 w360 w432 w534 w560 w565] -> w6
      tunnel: w4 -> [w14 _ _ _ _ _ _ _ _ _ _ _ _ _ _ _ _ _ _ _ _ _ _ _ _]
      frame "", "Event Structure", "Idle" {
        # "executes when the state queue is empty"
        n5 = event shown="[0] 超时" {
          selector: _ -> [_ _]
          dyn-events: _ -> [_ _]
          timeout: w14 -> [_ _]
          tunnel: w20 -> [w24 w30]
          tunnel: [w23 w29] -> w19
          tunnel: w18 -> [w21 w27]
          tunnel: [w22 w28] -> w17
          tunnel: w16 -> [w22 w28]
          tunnel: [w21 w27] -> w15
          event Timeout {
            # "README FIRST\nThis VI template should be used by dragging & dropping it from the Functions palette onto the Block Diagram of a new, blank VI, which will place it's contents into the blank VI.\n\nDo not edit the VI found in the palette.  Only edit the state machine after it is placed into your blank VI.\n\nFor instructions on how to use the JKI State Machine, examples and video tutorials, visit:\nhttp://jki.net/state-machine/\n\nDELETE THIS NOTE AFTER READING"
            # "Timeout Frame\n(this will only execute if the Event Structure timeout is >= 0)"
            n6 = event-data() -> ()  [unwired: 1 in, 1 out]
            n7 = call <vilib>:"Add State(s) to Queue__jki_lib_state_machine.vi"("State(s) in (\"\")"=w24) -> ("States Out"=w23:string)  [unwired: 14 in]
          }
          event Panel Close? {
            # "Discard the event because we'll close the front panel ourselves in Macro: Exit"
            n8 = event-data() -> ()  [unwired: 1 in, 1 out]
            n9 = call <vilib>:"Add State(s) to Queue__jki_lib_state_machine.vi"("State(s) in Front (\"\")"="Macro: Exit", "State(s) in (\"\")"=w30) -> ("States Out"=w29:string)  [unwired: 13 in]
            n10 = event-data("Discard?"=FALSE) -> ()  [unwired: 1 in, 1 out]
          }
        }
      }
      frame "---------- Core ----------" {
        # "Do not put any code in this frame.\n(it is a separator no-op)"
        n11 = call <vilib>:"Add State(s) to Queue__JKI_lib_State_Machine.vi"("State(s) in (\"\")"=w34) -> ("States Out"=w33:string)  [unwired: 14 in]
      }
      frame Default {
        w44 = 42 items=["No error", "Argument error", "Memory is full", "Out of zone", "End of file", "File already open", "Generic file I/O error", "File not found", "File permission error", "Disk is full", "Duplicate path", "Too many files open", "System feature not enabled", "Resource file not found", "Cannot add resource", "Resource not found", "Image not found", "Image memory error", "Pen does not exist", "Config type invalid", "Config token not found", "Config parse error", "Config memory error", "Bad external code format", "Bad external code offset", "External code not present", "Null window", "Destroy window error", "Null menu", "Print aborted", "Bad print record", "Print driver error", "Windows error during printing", "Memory error during printing", "Print dialog error", "Generic print error", "Invalid device refnum", "Device not found", "Device parameter error", "Device unit error", "Cannot open device", "Device call aborted", "Generic error", "Cancelled by user", "Object ID too low", "Object ID too high", "Object not in heap", "Unknown heap", "Unknown object (invalid DefProc)", "Unknown object (DefProc not in table)", "Message out of range", "Invalid (null) method", "Unknown message", "Manager call not supported", "Bad address", "Network operation in progress", "Network operation timed out", "Connection is busy", "Network attribute not supported", "Network error", "Address in use", "System out of memory", "Connection aborted", "Connection refused", "Not connected", "Already connected", "Connection closed", "Initialization error (interapplication manager)", "Bad occurrence", "Wait on unbound occurrence handler", "Occurrence queue overflow", "Datalog type conflict", "Unused", "Unrecognized type (interapplication manager)", "Memory corrupt", "Failed to make temporary DLL", "Old CIN version", "Drag socket not found", "Failed to load drop-object", "Failed to register OLE object", "Failed to release OLE object", "Format specifier type mismatch", "Unknown format specifier", "Too few format specifiers", "Too many format specifiers", "Scan failed", "Newer CIN version", "Error converting to variant", "Runtime menu error", "Password tampered", "Variant attribute not found", "Incompatible variant data type", "Event data is not available", "Event Store is not present", "Occurrence is not found", "Event Queue is not created", "Event info is not available", "Refnum passed is NULL", "Error retrieving Class GUID", "Error retrieving CoClass GUID", "Error retrieving TypeLib GUID.", "Bad built application magic bytes.", "Specific driver is different from the specific driver associated with the Logical Name.", "There is no session opened to the class driver.", "Max Error", "MAX - Error with config objects", "MAX - Error loading configuration", "MAX - Group not supported"]
        # "Current State"
        # "Do not delete, rename, or modify this frame.\n(this is used to capture unhandled states and typos)"
        # "Handle mistyped state name (developer tool)"
        n12 = Format Into String(format string="Software Exception: Unhandled State \"%s\"." ("message"), error in=w40, w35) -> (resulting string=w43:string, error out=w42:errorcluster)  [unwired: 1 in]
        n13 = call <vilib>:"Error Cluster From Error Code.vi"("show call chain? (False)"=TRUE, "error in (no error)"=w42, "error message (\"\")"=w43, "error code (0)"=w44) -> ("error out"=w41:errorcluster)  [unwired: 5 in]
        n14 = call <vilib>:"Add State(s) to Queue__JKI_lib_State_Machine.vi"("State(s) in (\"\")"=w39) -> ("States Out"=w38:string)  [unwired: 14 in]
      }
      frame "Initialize Core Data" {
        # "Do not delete, rename, or modify this frame.\n(this is used to determine panel behavior on exit)"
        # "originally closed?"
        # "exe?"
        # "If panel starts closed or is an EXE, then close it when we exit"
        n15 = property class="VI"() -> ("FP.State"=w48:T46)  [unwired: 2 in, 2 out]
        n16 = property class="App"() -> ("App.Kind"=w54:T47)  [unwired: 2 in, 2 out]
        n17 = control-ref of="Current VI Reference"() -> (w49:refnum<vi>)
        n18 = Equal?(x=w48, y=T46."Closed" ("Front Panel Window:State")) -> (x = y?=w46:bool)
        n19 = Equal?(x=w54, y=T47."Run Time System" ("Application:Kind")) -> (x = y?=w52:bool)
        n20 = Or(x=w46, y=w52) -> (x .or. y?=w50:bool)
        n21 = Bundle By Name(cluster=w51, "Core.Current VI Reference"=w49, "Core.Close Panel on Exit?"=w50) -> (w56:T52)
        n22 = call <vilib>:"Add State(s) to Queue__JKI_lib_State_Machine.vi"("State(s) in (\"\")"=w58) -> ("States Out"=w57:string)  [unwired: 14 in]
      }
      frame "Error Handler" {
        # "Unhandled Error -- Display it"
        # "Handle any errors here.\nYou can also output any states to clean-up after errors occur"
        # "Clear error"
        n23 = call <vilib>:"General Error Handler.vi"("error in (no error)"=w60) -> ()  [unwired: 10 in, 5 out]
        n24 = call <vilib>:"Add State(s) to Queue__JKI_lib_State_Machine.vi"("State(s) in Front (\"\")"="/* Post Error States", "State(s) in (\"\")"=w64) -> ("States Out"=w63:string)  [unwired: 13 in]
      }
      frame "Exit" {
        # "Do not put any code in this frame.\n(No errors that occur here will be handled.)"
        n25 = call <vilib>:"Add State(s) to Queue__JKI_lib_State_Machine.vi"("State(s) in (\"\")"=w69) -> ("States Out"=w68:string)  [unwired: 14 in]
      }
      frame "---------- Data ----------" {
        # "Do not put any code in this frame.\n(It is a separator no-op. You can make a copy of this frame to create a new Data frame)"
        n26 = call <vilib>:"Add State(s) to Queue__JKI_lib_State_Machine.vi"("State(s) in (\"\")"=w73) -> ("States Out"=w72:string)  [unwired: 14 in]
      }
      frame "Data: Initialize" {
        w75 = T53 {"Current VI Reference"=refnum, "Close Panel on Exit?"=FALSE}  # Core
        w77 = TRUE  # Your Boolean data
        w76 = ""  # Your string data
        # "do not delete - used by framework"
        # "Add new data here."
        # "Initialize the shift-register data, here.\n(data names are defined by what you wire into the bundle function)"
        n27 = call <vilib>:"Add State(s) to Queue__jki_lib_state_machine.vi"("State(s) in (\"\")"=w81) -> ("States Out"=w80:string)  [unwired: 14 in]
        n28 = Bundle("Core"=w75, "Your Boolean data"=w77, "Your string data"=w76, "Main State Cluster"="Main State Cluster") -> (w79:T52)  [unwired: 1 in]
      }
      frame "Data: Cleanup" {
        # "Cleanup any data and references, here.\n(this is called automatically, by the Macro: Exit)"
        n29 = Unbundle By Name(w82) -> ("Core.Current VI Reference"=w85:refnum<vi>)
        n30 = Close Reference(reference=w85, error in (no error)=w84) -> (error out=w83:errorcluster)
        n31 = call <vilib>:"Add State(s) to Queue__jki_lib_state_machine.vi"("State(s) in (\"\")"=w87) -> ("States Out"=w86:string)  [unwired: 14 in]
      }
      frame "---------- UI ----------" {
        # "Do not put any code in this frame.\n(It is a separator no-op. You can make a copy of this frame to create a new UI frame)"
        n32 = call <vilib>:"Add State(s) to Queue__jki_lib_state_machine.vi"("State(s) in (\"\")"=w91) -> ("States Out"=w90:string)  [unwired: 14 in]
      }
      frame "UI: Initialize" {
        # "Initialize the User Interface, here.\n(this is called automatically, by the Macro: Init)"
        n33 = call <vilib>:"Add State(s) to Queue__jki_lib_state_machine.vi"("State(s) in (\"\")"=w95) -> ("States Out"=w94:string)  [unwired: 14 in]
      }
      frame "UI: Cursor Set" {
        # "Argument"
        # "Set and Unset Cursor Busy.\n(Usage: \"UI: Cursor Set >> Busy|Idle\")"
        n34 = case shown="\"Idle\", 默认" w96 {
          tunnel: w98 -> [w103 w105]
          tunnel: [w102 w104] -> w97
          frame "Idle", Default {
            n35 = call <vilib>:"Unset Busy.vi"("error in (no error)"=w103) -> ("error out"=w102:errorcluster)  [unwired: 10 in]
          }
          frame "Busy" {
            n36 = call <vilib>:"Set Busy.vi"("error in (no error)"=w105) -> ("error out"=w104:errorcluster)  [unwired: 9 in, 1 out]
          }
        }
        n37 = call <vilib>:"Add State(s) to Queue__jki_lib_state_machine.vi"("State(s) in (\"\")"=w101) -> ("States Out"=w100:string)  [unwired: 14 in]
      }
      frame "UI: Front Panel State" {
        # "Argument"
        # "Set Front Panel Open or Closed\n(Usage: \"UI: Front Panel State >> Open|Close\")"
        n38 = Unbundle By Name(w108) -> ("Core.Current VI Reference"=w107:refnum<vi>)
        n39 = case shown="\"Minimize\", \"Minimized\"" w106 {
          tunnel: w110 -> [w118 w133 w144 w157 w170]
          tunnel: [w120 w134 w146 w159 w172] -> w109
          tunnel: w107 -> [w119 w131 w145 w158 w171]
          frame "Open", "Standard", Default {
            w113 = T46."Standard" ("State")
            n40 = property class="VI"(reference=w119, error in=w118) -> (reference out=w116:refnum<vi>, error out=w117:errorcluster, "FP.State"=w115:T46)
            n41 = Not Equal?(x=w115, y=w113) -> (x != y?=w114:bool)
            n42 = case shown="真" w114 {
              tunnel: [w124 w126] -> w120
              tunnel: w117 -> [w123 w126]
              tunnel: w116 -> [w122 _]
              tunnel: w113 -> [w121 _]
              frame True {
                n43 = invoke class="VI" method="FP.Open"(reference=w122, error in=w123, "Activate"=TRUE, "State"=w121) -> (error out=w124:errorcluster)  [unwired: 1 in, 4 out]
              }
              frame False {
              }
            }
          }
          frame "Close", "Closed" {
            n44 = property class="VI"(reference=w131, error in=w133) -> (reference out=w130:refnum<vi>, error out=w132:errorcluster, "FP.State"=w128:T46)
            n45 = Not Equal?(x=w128, y=T46."Closed" ("Front Panel Window:State")) -> (x != y?=w127:bool)
            n46 = case shown="真" w127 {
              tunnel: [w135 w138] -> w134
              tunnel: w132 -> [w135 w137]
              tunnel: w130 -> [_ w136]
              frame False {
              }
              frame True {
                n47 = invoke class="VI" method="FP.Close"(reference=w136, error in=w137) -> (error out=w138:errorcluster)  [unwired: 1 in, 2 out]
              }
            }
          }
          frame "Hidden", "Hide" {
            w139 = T46."Hidden" ("State")
            n48 = property class="VI"(reference=w145, error in=w144) -> (reference out=w142:refnum<vi>, error out=w143:errorcluster, "FP.State"=w141:T46)
            n49 = Not Equal?(x=w141, y=w139) -> (x != y?=w140:bool)
            n50 = case shown="真" w140 {
              tunnel: [w150 w151] -> w146
              tunnel: w143 -> [w149 w151]
              tunnel: w142 -> [w148 _]
              tunnel: w139 -> [w147 _]
              frame True {
                n51 = invoke class="VI" method="FP.Open"(reference=w148, error in=w149, "State"=w147) -> (error out=w150:errorcluster)  [unwired: 2 in, 4 out]
              }
              frame False {
              }
            }
          }
          frame "Minimize", "Minimized" {
            w152 = T46."Minimized" ("State")
            n52 = property class="VI"(reference=w158, error in=w157) -> (reference out=w155:refnum<vi>, error out=w156:errorcluster, "FP.State"=w154:T46)
            n53 = Not Equal?(x=w154, y=w152) -> (x != y?=w153:bool)
            n54 = case shown="真" w153 {
              tunnel: [w163 w164] -> w159
              tunnel: w156 -> [w162 w164]
              tunnel: w155 -> [w161 _]
              tunnel: w152 -> [w160 _]
              frame True {
                n55 = invoke class="VI" method="FP.Open"(reference=w161, error in=w162, "State"=w160) -> (error out=w163:errorcluster)  [unwired: 2 in, 4 out]
              }
              frame False {
              }
            }
          }
          frame "Maximize", "Maximized" {
            w165 = T46."Maximized" ("State")
            n56 = property class="VI"(reference=w171, error in=w170) -> (reference out=w168:refnum<vi>, error out=w169:errorcluster, "FP.State"=w167:T46)
            n57 = Not Equal?(x=w167, y=w165) -> (x != y?=w166:bool)
            n58 = case shown="真" w166 {
              tunnel: [w176 w177] -> w172
              tunnel: w169 -> [w175 w177]
              tunnel: w168 -> [w174 _]
              tunnel: w165 -> [w173 _]
              frame True {
                n59 = invoke class="VI" method="FP.Open"(reference=w174, error in=w175, "State"=w173) -> (error out=w176:errorcluster)  [unwired: 2 in, 4 out]
              }
              frame False {
              }
            }
          }
        }
        n60 = call <vilib>:"Add State(s) to Queue__jki_lib_state_machine.vi"("State(s) in (\"\")"=w112) -> ("States Out"=w111:string)  [unwired: 14 in]
      }
      frame "---------- Macro ----------" {
        # "Do not put any code in this frame.\n(It is a separator no-op. You can make a copy of this frame to create a new Macro frame)"
        n61 = call <vilib>:"Add State(s) to Queue__jki_lib_state_machine.vi"("State(s) in (\"\")"=w181) -> ("States Out"=w180:string)  [unwired: 14 in]
      }
      frame "Macro: Initialize" {
        w182 = "Data: Initialize\nInitialize Core Data\nUI: Initialize\nUI: Front Panel State >> Open"  # Data: Initialize Initialize Core Data UI: Initialize UI: Front Panel State >> Open
        # "Initialization Macro\n(This is called once, when the VI starts)"
        n62 = call <vilib>:"Add State(s) to Queue__JKI_lib_State_Machine.vi"("State(s) in Front (\"\")"=w182, "State(s) in (\"\")"=w186) -> ("States Out"=w185:string)  [unwired: 13 in]
      }
      frame "Macro: Exit" {
        # "Exit Macro\n(This is called once, when the VI exits)"
        n63 = Unbundle By Name(w193) -> ("Core.Close Panel on Exit?"=w192:bool)
        n64 = Select(t="UI: Front Panel State >> Close", s=w192, f="") -> (s? t:f=w189:string)
        n65 = call <vilib>:"Add State(s) to Queue__JKI_lib_State_Machine.vi"("State(s) in (\"\")"=w189, "State(s) at Back (\"\")"="Data: Cleanup\nExit") -> ("States Out"=w187:string)  [unwired: 13 in]
        n66 = call <vilib>:"Add State(s) to Queue__JKI_lib_State_Machine.vi"("State(s) in Front (\"\")"=w187, "State(s) in (\"\")"=w196) -> ("States Out"=w195:string)  [unwired: 13 in]
      }
      frame "---------- Initialize ----------" {
        # "Template Separator\n(You can make a copy of, or modify, this frame)"
        n67 = call <vilib>:"Add State(s) to Queue__jki_lib_state_machine.vi"("State(s) in (\"\")"=w200) -> ("States Out"=w199:string)  [unwired: 14 in]
      }
      frame "Initialize: initPartment" {
        w210 = path "c:/Database"
        (unwired) 24 ("dimension size")
        (unwired) 175000 ("dimension size")
        w211 = sgl 14.0 ("element")
        (unwired) string[] ["Check Input"] ("event queue out")
        # "old"
        # "old"
        # "Your code here.\n(You can make a copy of, or modify, this frame)"
        n68 = Unbundle By Name(w204) -> ("Main State Cluster.ctl refs.all station status"=w242:refnum<vi>, "Main State Cluster.ctl refs.Individual Station Status"=w241:refnum<vi>, "Main State Cluster.misc station config.Station Name"=w230:string, "Main State Cluster.rs232 port map.PS Port"=w228:refnum<visa-resource-name>, "Main State Cluster.D out map.Comm Power"=w251:T8, "Main State Cluster.misc station config.power supply type"=w240:T23, "Main State Cluster.NVH Configuration"=w220:T6)  [unwired: 1 out]
        n69 = Unbundle By Name(w204) -> ("Main State Cluster.rs232 port map.RS232"=w213:refnum<visa-resource-name>)
        n70 = Empty String/Path?(string/path=w213) -> (empty?=w214:bool)
        n71 = Concatenate Strings(w230, "\\Excel Data\\" ("Audit")) -> (w234:string)
        n72 = Concatenate Strings(w230, "\\AP Data\\") -> (w233:string)
        n73 = Concatenate Strings(w230, "\\Current Data\\") -> (w232:string)
        n74 = Concatenate Strings(w230, "\\Sunshade Force Data\\") -> (w231:string)
        n75 = disable-structure shown="禁用" {
          disable-tunnel: w220 -> [w274 _]
          frame Disabled {
            n76 = Unbundle By Name(w274) -> ("NVH Station?"=w273:bool)
            n77 = case shown="真" w273 {
              tunnel: w274 -> [_ w275]
              frame False {
              }
              frame True {
                w276 = NVH_Mode_Control_2.0."Init" ("Mode")
                n78 = call "EOL NVH Inputs Controls Buffer 2.0.vi"("NVH Configuration"=w275, "Mode"=w276) -> ()  [unwired: 5 in, 5 out]
                n79 = call "EOL NVH Outputs Controls Buffer 2.0.vi"("Mode"=w276, "NVH Configuration"=w275) -> ()  [unwired: 8 in, 6 out]
              }
            }
          }
          frame Enabled {
          }
        }
        n80 = case shown="假" w214 {
          tunnel: w213 -> [w279 _]
          tunnel: w203 -> [w278 w280]
          tunnel: [w277 w280] -> w212
          frame False {
            n81 = call-poly "VISA Configure Serial Port"("VISA resource name"=w279, "error in (no error)"=w278) -> ("error out"=w277:errorcluster)  [unwired: 12 in, 1 out]
          }
          frame True {
          }
        }
        n82 = Concatenate Strings(w230, "\\Data Bytes Log\\" ("Audit")) -> (w229:string)
        n83 = property class="Clust (严格)"(reference=w241) -> (reference out=w243:refnum<vi>, error out=w246:errorcluster, "Value"=w245:T54)  [unwired: 1 in]
        n84 = property class="Clust (严格)"(reference=w242) -> (reference out=w250:refnum<vi>, error out=w247:errorcluster, "Value"=w248:T55)  [unwired: 1 in]
        n85 = Build Path(base path=w210, name or relative path=w234) -> (appended path=w227:path)
        n86 = Build Path(base path=w210, name or relative path=w233) -> (appended path=w225:path)
        n87 = Build Path(base path=w210, name or relative path=w232) -> (appended path=w224:path)
        n88 = Build Path(base path=w210, name or relative path=w231) -> (appended path=w223:path)
        n89 = Build Path(base path=w210, name or relative path=w229) -> (appended path=w222:path)
        n90 = Build Array(w210, w227, w225, w224, w223, w222) -> (w226:path[])
        n91 = Bundle By Name(cluster=w248, "Station Name"=w230) -> (w249:T55)
        n92 = Bundle By Name(cluster=w245, "Station"=w230) -> (w244:T54)
        n93 = call <vilib>:"Add State(s) to Queue__JKI_lib_State_Machine.vi"("State(s) in (\"\")"=w255) -> ("States Out"=w254:string)  [unwired: 14 in]
        n94 = for {
          shift-right: [w284] -> w221
          shift-left: w212 -> [w283]
          tunnel: w226 -> [w281] mode=indexing
          n95 = call <vilib>:"Check if File or Folder Exists.vi"("error in (no error)"=w283, "path"=w281) -> ("error out"=w282:errorcluster, "file or folder exists?"=w286:bool, "dup path"=w285:path)  [unwired: 7 in]
          n96 = case shown="真" w286 {
            tunnel: w285 -> [w288 w292]
            tunnel: [w288 w291] -> _
            tunnel: w282 -> [_ w290]
            tunnel: [errorcluster {"status"=FALSE, "code"=0, "source"=""} ("error out") w289] -> w284
            frame True {
            }
            frame False {
              n97 = Create Folder(path (use dialog)=w292, error in=w290) -> (created path=w291:path, error out=w289:errorcluster)  [unwired: 1 in, 1 out]
            }
          }
        }
        n98 = property class="Clust (严格)"(reference=w243, error in=w246, "Value"=w244) -> ()  [unwired: 2 out]
        n99 = property class="Clust (严格)"(reference=w250, error in=w247, "Value"=w249) -> ()  [unwired: 2 out]
        n100 = Initialize Array(sgl 0.0 ("element"), 350000 ("dimension size"), 8 ("dimension size")) -> (w215:sgl[][])
        n101 = Bundle By Name(cluster=T48 {"Status"=FALSE, "Global DO Ch"=enum."Battery"} ("Cluster"), "Status"=TRUE, "Global DO Ch"=w251) -> (w206:T48)
        n102 = Bundle By Name(cluster=w204, "Main State Cluster.paths.Base Path"=path "C:/Labview Code", "Main State Cluster.Application Status"="Init" ("Application Status"), "Main State Cluster.misc status.Serial Port Configured?"=FALSE ("Serial Port Configured?"), "Main State Cluster.Motion Status.Motion"=All_Motions."Idle" ("Current Motion"), "Main State Cluster.Motion Status.Analog Data"=w215, "Main State Cluster.misc status.PS Voltage"=w211) -> (w201:T52)
        n103 = Build Array(w206) -> (w205:T48[])
        n104 = disable-structure shown="启用" {
          disable-tunnel: [w265 _] -> w202
          disable-tunnel: w240 -> [w264 _]
          disable-tunnel: w228 -> [w263 _]
          disable-tunnel: w221 -> [w262 _]
          disable-tunnel: w211 -> [w261 _]
          disable-tunnel: w205 -> [w259 _]
          frame Enabled {
            n105 = Empty String/Path?(string/path=w263) -> (empty?=w256:bool)
            n106 = case shown="假" w256 {
              tunnel: [w271 w272] -> w257
              tunnel: w263 -> [w270 _]
              tunnel: 1 ("No. of Power Supplies") -> [w269 _]
              tunnel: w264 -> [w268 _]
              tunnel: w262 -> [w267 w272]
              tunnel: w261 -> [w266 _]
              frame False {
                n107 = call "EOL Initialize Power Supplies.vi"("Volt Limit"=w266, "Error In"=w267, "power supply model"=w268, "No. of Power Supplies"=w269, "VISA resource name"=w270) -> ("error out"=w271:errorcluster)  [unwired: 6 in]
              }
              frame True {
              }
            }
            n108 = call "EOL Digital Outputs v3.vi"("Error In"=w257, "DO Status"=w259, "Mode"=T49."Write") -> ("Error Out"=w265:errorcluster)  [unwired: 7 in, 1 out]
          }
          frame Disabled {
          }
        }
      }
      frame "Initialize: initComPort" {
        w300 = 14.5 ("Volt Limit")
        # "Your code here.\n(You can make a copy of, or modify, this frame)"
        n109 = Unbundle By Name(w296) -> ("Main State Cluster"=w299:T1)
        n110 = Unbundle By Name(w299) -> ("ctl refs.Individual Station Status"=w303:refnum<vi>, "rs232 port map.RS232"=w312:refnum<visa-resource-name>, "Store Data.Error Table"=w313:string[][], "rs232 port map.PMAC"=w311:refnum<visa-resource-name>, "D out map.Comm Power"=w301:T8)  [unwired: 1 out]
        n111 = flat-sequence {
          tunnel: w301 -> [w320]
          tunnel: w298 -> [w319]
          tunnel: [w318] -> w315
          tunnel: [w326] -> w308
          tunnel: w315 -> [w326]
          frame #0 {
            n112 = Bundle By Name(cluster=T48 {"Status"=FALSE, "Global DO Ch"=enum."Battery"} ("Cluster"), "Status"=TRUE, "Global DO Ch"=w320) -> (w324:T48)
            n113 = Build Array(w324) -> (w323:T48[])
            n114 = call "EOL Digital Outputs v3.vi"("Error In"=w319, "DO Status"=w323, "Mode"=T49."Write") -> ("Error Out"=w318:errorcluster)  [unwired: 7 in, 1 out]
          }
          frame #1 {
            n115 = Wait (ms)(milliseconds to wait=u32 500) -> ()  [unwired: 1 out]
          }
        }
        n116 = Empty String/Path?(string/path=w311) -> (empty?=w310:bool)
        n117 = case shown="假" w310 {
          tunnel: w311 -> [w332 w335]
          tunnel: [w331 w335] -> w309
          tunnel: w308 -> [w330 w334]
          tunnel: [w328 w334] -> w293
          frame False {
            n118 = call-poly "VISA Configure Serial Port"("VISA resource name"=w332, "error in (no error)"=w330) -> ("VISA resource name out"=w333:refnum<visa-resource-name>, "error out"=w329:errorcluster)  [unwired: 12 in]
            n119 = VISA Flush I/O Buffer(VISA resource name=w333, error in (no error)=w329) -> (VISA resource name out=w331:refnum<visa-resource-name>, error out=w328:errorcluster)  [unwired: 1 in]
          }
          frame True {
          }
        }
        n120 = call <vilib>:"Add State(s) to Queue__JKI_lib_State_Machine.vi"("State(s) in (\"\")"=w317) -> ("States Out"=w316:string)  [unwired: 14 in]
        n121 = case shown="错误" w293 {
          selector: w293 -> [w336 w340]
          tunnel: [w338 w343] -> w314
          tunnel: w312 -> [_ w346]
          tunnel: w313 -> [w338 w345]
          tunnel: [TRUE FALSE] -> w302
          tunnel: [w336 w339] -> w297
          frame No Error {
          }
          frame Error {
            n122 = Format Into String(initial string="", w346) -> (resulting string=w341:string)  [unwired: 2 in, 1 out]
            n123 = call "EOL Error Table.vi"("Error Description"=w341, "error in"=w340, "Error No."=u16 11, "Error Table In"=w345) -> ("error out"=w339:errorcluster, "Error Table Out"=w343:string[][])  [unwired: 6 in]
          }
        }
        n124 = property class="Clust (严格)"(reference=w303) -> (reference out=w307:refnum<vi>, error out=w304:errorcluster, "Value"=w305:T54)  [unwired: 1 in]
        n125 = Bundle By Name(cluster=w305, "Serial Port"=w302, "Glass Voltage"=w300) -> (w306:T54)
        n126 = Bundle By Name(cluster=w299, "misc status.Serial Port Configured?"=w302, "Store Data.Error Table"=w314, "misc status.Diag Serial Port"=w312, "rs232 port map.PMAC"=w309, "misc status.PS Voltage"=w300) -> (w294:T1)
        n127 = property class="Clust (严格)"(reference=w307, error in=w304, "Value"=w306) -> ()  [unwired: 2 out]
        n128 = Bundle By Name(cluster=w296, "Main State Cluster"=w294) -> (w295:T52)
      }
      frame "Initialize: initContral" {
        w350 = T56 {"Noise Test"=enum."Not Tested", "Avg Current"=0.0, "Run Time"=0.0, "Speed"=0.0, "Position"=enum."Not Tested"}
        # "Template Separator\n(You can make a copy of, or modify, this frame)"
        n129 = Unbundle By Name(w349) -> ("Main State Cluster"=w348:T1)
        n130 = Unbundle By Name(w348) -> ("ctl refs.Motion Data"=w351:refnum<vi>)
        n131 = property class="Clust (严格)"(reference=w351) -> (reference out=w355:refnum<vi>, error out=w352:errorcluster, "Value"=w353:T57)  [unwired: 1 in]
        n132 = Bundle By Name(cluster=w353, "Shade Close Limits"=w350, "Shade Close Data 2"=w350, "Shade Open Limits"=w350, "Shade Open Data"=w350, "Vent Close Limits"=w350, "Vent Close Data"=w350, "Vent Open Limits"=w350, "Vent Open Data"=w350, "Slide Close Limits"=w350, "Slide Close Data"=w350, "Slide Open Limits"=w350, "Slide Open Data"=w350) -> (w354:T57)
        n133 = property class="Clust (严格)"(reference=w355, error in=w352, "Value"=w354) -> ()  [unwired: 2 out]
        n134 = call <vilib>:"Add State(s) to Queue__jki_lib_state_machine.vi"("State(s) in (\"\")"=w358) -> ("States Out"=w357:string)  [unwired: 14 in]
      }
      frame "Initialize: initMotion" {
        w395 = Pass_Fail_Control."Not Tested"  # Position Test
        w396 = Pass_Fail_Control."Not Tested"  # Noise Test
        w398 = 0 ("Current Data Index")
        # "Template Separator\n(You can make a copy of, or modify, this frame)"
        n135 = Unbundle By Name(w361) -> ("Main State Cluster"=w364:T1)
        n136 = Unbundle By Name(w364) -> ("noSCU Paremeter.set position"=w370:i32[], "misc status.AP Data Type"=w376:T16, "misc status.Serial Port Configured?"=w385:bool, "misc status.PS Voltage"=w392:dbl, "Sequence State.Step Data String"=w397:string, "Motion Status.Analog Data"=w389:sgl[][], "Store Data.Motion Data Array"=w380:T14[], "Motion Status.Motion"=w374:T3, "misc status.Part Setup.Communication Type"=w372:T39, "noSCU Paremeter.Derect control"=w365:bool, "manual control(direct)"=w366:bool)
        n137 = call "Inalfa SCU LIN Message to Move.vi"("Communication Type"=w372, "Motion"=w374) -> ("Have Swtich?"=w368:bool)  [unwired: 9 in]
        n138 = Empty String/Path?(string/path=w397) -> (empty?=w373:bool)
        n139 = Compound Arithmetic op=AND ("复合运算")(w368, invert w365) -> (w367:bool)
        n140 = Compound Arithmetic op=OR ("复合运算")(w366, w373, w367) -> (w371:bool)
        n141 = Array Size(array=w389) -> (size(s)=w388:i32[])
        n142 = case shown="假" w371 {
          tunnel: T15 {"Power Supply Voltage"=13.0, "Min Avg Current"=0.0, "Max Avg Current"=0.0, "Min Run Time"=0.0, "Max Run Time"=0.0, "Min Speed"=0.0, "Max Speed"=0.0, "AP Data % of Threshold"=0.0, "Travel Distance"=0.0, "AP Data Type"=enum."91/61", "Check Current"=FALSE, "Check Run Time"=FALSE, "Check Speed"=FALSE, "Express Motion?"=FALSE, "Check Sound Test"=FALSE, "Check Position?"=FALSE, "Collect AP Data"=FALSE, "Inital Position"=0, "End Position"=0, "Goto Posiition"=0, "Max max Current"=0.0, "Min max Current"=0.0, "Check max Current"=FALSE, "Check Sound"=FALSE, "Min Sound (dB)"=0.0, "Max Sound (dB)"=0.0} ("Motion Data Cluster") -> [w423 w429]
          tunnel: [w412 w428] -> w384
          tunnel: w397 -> [w419 _]
          tunnel: [w422 w427] -> w378
          tunnel: w392 -> [_ w427]
          tunnel: w363 -> [w421 w426]
          tunnel: [w420 w426] -> w362
          tunnel: w385 -> [_ _]
          tunnel: [w416 w425] -> w377
          tunnel: w376 -> [_ w425]
          tunnel: [w411 w424] -> w369
          tunnel: w370 -> [_ w424]
          frame False {
            n143 = Unflatten From String(type=w423, binary string=w419, error in (no error)=w421) -> (value=w417:T15, error out=w418:errorcluster)  [unwired: 2 in, 1 out]
            n144 = call "convert motion step with u8 positions to u16.vi"("error in"=w418, "data string"=w419, "Motion Data Cluster in"=w417) -> ("error out"=w420:errorcluster, "Motion Data Cluster out"=w412:T15)  [unwired: 7 in]
            n145 = Unbundle By Name(w412) -> ("Inital Position"=w415:u16, "End Position"=w414:u16, "Goto Posiition"=w413:u16)
            n146 = Unbundle By Name(w412) -> ("Power Supply Voltage"=w422:dbl, "AP Data Type"=w416:T16)
            n147 = Build Array(w415, w414, w413) -> (w411:u16[])
          }
          frame True {
            n148 = Bundle By Name(cluster=w429, "Power Supply Voltage"=w427, "AP Data Type"=w425) -> (w428:T15)
          }
        }
        n149 = Index Array(array=w388) -> (element #1=w387:i32, element #2=w386:i32)  [unwired: 2 in]
        n150 = for {
          N: w387 -> [_]
          shift-right: [w404] -> w390
          shift-left: w389 -> [w405]
          tunnel: w386 -> [w403]
          i -> [w402]
          n151 = for {
            N: w403 -> [_]
            shift-right: [w408] -> w404
            shift-left: w405 -> [w409]
            tunnel: w402 -> [w407]
            i -> [w406]
            n152 = in-place {
              n153 = in-place-array #1(w409, w407, w406) -> ()  [unwired: 1 out]
              n154 = in-place-array #1(sgl 0.0 ("element")) -> (w408:sgl[][])  [unwired: 2 out]
            }
          }
        }
        n155 = Initialize Array(0.0 ("element"), 8 ("dimension size")) -> (w383:dbl[])
        n156 = Bundle By Name(cluster=T14 {"Motion"=enum."Glass Teach", "Actual Avg Current"=0.0, "Actual Runtime"=0.0, "Actual Speed"=0.0, "Current Data"=[], "Motion Data Limits"={"Power Supply Voltage"=0.0, "Min Avg Current"=0.0, "Max Avg Current"=0.0, "Min Run Time"=0.0, "Max Run Time"=0.0, "Min Speed"=0.0, "Max Speed"=0.0, "AP Data % of Threshold"=10.0, "Travel Distance"=0.0, "AP Data Type"=enum."91/61", "Check Current"=FALSE, "Check Run Time"=FALSE, "Check Speed"=FALSE, "Express Motion?"=FALSE, "Check Sound Test"=FALSE, "Check Position?"=FALSE, "Collect AP Data"=FALSE, "Inital Position"=0, "End Position"=0, "Goto Posiition"=0, "Max max Current"=0.0, "Min max Current"=0.0, "Check max Current"=FALSE, "Check Sound"=FALSE, "Min Sound (dB)"=0.0, "Max Sound (dB)"=0.0}, "Switch 1 to 6"=[], "Actual PS Voltage"=0.0, "AP Data"=[], "Actual max Current"=0.0, "Actual Noise (dB)"=0.0} ("Motion Data"), "Motion Data Limits"=w384, "Switch 1 to 6"=w383, "Motion"=w374) -> (w381:T14)
        n157 = Build Array (concatenate)(w380, w381) -> (w379:T14[])
        n158 = Bundle By Name(cluster=w364, "noSCU Paremeter.set position"=w369, "misc status.AP Data Type"=w377, "misc status.PS Voltage"=w378, "Motion Status.Current Data Index"=w398, "Motion Status.Messages Index"=w398, "Motion Status.Analog Data"=w390, "Motion Status.Noise Test"=w396, "Motion Status.Position Test"=w395, "Motion Status.motion stop check initialized"=FALSE ("motion stop check initialized"), "Store Data.Motion Data Array"=w379, "Decibel data"=dbl[] []) -> (w359:T1)
        n159 = Bundle By Name(cluster=w361, "Main State Cluster"=w359) -> (w360:T52)
        n160 = call <vilib>:"Add State(s) to Queue__jki_lib_state_machine.vi"("State(s) in (\"\")"=w401) -> ("States Out"=w400:string)  [unwired: 14 in]
      }
      frame "Initialize: initTest" {
        w437 = FALSE ("Operator Action?")
        w451 = TRUE ("NVH Operator?")
        w485 = FALSE ("Ext Diag Mode?")
        w488 = TRUE ("Cycling?")
        w486 = u8 0 ("Motion Index")
        # "Template Separator\n(You can make a copy of, or modify, this frame)"
        n161 = Unbundle By Name(w433) -> ("Main State Cluster"=w436:T1)
        n162 = Unbundle By Name(w436) -> ("ctl refs.Route to Repair"=w438:refnum<vi>, "ctl refs.Red-Rabbit Mode"=w456:refnum<vi>, "Motion Status.Analog Data"=w459:sgl[][], "ctl refs.Individual Station Status"=w439:refnum<vi>, "ctl refs.all station status"=w472:refnum<vi>, "PLC Comms.PLC bool write Tags.Test Started"=w482:T26, "PLC Comms.PLC bool write Tags.Retract LVDT's"=w481:T26, "PLC Comms.PLC bool write Tags.Extend LVDT's"=w480:T26, "PLC Comms.PLC bool write Tags.AT set wand home pos"=w466:T26, "PLC Comms.PLC bool write Tags.Test Complete Pass"=w464:T26, "PLC Comms.PLC bool write Tags.Test Complete Fail"=w463:T26, "PLC Comms.PLC bool write Tags.NVH Operator Pass"=w449:T26, "PLC Comms.PLC bool write Tags.NVH Operator Fail"=w448:T26, "PLC Comms.PLC bool write Tags.NVH Operator Check"=w447:T26, "PLC Comms.PLC bool write Tags.NVH Operator Vent Open Noise"=w446:T26, "PLC Comms.PLC bool write Tags.NVH Operator Vent Close Noise"=w445:T26, "PLC Comms.PLC bool write Tags.NVH Operator Sunshade Open Noise"=w444:T26, "PLC Comms.PLC bool write Tags.NVH Operator Sunshade Close Noise"=w443:T26, "PLC Comms.PLC bool write Tags.NVH Operator Glass Open Noise"=w442:T26, "PLC Comms.PLC bool write Tags.NVH Operator Glass Close Noise"=w441:T26, "PLC Comms.PLC bool write Tags.NVH Operator Finish"=w440:T26)  [unwired: 1 out]
        n163 = Array Size(array=w459) -> (size(s)=w462:i32[])
        n164 = Build Array(w464, w463, w482, w481, w480, w466, w449, w448, w447, w446, w445, w444, w443, w442, w441, w440) -> (w479:T26[])
        n165 = property class="Clust (严格)"(reference=w472) -> (reference out=w476:refnum<vi>, error out=w473:errorcluster, "Value"=w474:T55)  [unwired: 1 in]
        n166 = Bundle By Name(cluster=w474, "Error Table Br"=string[][] [] ("Error Table Au"), "Pass / Fail"=u32 13816530 ("Pass/Fail AU"), "NVH System"=FALSE ("B&K System"), "Database LVDT's Data Out"=T50[] []) -> (w475:T55)
        n167 = Index Array(array=w462) -> (element #1=w461:i32, element #2=w460:i32)  [unwired: 2 in]
        n168 = disable-structure shown="启用" {
          disable-tunnel: w435 -> [w500 _]
          disable-tunnel: w479 -> [w499 _]
          disable-tunnel: bool[] [FALSE, FALSE, TRUE, FALSE, FALSE, TRUE, FALSE, FALSE, FALSE, FALSE, FALSE, FALSE, FALSE, FALSE, FALSE, FALSE] -> [w498 _]
          disable-tunnel: [w494 _] -> w434
          disable-tunnel: w466 -> [w493 _]
          frame Enabled {
            n169 = for {
              tunnel: w499 -> [w512] mode=indexing
              shift-right: [w515] -> w495
              shift-left: w500 -> [w516]
              tunnel: w498 -> [w511] mode=indexing
              n170 = Unbundle By Name(w512) -> ("Tag Name"=w513:string)
              n171 = Wait Until Next ms Multiple(millisecond multiple=u32 10 ("milliseconds to wait")) -> ()  [unwired: 1 out]
              n172 = Empty String/Path?(string/path=w513) -> (empty?=w514:bool)
              n173 = case shown="假" w514 {
                tunnel: w516 -> [w519 w521]
                tunnel: w513 -> [_ _]
                tunnel: [w520 w521] -> w515
                tunnel: w512 -> [w518 _]
                tunnel: w511 -> [w517 _]
                frame False {
                  n174 = call "plc write bool.vi"("error in"=w519, "value"=w517, "addr,tag"=w518) -> ("error out"=w520:errorcluster)  [unwired: 8 in]
                }
                frame True {
                }
              }
            }
            n175 = Unbundle By Name(w493) -> ("Tag Name"=w497:string)
            n176 = Empty String/Path?(string/path=w497) -> (empty?=w496:bool)
            n177 = case shown="真" w496 {
              tunnel: w495 -> [w505 w509]
              tunnel: [w504 w509] -> w494
              tunnel: w493 -> [w501 _]
              frame False {
                n178 = flat-sequence {
                  tunnel: [w506] -> w503
                  tunnel: w505 -> [w506]
                  frame #0 {
                    n179 = Wait (ms)(milliseconds to wait=u32 1000) -> ()  [unwired: 1 out]
                  }
                }
                n180 = call "plc write bool.vi"("error in"=w503, "value"=FALSE, "addr,tag"=w501) -> ("error out"=w504:errorcluster)  [unwired: 8 in]
              }
              frame True {
                # "delay to give plc\nchance to reset\nabort discrete signal"
                n181 = Wait (ms)(milliseconds to wait=u32 100) -> ()  [unwired: 1 out]
              }
            }
          }
          frame Disabled {
          }
        }
        n182 = for {
          N: w461 -> [_]
          shift-right: [w524] -> w458
          shift-left: w459 -> [w525]
          tunnel: w460 -> [w523]
          i -> [w522]
          n183 = for {
            N: w523 -> [_]
            shift-right: [w528] -> w524
            shift-left: w525 -> [w529]
            tunnel: w522 -> [w527]
            i -> [w526]
            n184 = in-place {
              n185 = in-place-array #2(w529, w527, w526) -> ()  [unwired: 1 out]
              n186 = in-place-array #2(sgl 0.0 ("element")) -> (w528:sgl[][])  [unwired: 2 out]
            }
          }
        }
        n187 = property class="Clust (严格)"(reference=w439) -> (error out=w457:errorcluster, "Value"=w468:T54)  [unwired: 1 in, 1 out]
        n188 = property class="Clust (严格)"(reference=w476, error in=w473, "Value"=w475) -> ()  [unwired: 2 out]
        n189 = Unbundle By Name(w468) -> ("Line Number"=w467:u8)
        n190 = property class="Bool (严格)"(reference=w456, error in=w457) -> (error out=w454:errorcluster, "Value"=w455:bool)  [unwired: 1 out]
        n191 = property on="Property Node" class="Bool (严格)"(reference=w438, error in=w454) -> ("Value"=w453:bool)  [unwired: 2 out]
        n192 = call "EOL All-Station Module Test Data Buffer.vi"() -> ("Store Data out"=w477:T13)  [unwired: 11 in]
        n193 = Tick Count (ms)() -> (millisecond timer value=w484:u32)
        n194 = Bundle By Name(cluster=w436, "Operator Pass?"=w451, "NVH Pass?"=w451, "NVH Operator?"=w451, "Sequence State.NVH Status.Restart IRQ Counter"=w486, "Sequence State.Active Step"=w486, "Application Status"="Test Started", "Motion Status.Motion"=All_Motions."Idle" ("Current Motion"), "Sequence State.Testing?"=w488, "Sequence State.Pass?"=w488, "misc status.Diag Mode?"=w485, "misc status.In Vehicle Mode?"=w485, "Sequence State.NVH Status.NVH Test Needed?"=w485, "Store Data.Error Table"=string[][] [] ("Error Table"), "Motion Status.Analog Data"=w458, "Sequence State.Cycle Start Time"=w484, "Sequence State.Red-Rabbit Mode"=w455, "misc status.Plant Number"=w467, "AP Test Data.Database AP Data"=dbl[] [0.0, 0.0, 0.0, 50.0, 0.0, 0.0, 0.0, 0.0, 0.0] ("Database AP Data"), "Store Data"=w477, "Sequence State.route-to-repair mode"=w453, "Motion Status.Current Hall Position"=i16 0, "Store Data.data bytes log"="", "Operator Action?"=w437, "Noise Source"=u32 0, "Second Check?"=w437, "noSCU Paremeter.teach pass"=w437) -> (w431:T1)
        n195 = Bundle By Name(cluster=w433, "Main State Cluster"=w431) -> (w432:T52)
        n196 = call <vilib>:"Add State(s) to Queue__jki_lib_state_machine.vi"("State(s) in (\"\")"=w492) -> ("States Out"=w491:string)  [unwired: 14 in]
      }
      frame "Initialize: initNVH" {
        # "Template Separator\n(You can make a copy of, or modify, this frame)"
        n197 = Unbundle By Name(w534) -> ("Main State Cluster"=w533:T1)
        n198 = Unbundle By Name(w533) -> ("ctl refs.all station status"=w536:refnum<vi>, "NVH Configuration.NVH Station?"=w537:bool, "NVH Configuration"=w535:T6)
        n199 = case shown="真" w537 {
          tunnel: [w541 w553] -> _
          tunnel: w533 -> [w541 w552]
          tunnel: w536 -> [_ w547]
          tunnel: w535 -> [_ w545]
          tunnel: [w540 w542] -> w532
          tunnel: w531 -> [w540 _]
          frame False {
          }
          frame True {
            w558 = T59[] [enum."Online", enum."Ready for Model"] items=["Online", "Pass", "Fail", "Testing", "Ready for Model", "Error Bit 1", "Error Bit 2", "Error Bit 3", "Failure Bit 1", "Failure Bit 2", "Failure Bit 3", "Failure Bit 4", "Echo Bit 1", "Echo Bit 2", "Echo Bit 3", "Echo Bit 4", "Serial Number Read Ok", "Ready for Serrial Number"] ("B&K Inputs Control")
            w546 = TRUE ("NVH Test Running?")
            n200 = property class="Clust (严格)"(reference=w547) -> (reference out=w551:refnum<vi>, error out=w548:errorcluster, "Value"=w549:T55)  [unwired: 1 in]
            n201 = Bundle By Name(cluster=w549, "NVH System"=w546) -> (w550:T55)
            n202 = Bundle By Name(cluster=w552, "Sequence State.NVH Status.NVH Test Running?"=w546) -> (w553:T1)
            n203 = call "EOL NVH Inputs Controls Buffer 2.0.vi"("NVH Configuration"=w545, "NVHK Inputs Control"=w558, "Mode"=NVH_Mode_Control_2.0."Read") -> ("NVH Inputs Out"=w554:bool[])  [unwired: 4 in, 4 out]
            n204 = Index Array(array=w554) -> (element #1=w557:bool, element #2=w556:bool)  [unwired: 2 in]
            n205 = Compound Arithmetic op=AND(w557, invert w556) -> (w555:bool)
            n206 = property class="Clust (严格)"(reference=w551, error in=w548, "Value"=w550) -> ()  [unwired: 2 out]
            n207 = Select(t="NVH Check Echo", s=w555, f="NVH Restart IRQ") -> (s? t:f=w542:string)
          }
        }
        n208 = call <vilib>:"Add State(s) to Queue__jki_lib_state_machine.vi"("State(s) in Front (\"\")"=w532, "State(s) in (\"\")"=w531) -> ("States Out"=w539:string)  [unwired: 13 in]
      }
      frame "---------- MyLoop ----------" {
        # "Template Separator\n(You can make a copy of, or modify, this frame)"
        n209 = call <vilib>:"Add State(s) to Queue__jki_lib_state_machine.vi"("State(s) in (\"\")"=w563) -> ("States Out"=w562:string)  [unwired: 14 in]
      }
      frame "MyLoop: 1234" {
        # "Template Separator\n(You can make a copy of, or modify, this frame)"
        n210 = Unbundle By Name(w565) -> ("Main State Cluster.Station Count"=→"Main State Cluster.Station Count":i32)
        n211 = call <vilib>:"Add State(s) to Queue__jki_lib_state_machine.vi"("State(s) in (\"\")"=w568) -> ("States Out"=w567:string)  [unwired: 14 in]
      }
    }
  }
